vi "PrefDialog-2.vi"(8 "error in (no error)":errorcluster, 11 "MyPluginsBase in":refnum<class "NHRGridSim.lvclass">) -> (0 "error out":errorcluster, 1 "Save As":bool, 2 "Changed":bool, 3 "MyPluginsBase out":refnum<class "NHRGridSim.lvclass">)   [LabVIEW 2018, in "AcPwrPlugins.lvlib" / "NHRGridSim.lvclass"]
doc: "This VI opens up the modal preference dialog window and allows a user to configure the properties with new values, or keep the existing values from the last time the function was called. The user can also save the new values to a new file name and new type name using the save as button."
uses:
  NHRGridSim.lvclass
  C:/Program Files (x86)/National Instruments/LabVIEW 2018/user.lib/NIST/BaseClasses/BasePlugin_class/BasePlugin.lvclass
  C:/Users/Public/Projects/ICDAS/NistPluggableModules/AcPwr/AcPwrPlugins/AcPwrBaseClass/AcPwrBase.lvclass
  PublicMethods/Measurements.ctl
  TypeDefs/MeasurementType.ctl
  TypeDefs/NHRGrid_Modes.ctl
  TypeDefs/Device(s)Settings.ctl
  TypeDefs/NHRGrid_InstrumentCluster_Tabs.ctl
  TypeDefs/NHRGrid_Configure_Tabs.ctl
  TypeDefs/NHRGrid_Ranges_Tabs.ctl
  TypeDefs/NHRGrid_SafetyTrips_Tabs.ctl
  TypeDefs/NHRGrid_SlewRates_Tabs.ctl
  TypeDefs/NHRGrid_Phases_Tabs.ctl
  <userlib>/NIST/BaseClasses/BasePlugin_class/BasePlugin.lvclass/BasePlugin.ctl
  AcPwrBaseClass/AcPwrBase.lvclass/AcPwrBase.ctl
  TypeDefs/NHRGrid_UpdateSettings.ctl
  TypeDefs/NHRGrid_ModeAdjust_Tabs.ctl
  <userlib>/NIST/BaseClasses/BasePlugin_class/Accessors/Read PluginIniFilePath.vi
  AcPwrBaseClass/Accessors/Read BaseConfig.vi
  AcPwrBaseClass/Accessors/Read BaseMeasurements.vi
  <userlib>/NIST/BaseClasses/BasePlugin_class/Accessors/Write PluginIniFilePath.vi
  <vilib>/Utility/config.llb/NI_LVConfig.lvlib
panel:
  in  "ModeVal":u8
  in  "ChassisTxt":string
  in  "Update":bool
  in  "Device(s)Settings":T1={"MeasName"="", "Instr1"={"Name"="", "Vout (V)"=0.0, "VType"="", "FreqOut (Hz)"=60.0, "Aperture (cycles)"=1, "Synchronization"=0, "Ranges"={"Voltage (V)"=0, "Current (A)"=1}, "Safety Trips"={"Vmin (V)"=0.0, "Vmin Time (s)"=-1.0, "Vmax (V)"=0.0, "Vmax Time (s)"=-1.0, "Imax Source (A)"=0.0, "I Src Time (s)"=-1.0, "Imax Sink (A)"=0.0, "I Snk Time (s)"=-1.0, "Pmax Source (W)"=0.0, "P Src Time (s)"=-1.0, "Pmax Sink (W)"=0.0, "P Snk Time (s)"=-1.0, "Abs Volt Peak"=0.0, "Enable Vpk"=FALSE, "Abs Curr Peak"=0.0, "Enable Ipk"=FALSE}, "Slew Rates"={"Voltage (V/s)"=866030.0, "Current (A/s)"=100000.0, "Power (W/s)"=3000000.0, "Frequency (Hz/s)"=500.0, "Phase Angle (Deg/s)"=50000.0}, "Phases"={"A-Volts (V)"=0.0, "B-Volts (V)"=0.0, "C-Volts (V)"=0.0, "A-Change at..."=0, "B-Angle (Deg)"=240, "C-Angle (Deg)"=120, "B-Change at..."=0, "C-Change at..."=0, "AngleTxt"="", "A-Wave Shape"=0, "B-Wave Shape"=0, "C-Wave Shape"=0}}, "Instr2"={"Name"="", "Vout (V)"=0.0, "VType"="", "FreqOut (Hz)"=60.0, "Aperture (cycles)"=1, "Synchronization"=0, "Ranges"={"Voltage (V)"=0, "Current (A)"=1}, "Safety Trips"={"Vmin (V)"=0.0, "Vmin Time (s)"=-1.0, "Vmax (V)"=0.0, "Vmax Time (s)"=-1.0, "Imax Source (A)"=0.0, "I Src Time (s)"=-1.0, "Imax Sink (A)"=0.0, "I Snk Time (s)"=-1.0, "Pmax Source (W)"=0.0, "P Src Time (s)"=-1.0, "Pmax Sink (W)"=0.0, "P Snk Time (s)"=-1.0, "Abs Volt Peak"=0.0, "Enable Vpk"=FALSE, "Abs Curr Peak"=0.0, "Enable Ipk"=FALSE}, "Slew Rates"={"Voltage (V/s)"=866030.0, "Current (A/s)"=100000.0, "Power (W/s)"=3000000.0, "Frequency (Hz/s)"=500.0, "Phase Angle (Deg/s)"=50000.0}, "Phases"={"A-Volts (V)"=0.0, "B-Volts (V)"=0.0, "C-Volts (V)"=0.0, "A-Change at..."=0, "B-Angle (Deg)"=240, "C-Angle (Deg)"=120, "B-Change at..."=0, "C-Change at..."=0, "AngleTxt"="", "A-Wave Shape"=0, "B-Wave Shape"=0, "C-Wave Shape"=0}}, "Instr3"={"Name"="", "Vout (V)"=0.0, "VType"="", "FreqOut (Hz)"=60.0, "Aperture (cycles)"=1, "Synchronization"=0, "Ranges"={"Voltage (V)"=0, "Current (A)"=1}, "Safety Trips"={"Vmin (V)"=0.0, "Vmin Time (s)"=-1.0, "Vmax (V)"=0.0, "Vmax Time (s)"=-1.0, "Imax Source (A)"=0.0, "I Src Time (s)"=-1.0, "Imax Sink (A)"=0.0, "I Snk Time (s)"=-1.0, "Pmax Source (W)"=0.0, "P Src Time (s)"=-1.0, "Pmax Sink (W)"=0.0, "P Snk Time (s)"=-1.0, "Abs Volt Peak"=0.0, "Enable Vpk"=FALSE, "Abs Curr Peak"=0.0, "Enable Ipk"=FALSE}, "Slew Rates"={"Voltage (V/s)"=866030.0, "Current (A/s)"=100000.0, "Power (W/s)"=3000000.0, "Frequency (Hz/s)"=500.0, "Phase Angle (Deg/s)"=50000.0}, "Phases"={"A-Volts (V)"=0.0, "B-Volts (V)"=0.0, "C-Volts (V)"=0.0, "A-Change at..."=0, "B-Angle (Deg)"=240, "C-Angle (Deg)"=120, "B-Change at..."=0, "C-Change at..."=0, "AngleTxt"="", "A-Wave Shape"=0, "B-Wave Shape"=0, "C-Wave Shape"=0}}, "Handle"="", "Reset"=FALSE, "Mode"=0, "ID Query"=FALSE, "Connected"=FALSE, "Chassis"=1, "VRangeVals1"=[], "SyncList1"=[], "Wave1A"=[], "Wave1B"=[], "Wave1C"=[], "SyncList2"=[], "SyncList3"=[], "VRangeVals3"=[], "VRangeVals2"=[], "CRangeVals1"=[], "CRangeVals3"=[], "CRangeVals2"=[], "TabPages"=[], "Wave2A"=[], "Wave2B"=[], "Wave2C"=[], "Wave3A"=[], "Wave3B"=[], "Wave3C"=[], "EnableCtrls"=[[1, 0, 0, 0, 0, 0, 0, 0, 0, 0, 0, 0, 0, 0, 0, 0, 0, 0], [1, 0, 0, 0, 0, 0, 0, 0, 0, 0, 0, 0, 0, 0, 0, 0, 0, 0], [1, 0, 0, 0, 0, 0, 0, 0, 0, 0, 0, 0, 0, 0, 0, 0, 0, 0]]} {"Chassis" min=1 max=8 step=1; "Mode" items=["3-Phase AC"=0, "AC"=1, "DC"=2, "AC - AC"=7, "AC - DC"=8, "DC - AC"=11, "DC - DC"=12, "2-Phase AC - AC"=5, "2-Phase AC - DC"=6, "AC - AC - AC"=3, "DC - DC - DC"=4, "AC - AC - DC"=9, "AC - DC - DC"=10, "AC - DC - AC"=13, "DC - AC - AC"=14, "DC - AC - DC"=15]; "Instr3"."Phases"."C-Wave Shape" items=["Sine", "User1", "User2", "User3"]; "Instr3"."Phases"."B-Wave Shape" items=["Sine", "User1", "User2", "User3"]; "Instr3"."Phases"."A-Wave Shape" items=["Sine", "User1", "User2", "User3"]; "Instr3"."Phases"."C-Change at..." min=0 max=359; "Instr3"."Phases"."B-Change at..." min=0 max=359; "Instr3"."Phases"."A-Change at..." min=0 max=359; "Instr3"."Phases"."C-Angle (Deg)" min=0 max=359; "Instr3"."Phases"."B-Angle (Deg)" min=0 max=359; "Instr3"."Phases"."C-Volts (V)" min=0.0 max=606.0; "Instr3"."Phases"."B-Volts (V)" min=0.0 max=606.0; "Instr3"."Phases"."A-Volts (V)" min=0.0 max=606.0; "Instr3"."Slew Rates"."Phase Angle (Deg/s)" min=0.1 max=50000.0; "Instr3"."Slew Rates"."Frequency (Hz/s)" min=0.01 max=500.0; "Instr3"."Slew Rates"."Power (W/s)" min=2.0 max=8000000.0; "Instr3"."Slew Rates"."Current (A/s)" min=0.2 max=2400000.0; "Instr3"."Slew Rates"."Voltage (V/s)" min=0.01 max=2000000.0; "Instr3"."Safety Trips"."Abs Curr Peak" min=0.0; "Instr3"."Safety Trips"."Abs Volt Peak" min=0.0; "Instr3"."Safety Trips"."P Snk Time (s)" min=-1.0 max=3600.0; "Instr3"."Safety Trips"."Pmax Sink (W)" min=0.0 max=436000.0 format="%#_7g"; "Instr3"."Safety Trips"."P Src Time (s)" min=-1.0 max=3600.0; "Instr3"."Safety Trips"."Pmax Source (W)" min=0.0 max=436000.0 format="%#_7g"; "Instr3"."Safety Trips"."I Snk Time (s)" min=-1.0 max=3600.0; "Instr3"."Safety Trips"."Imax Sink (A)" min=0.0 max=720.0; "Instr3"."Safety Trips"."I Src Time (s)" min=-1.0 max=3600.0; "Instr3"."Safety Trips"."Imax Source (A)" min=0.0 max=720.0; "Instr3"."Safety Trips"."Vmax Time (s)" min=-1.0 max=3600.0; "Instr3"."Safety Trips"."Vmax (V)" min=0.0 max=606.0; "Instr3"."Safety Trips"."Vmin Time (s)" min=-1.0 max=3600.0; "Instr3"."Safety Trips"."Vmin (V)" min=0.0 max=606.0; "Instr3"."Ranges"."Current (A)" items=["6", "30"]; "Instr3"."Ranges"."Voltage (V)" items=["303", "606"]; "Instr3"."Synchronization" items=["Immediate", "Sync to Phase A"]; "Instr3"."Aperture (cycles)" min=0 max=64; "Instr3"."FreqOut (Hz)" min=30.0 max=880.0; "Instr3"."Vout (V)" min=0.0 max=606.0; "Instr2"."Phases"."C-Wave Shape" items=["Sine", "User1", "User2", "User3"]; "Instr2"."Phases"."B-Wave Shape" items=["Sine", "User1", "User2", "User3"]; "Instr2"."Phases"."A-Wave Shape" items=["Sine", "User1", "User2", "User3"]; "Instr2"."Phases"."C-Change at..." min=0 max=359; "Instr2"."Phases"."B-Change at..." min=0 max=359; "Instr2"."Phases"."A-Change at..." min=0 max=359; "Instr2"."Phases"."C-Angle (Deg)" min=0 max=359; "Instr2"."Phases"."B-Angle (Deg)" min=0 max=359; "Instr2"."Phases"."C-Volts (V)" min=0.0 max=606.0; "Instr2"."Phases"."B-Volts (V)" min=0.0 max=606.0; "Instr2"."Phases"."A-Volts (V)" min=0.0 max=606.0; "Instr2"."Slew Rates"."Phase Angle (Deg/s)" min=0.1 max=50000.0; "Instr2"."Slew Rates"."Frequency (Hz/s)" min=0.01 max=500.0; "Instr2"."Slew Rates"."Power (W/s)" min=2.0 max=8000000.0; "Instr2"."Slew Rates"."Current (A/s)" min=0.2 max=2400000.0; "Instr2"."Slew Rates"."Voltage (V/s)" min=0.01 max=2000000.0; "Instr2"."Safety Trips"."Abs Curr Peak" min=0.0; "Instr2"."Safety Trips"."Abs Volt Peak" min=0.0; "Instr2"."Safety Trips"."P Snk Time (s)" min=-1.0 max=3600.0; "Instr2"."Safety Trips"."Pmax Sink (W)" min=0.0 max=436000.0 format="%#_7g"; "Instr2"."Safety Trips"."P Src Time (s)" min=-1.0 max=3600.0; "Instr2"."Safety Trips"."Pmax Source (W)" min=0.0 max=436000.0 format="%#_7g"; "Instr2"."Safety Trips"."I Snk Time (s)" min=-1.0 max=3600.0; "Instr2"."Safety Trips"."Imax Sink (A)" min=0.0 max=720.0; "Instr2"."Safety Trips"."I Src Time (s)" min=-1.0 max=3600.0; "Instr2"."Safety Trips"."Imax Source (A)" min=0.0 max=720.0; "Instr2"."Safety Trips"."Vmax Time (s)" min=-1.0 max=3600.0; "Instr2"."Safety Trips"."Vmax (V)" min=0.0 max=606.0; "Instr2"."Safety Trips"."Vmin Time (s)" min=-1.0 max=3600.0; "Instr2"."Safety Trips"."Vmin (V)" min=0.0 max=606.0; "Instr2"."Ranges"."Current (A)" items=["6", "30"]; "Instr2"."Ranges"."Voltage (V)" items=["303", "606"]; "Instr2"."Synchronization" items=["Immediate", "Sync to Phase A"]; "Instr2"."Aperture (cycles)" min=0 max=64; "Instr2"."FreqOut (Hz)" min=30.0 max=880.0; "Instr2"."Vout (V)" min=0.0 max=606.0; "Instr1"."Phases"."C-Wave Shape" items=["Sine", "User1", "User2", "User3"]; "Instr1"."Phases"."B-Wave Shape" items=["Sine", "User1", "User2", "User3"]; "Instr1"."Phases"."A-Wave Shape" items=["Sine", "User1", "User2", "User3"]; "Instr1"."Phases"."C-Change at..." min=0 max=359; "Instr1"."Phases"."B-Change at..." min=0 max=359; "Instr1"."Phases"."A-Change at..." min=0 max=359; "Instr1"."Phases"."C-Angle (Deg)" min=0 max=359; "Instr1"."Phases"."B-Angle (Deg)" min=0 max=359; "Instr1"."Phases"."C-Volts (V)" min=0.0 max=606.0; "Instr1"."Phases"."B-Volts (V)" min=0.0 max=606.0; "Instr1"."Phases"."A-Volts (V)" min=0.0 max=606.0; "Instr1"."Slew Rates"."Phase Angle (Deg/s)" min=0.1 max=50000.0; "Instr1"."Slew Rates"."Frequency (Hz/s)" min=0.01 max=500.0; "Instr1"."Slew Rates"."Power (W/s)" min=2.0 max=8000000.0; "Instr1"."Slew Rates"."Current (A/s)" min=0.2 max=2400000.0; "Instr1"."Slew Rates"."Voltage (V/s)" min=0.01 max=2000000.0; "Instr1"."Safety Trips"."Abs Curr Peak" min=0.0; "Instr1"."Safety Trips"."Abs Volt Peak" min=0.0; "Instr1"."Safety Trips"."P Snk Time (s)" min=-1.0 max=3600.0; "Instr1"."Safety Trips"."Pmax Sink (W)" min=0.0 max=436000.0 format="%#_7g"; "Instr1"."Safety Trips"."P Src Time (s)" min=-1.0 max=3600.0; "Instr1"."Safety Trips"."Pmax Source (W)" min=0.0 max=436000.0 format="%#_7g"; "Instr1"."Safety Trips"."I Snk Time (s)" min=-1.0 max=3600.0; "Instr1"."Safety Trips"."Imax Sink (A)" min=0.0 max=720.0; "Instr1"."Safety Trips"."I Src Time (s)" min=-1.0 max=3600.0; "Instr1"."Safety Trips"."Imax Source (A)" min=0.0 max=720.0; "Instr1"."Safety Trips"."Vmax Time (s)" min=-1.0 max=3600.0; "Instr1"."Safety Trips"."Vmax (V)" min=0.0 max=606.0; "Instr1"."Safety Trips"."Vmin Time (s)" min=-1.0 max=3600.0; "Instr1"."Safety Trips"."Vmin (V)" min=0.0 max=606.0; "Instr1"."Ranges"."Current (A)" items=["6", "30"]; "Instr1"."Ranges"."Voltage (V)" items=["303", "606"]; "Instr1"."Synchronization" items=["Immediate", "Sync to Phase A"]; "Instr1"."Aperture (cycles)" min=0 max=64; "Instr1"."FreqOut (Hz)" min=30.0 max=880.0; "Instr1"."Vout (V)" min=0.0 max=606.0}
  in  "Chassis":i32=1 min=1 max=8 step=1
  in  "MeasName":string
  out "Connected":bool
  in  "ID Query":bool
  in  "Mode":T8 items=["3-Phase AC"=0, "AC"=1, "DC"=2, "AC - AC"=7, "AC - DC"=8, "DC - AC"=11, "DC - DC"=12, "2-Phase AC - AC"=5, "2-Phase AC - DC"=6, "AC - AC - AC"=3, "DC - DC - DC"=4, "AC - AC - DC"=9, "AC - DC - DC"=10, "AC - DC - AC"=13, "DC - AC - AC"=14, "DC - AC - DC"=15]
  in  "Reset":bool
  in  "Handle":string
  in  "Instruments":enum32{"Page 1", "Page 2", "Page 3"}(tab)
  in  "Instr1":T2={"Name"="", "Vout (V)"=0.0, "VType"="", "FreqOut (Hz)"=60.0, "Aperture (cycles)"=1, "Synchronization"=0, "Ranges"={"Voltage (V)"=0, "Current (A)"=1}, "Safety Trips"={"Vmin (V)"=0.0, "Vmin Time (s)"=-1.0, "Vmax (V)"=0.0, "Vmax Time (s)"=-1.0, "Imax Source (A)"=0.0, "I Src Time (s)"=-1.0, "Imax Sink (A)"=0.0, "I Snk Time (s)"=-1.0, "Pmax Source (W)"=0.0, "P Src Time (s)"=-1.0, "Pmax Sink (W)"=0.0, "P Snk Time (s)"=-1.0, "Abs Volt Peak"=0.0, "Enable Vpk"=FALSE, "Abs Curr Peak"=0.0, "Enable Ipk"=FALSE}, "Slew Rates"={"Voltage (V/s)"=866030.0, "Current (A/s)"=100000.0, "Power (W/s)"=3000000.0, "Frequency (Hz/s)"=500.0, "Phase Angle (Deg/s)"=50000.0}, "Phases"={"A-Volts (V)"=0.0, "B-Volts (V)"=0.0, "C-Volts (V)"=0.0, "A-Change at..."=0, "B-Angle (Deg)"=240, "C-Angle (Deg)"=120, "B-Change at..."=0, "C-Change at..."=0, "AngleTxt"="", "A-Wave Shape"=0, "B-Wave Shape"=0, "C-Wave Shape"=0}} {"Phases"."C-Wave Shape" items=["Sine", "User1", "User2", "User3"]; "Phases"."B-Wave Shape" items=["Sine", "User1", "User2", "User3"]; "Phases"."A-Wave Shape" items=["Sine", "User1", "User2", "User3"]; "Phases"."C-Change at..." min=0 max=359; "Phases"."B-Change at..." min=0 max=359; "Phases"."A-Change at..." min=0 max=359; "Phases"."C-Angle (Deg)" min=0 max=359; "Phases"."B-Angle (Deg)" min=0 max=359; "Phases"."C-Volts (V)" min=0.0 max=606.0; "Phases"."B-Volts (V)" min=0.0 max=606.0; "Phases"."A-Volts (V)" min=0.0 max=606.0; "Slew Rates"."Phase Angle (Deg/s)" min=0.1 max=50000.0; "Slew Rates"."Frequency (Hz/s)" min=0.01 max=500.0; "Slew Rates"."Power (W/s)" min=2.0 max=8000000.0; "Slew Rates"."Current (A/s)" min=0.2 max=2400000.0; "Slew Rates"."Voltage (V/s)" min=0.01 max=2000000.0; "Safety Trips"."Abs Curr Peak" min=0.0; "Safety Trips"."Abs Volt Peak" min=0.0; "Safety Trips"."P Snk Time (s)" min=-1.0 max=3600.0; "Safety Trips"."Pmax Sink (W)" min=0.0 max=436000.0 format="%#_7g"; "Safety Trips"."P Src Time (s)" min=-1.0 max=3600.0; "Safety Trips"."Pmax Source (W)" min=0.0 max=436000.0 format="%#_7g"; "Safety Trips"."I Snk Time (s)" min=-1.0 max=3600.0; "Safety Trips"."Imax Sink (A)" min=0.0 max=720.0; "Safety Trips"."I Src Time (s)" min=-1.0 max=3600.0; "Safety Trips"."Imax Source (A)" min=0.0 max=720.0; "Safety Trips"."Vmax Time (s)" min=-1.0 max=3600.0; "Safety Trips"."Vmax (V)" min=0.0 max=606.0; "Safety Trips"."Vmin Time (s)" min=-1.0 max=3600.0; "Safety Trips"."Vmin (V)" min=0.0 max=606.0; "Ranges"."Current (A)" items=["6", "30"]; "Ranges"."Voltage (V)" items=["303", "606"]; "Synchronization" items=["Immediate", "Sync to Phase A"]; "Aperture (cycles)" min=0 max=64; "FreqOut (Hz)" min=30.0 max=880.0; "Vout (V)" min=0.0 max=606.0}
  in  "Instr2":T2={"Name"="", "Vout (V)"=0.0, "VType"="", "FreqOut (Hz)"=60.0, "Aperture (cycles)"=1, "Synchronization"=0, "Ranges"={"Voltage (V)"=0, "Current (A)"=1}, "Safety Trips"={"Vmin (V)"=0.0, "Vmin Time (s)"=-1.0, "Vmax (V)"=0.0, "Vmax Time (s)"=-1.0, "Imax Source (A)"=0.0, "I Src Time (s)"=-1.0, "Imax Sink (A)"=0.0, "I Snk Time (s)"=-1.0, "Pmax Source (W)"=0.0, "P Src Time (s)"=-1.0, "Pmax Sink (W)"=0.0, "P Snk Time (s)"=-1.0, "Abs Volt Peak"=0.0, "Enable Vpk"=FALSE, "Abs Curr Peak"=0.0, "Enable Ipk"=FALSE}, "Slew Rates"={"Voltage (V/s)"=866030.0, "Current (A/s)"=100000.0, "Power (W/s)"=3000000.0, "Frequency (Hz/s)"=500.0, "Phase Angle (Deg/s)"=50000.0}, "Phases"={"A-Volts (V)"=0.0, "B-Volts (V)"=0.0, "C-Volts (V)"=0.0, "A-Change at..."=0, "B-Angle (Deg)"=240, "C-Angle (Deg)"=120, "B-Change at..."=0, "C-Change at..."=0, "AngleTxt"="", "A-Wave Shape"=0, "B-Wave Shape"=0, "C-Wave Shape"=0}} {"Phases"."C-Wave Shape" items=["Sine", "User1", "User2", "User3"]; "Phases"."B-Wave Shape" items=["Sine", "User1", "User2", "User3"]; "Phases"."A-Wave Shape" items=["Sine", "User1", "User2", "User3"]; "Phases"."C-Change at..." min=0 max=359; "Phases"."B-Change at..." min=0 max=359; "Phases"."A-Change at..." min=0 max=359; "Phases"."C-Angle (Deg)" min=0 max=359; "Phases"."B-Angle (Deg)" min=0 max=359; "Phases"."C-Volts (V)" min=0.0 max=606.0; "Phases"."B-Volts (V)" min=0.0 max=606.0; "Phases"."A-Volts (V)" min=0.0 max=606.0; "Slew Rates"."Phase Angle (Deg/s)" min=0.1 max=50000.0; "Slew Rates"."Frequency (Hz/s)" min=0.01 max=500.0; "Slew Rates"."Power (W/s)" min=2.0 max=8000000.0; "Slew Rates"."Current (A/s)" min=0.2 max=2400000.0; "Slew Rates"."Voltage (V/s)" min=0.01 max=2000000.0; "Safety Trips"."Abs Curr Peak" min=0.0; "Safety Trips"."Abs Volt Peak" min=0.0; "Safety Trips"."P Snk Time (s)" min=-1.0 max=3600.0; "Safety Trips"."Pmax Sink (W)" min=0.0 max=436000.0 format="%#_7g"; "Safety Trips"."P Src Time (s)" min=-1.0 max=3600.0; "Safety Trips"."Pmax Source (W)" min=0.0 max=436000.0 format="%#_7g"; "Safety Trips"."I Snk Time (s)" min=-1.0 max=3600.0; "Safety Trips"."Imax Sink (A)" min=0.0 max=720.0; "Safety Trips"."I Src Time (s)" min=-1.0 max=3600.0; "Safety Trips"."Imax Source (A)" min=0.0 max=720.0; "Safety Trips"."Vmax Time (s)" min=-1.0 max=3600.0; "Safety Trips"."Vmax (V)" min=0.0 max=606.0; "Safety Trips"."Vmin Time (s)" min=-1.0 max=3600.0; "Safety Trips"."Vmin (V)" min=0.0 max=606.0; "Ranges"."Current (A)" items=["6", "30"]; "Ranges"."Voltage (V)" items=["303", "606"]; "Synchronization" items=["Immediate", "Sync to Phase A"]; "Aperture (cycles)" min=0 max=64; "FreqOut (Hz)" min=30.0 max=880.0; "Vout (V)" min=0.0 max=606.0}
  in  "Instr3":T2={"Name"="", "Vout (V)"=0.0, "VType"="", "FreqOut (Hz)"=60.0, "Aperture (cycles)"=1, "Synchronization"=0, "Ranges"={"Voltage (V)"=0, "Current (A)"=1}, "Safety Trips"={"Vmin (V)"=0.0, "Vmin Time (s)"=-1.0, "Vmax (V)"=0.0, "Vmax Time (s)"=-1.0, "Imax Source (A)"=0.0, "I Src Time (s)"=-1.0, "Imax Sink (A)"=0.0, "I Snk Time (s)"=-1.0, "Pmax Source (W)"=0.0, "P Src Time (s)"=-1.0, "Pmax Sink (W)"=0.0, "P Snk Time (s)"=-1.0, "Abs Volt Peak"=0.0, "Enable Vpk"=FALSE, "Abs Curr Peak"=0.0, "Enable Ipk"=FALSE}, "Slew Rates"={"Voltage (V/s)"=866030.0, "Current (A/s)"=100000.0, "Power (W/s)"=3000000.0, "Frequency (Hz/s)"=500.0, "Phase Angle (Deg/s)"=50000.0}, "Phases"={"A-Volts (V)"=0.0, "B-Volts (V)"=0.0, "C-Volts (V)"=0.0, "A-Change at..."=0, "B-Angle (Deg)"=240, "C-Angle (Deg)"=120, "B-Change at..."=0, "C-Change at..."=0, "AngleTxt"="", "A-Wave Shape"=0, "B-Wave Shape"=0, "C-Wave Shape"=0}} {"Phases"."C-Wave Shape" items=["Sine", "User1", "User2", "User3"]; "Phases"."B-Wave Shape" items=["Sine", "User1", "User2", "User3"]; "Phases"."A-Wave Shape" items=["Sine", "User1", "User2", "User3"]; "Phases"."C-Change at..." min=0 max=359; "Phases"."B-Change at..." min=0 max=359; "Phases"."A-Change at..." min=0 max=359; "Phases"."C-Angle (Deg)" min=0 max=359; "Phases"."B-Angle (Deg)" min=0 max=359; "Phases"."C-Volts (V)" min=0.0 max=606.0; "Phases"."B-Volts (V)" min=0.0 max=606.0; "Phases"."A-Volts (V)" min=0.0 max=606.0; "Slew Rates"."Phase Angle (Deg/s)" min=0.1 max=50000.0; "Slew Rates"."Frequency (Hz/s)" min=0.01 max=500.0; "Slew Rates"."Power (W/s)" min=2.0 max=8000000.0; "Slew Rates"."Current (A/s)" min=0.2 max=2400000.0; "Slew Rates"."Voltage (V/s)" min=0.01 max=2000000.0; "Safety Trips"."Abs Curr Peak" min=0.0; "Safety Trips"."Abs Volt Peak" min=0.0; "Safety Trips"."P Snk Time (s)" min=-1.0 max=3600.0; "Safety Trips"."Pmax Sink (W)" min=0.0 max=436000.0 format="%#_7g"; "Safety Trips"."P Src Time (s)" min=-1.0 max=3600.0; "Safety Trips"."Pmax Source (W)" min=0.0 max=436000.0 format="%#_7g"; "Safety Trips"."I Snk Time (s)" min=-1.0 max=3600.0; "Safety Trips"."Imax Sink (A)" min=0.0 max=720.0; "Safety Trips"."I Src Time (s)" min=-1.0 max=3600.0; "Safety Trips"."Imax Source (A)" min=0.0 max=720.0; "Safety Trips"."Vmax Time (s)" min=-1.0 max=3600.0; "Safety Trips"."Vmax (V)" min=0.0 max=606.0; "Safety Trips"."Vmin Time (s)" min=-1.0 max=3600.0; "Safety Trips"."Vmin (V)" min=0.0 max=606.0; "Ranges"."Current (A)" items=["6", "30"]; "Ranges"."Voltage (V)" items=["303", "606"]; "Synchronization" items=["Immediate", "Sync to Phase A"]; "Aperture (cycles)" min=0 max=64; "FreqOut (Hz)" min=30.0 max=880.0; "Vout (V)" min=0.0 max=606.0}
  in  "Measurements":T9 {"Instrument Number" items=["1", "2", "3"]}
  in  "btnSaveAs":bool
  in  "Measurement RefreshTime (ms)":u32
  in  "btnSave":bool
  in  "btnCancel":bool
  # "@ 12 kW each"
  # "Row = Instrument\nColumn: 0-Name, 1-FreqOut, 2-Sync, 3-AVolts, 4-BVolts, 5-CVolts, 6-BAngle, 7-CAngle, 8-AChange, 9-BChange, 10-CChange, 11-AWave, 12-BWave, 13-CWave, 14-SlewCurr, 15-SlewPower, 16-SlewFreq, 17-SlewPhase"
  # "0= Enabled, 1= Disabled, 2= Disabled and Greyed"
  # "Degrees with Respect to Phase A"
  # "Voltages (L-N)"
  # "Degrees for Synchronization"
  # "AC Phase Waveform"
  # "Degrees with Respect to Phase A"
  # "Voltages (L-N)"
  # "Degrees for Synchronization"
  # "AC Phase Waveform"
  # "Degrees with Respect to Phase A"
  # "Voltages (L-N)"
  # "Degrees for Synchronization"
  # "AC Phase Waveform"
  # "Degrees with Respect to Phase A"
  # "Voltages (L-N)"
  # "Degrees for Synchronization"
  # "AC Phase Waveform"
  # "Degrees with Respect to Phase A"
  # "Voltages (L-N)"
  # "Degrees for Synchronization"
  # "AC Phase Waveform"
  # "Degrees with Respect to Phase A"
  # "Voltages (L-N)"
  # "Degrees for Synchronization"
  # "AC Phase Waveform"
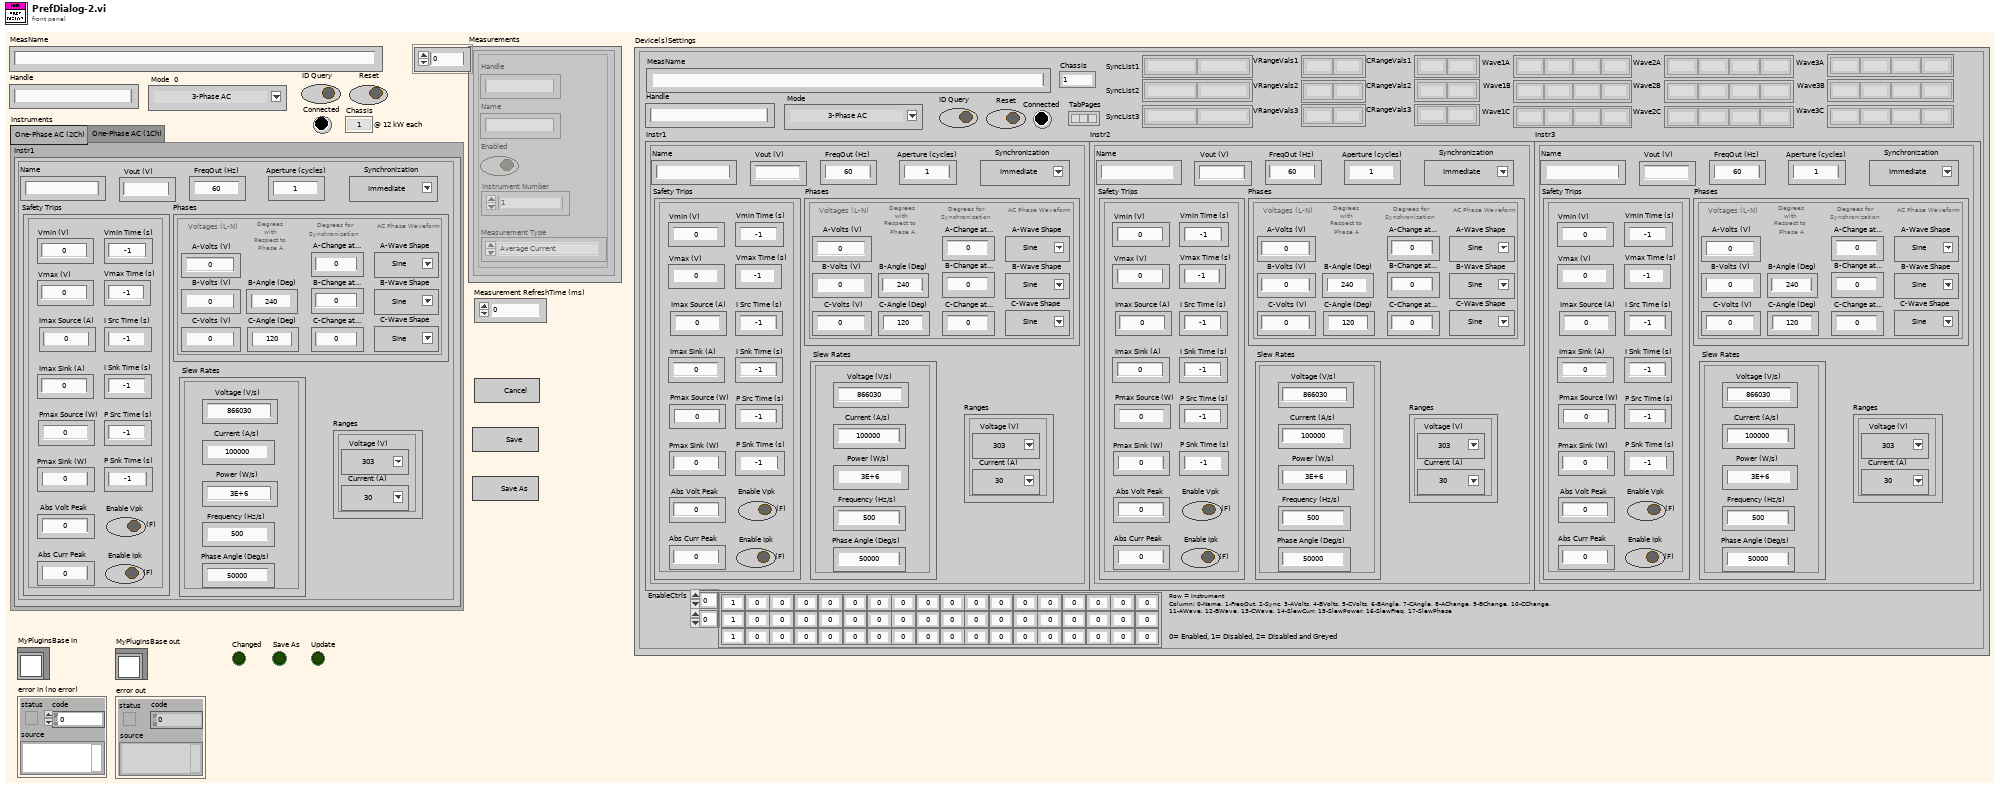
[diagram p1: front panel]
types:
  T1 = typedef "AcPwrPlugins.lvlib/NHRGridSim.lvclass/Device(s)Settings.ctl" = cluster{"MeasName":string, "Instr1":T2, "Instr2":T2, "Instr3":T2, "Handle":string, "Reset":bool, "Mode":T8, "ID Query":bool, "Connected":bool, "Chassis":i32, "VRangeVals1":string[], "SyncList1":string[], "Wave1A":string[], "Wave1B":string[], "Wave1C":string[], "SyncList2":string[], "SyncList3":string[], "VRangeVals3":string[], "VRangeVals2":string[], "CRangeVals1":string[], "CRangeVals3":string[], "CRangeVals2":string[], "TabPages":bool[], "Wave2A":string[], "Wave2B":string[], "Wave2C":string[], "Wave3A":string[], "Wave3B":string[], "Wave3C":string[], "EnableCtrls":i8[][]}
  T2 = typedef "AcPwrPlugins.lvlib/NHRGridSim.lvclass/NHRGrid_InstrumentCluster_Tabs.ctl" = cluster{"Name":string, "Vout (V)":dbl, "VType":string, "FreqOut (Hz)":dbl, "Aperture (cycles)":i32, "Synchronization":T3, "Ranges":T4, "Safety Trips":T5, "Slew Rates":T6, "Phases":T7}
  T3 = typedef "AcPwrPlugins.lvlib/NHRGridSim.lvclass/NHRGrid_Configure_Tabs.ctl" = u16
  T4 = typedef "AcPwrPlugins.lvlib/NHRGridSim.lvclass/NHRGrid_Ranges_Tabs.ctl" = cluster{"Voltage (V)":u16, "Current (A)":u16}
  T5 = typedef "AcPwrPlugins.lvlib/NHRGridSim.lvclass/NHRGrid_SafetyTrips_Tabs.ctl" = cluster{"Vmin (V)":dbl, "Vmin Time (s)":dbl, "Vmax (V)":dbl, "Vmax Time (s)":dbl, "Imax Source (A)":dbl, "I Src Time (s)":dbl, "Imax Sink (A)":dbl, "I Snk Time (s)":dbl, "Pmax Source (W)":dbl, "P Src Time (s)":dbl, "Pmax Sink (W)":dbl, "P Snk Time (s)":dbl, "Abs Volt Peak":dbl, "Enable Vpk":bool, "Abs Curr Peak":dbl, "Enable Ipk":bool}
  T6 = typedef "AcPwrPlugins.lvlib/NHRGridSim.lvclass/NHRGrid_SlewRates_Tabs.ctl" = cluster{"Voltage (V/s)":dbl, "Current (A/s)":dbl, "Power (W/s)":dbl, "Frequency (Hz/s)":dbl, "Phase Angle (Deg/s)":dbl}
  T7 = typedef "AcPwrPlugins.lvlib/NHRGridSim.lvclass/NHRGrid_Phases_Tabs.ctl" = cluster{"A-Volts (V)":dbl, "B-Volts (V)":dbl, "C-Volts (V)":dbl, "A-Change at...":i32, "B-Angle (Deg)":i32, "C-Angle (Deg)":i32, "B-Change at...":i32, "C-Change at...":i32, "AngleTxt":string, "A-Wave Shape":u16, "B-Wave Shape":u16, "C-Wave Shape":u16}
  T8 = typedef "AcPwrPlugins.lvlib/NHRGridSim.lvclass/NHRGrid_Modes.ctl" = u8
  T9 = typedef "AcPwrPlugins.lvlib/NHRGridSim.lvclass/Measurements.ctl" = cluster{"Handle":string, "Name":string, "Enabled ":bool, "Measurement Value":dbl, "Instrument Number ":i32, "Measurement Type ":T10}[]
  T10 = typedef "AcPwrPlugins.lvlib/NHRGridSim.lvclass/MeasurementType.ctl" = enum16{"Average Current", "Average Voltage"}
  T11 = enum32{"Invalid", "Default", "Floating", "Floating/Auto-Hide", "Modal"}
  T12 = enum32{"Invalid", "Standard", "Closed", "Hidden", "Minimized", "Maximized"}
  T13 = typedef "AcPwrPlugins.lvlib/NHRGridSim.lvclass/NHRGrid_UpdateSettings.ctl" = enum16{"VRanges", "CRanges", "Syncs", "Waves", "Load", "Tabs", "Values", "Waves1", "Waves2", "Waves3", "EnableNames", "EnableFreq", "EnableSync", "EnableVoltsA", "EnableVoltsB", "EnableVoltsC", "EnablePhaseB", "EnablePhaseC", "EnableChangeA", "EnableChangeB", "EnableChangeC", "EnableWavesA", "EnableWavesB", "EnableWavesC", "EnableCurrSlew", "EnablePowSlew", "EnableFreqSlew", "EnablePhaseSlew", "SaveEnables1", "SaveEnables2", "SaveEnables3", "SaveEnables4", "SaveEnables5", "SaveEnables6", "Array"}
  T14 = typedef "AcPwrPlugins.lvlib/NHRGridSim.lvclass/NHRGrid_ModeAdjust_Tabs.ctl" = enum16{"ShowTabs", "InstrNames", "VoltRanges", "ConfigSync", "Safety", "Phases", "FreqOut", "PhaseEnable", "ChangeEnable", "VoltsEnable", "Vtype", "Description", "CurrRanges", "VoutCoerce", "VSlewCoerce", "CSlewCoerce", "PSlewCoerce", "F&PhCoerce", "--- Available ---", "TripTCoerce1", "TripTCoerce2", "TripTCoerce3", "VPhaseCoerce", "WaveLists", "SetMode", "SetAperture", "Set V Slew", "Set I Slew", "Set F Slew", "Set P Slew", "Set Ang Slew", "SetVout", "WaveEnable", "SyncEnable", "SlewsCurr", "SlewsPow", "SlewsFreq", "SlewsPhase"}
  T15 = enum8{"Enabled", "Disabled", "Disabled and Grayed Out"}
  T16 = typedef "AcPwrPlugins.lvlib/AcPwrBase.lvclass/BaseConfig.ctl" = cluster{"Frequency":dbl, "FrequencyRange":dbl[], "Phases":T17[], "Name":string, "PluginConfigVariant":variant, "PluginMeasVariant":variant}
  T17 = typedef "AcPwrPlugins.lvlib/AcPwrBase.lvclass/Phase.ctl" = cluster{"Name":string, "Enabled":bool, "VoltageLevel":dbl, "Handle":string, "VoltageRange":dbl[], "Connected":bool, "CurrentLimit":dbl, "Waveform":string}
  T18 = typedef "AcPwrPlugins.lvlib/AcPwrBase.lvclass/BaseMeasurements.ctl" = cluster{"Handle":string, "Name":string, "Enabled":bool, "Measurement Value":dbl, "btnMeasFetch":bool, "Chroma Hold Peak Current Measurement":bool, "Chroma Measurement Type":T19, "Chroma Protection Status String":string, "NHRDC Fetch Method":i32, "NHRDC Fetch Time (s)":sgl, "NHRDC Measurement Type":i32, "NHRGridSim Measurement Type ":enum16{"Average Current", "Max Current", "Min Current", "Average Voltage", "Max Voltage", "Min Voltage", "Average True Power", "Max True Power", "Min True Power", "Average Apparent Power", "Max Apparent Power", "Min Apparent Power", "Power Factor", "Crest Factor"}, "NHRGridSim Phase ":i32, "PPS Measurement Type ":enum16{"Voltage RMS L-N", "Voltage RMS L-L", "Frequency", "Current RMS", "Current Peak", "Crest Factor", "Power Factor", "Power VA", "Real Power"}, "PPS Channel Name":enum16{"A", "B", "C"}}[]
  T19 = typedef "AcPwrPlugins.lvlib/ChromaAcLoad.lvclass/MeasurementType.ctl" = enum16{"Voltage (Vrms or V)", "Current (Arms or A)", "Power (W)", "Peak Voltage (V)", "Peak Current (A)", "Peak Power (W)", "Frequency (Hz)", "Resistance (Ohms)", "Voltage Overshoot (V)", "Positive Peak Current (A)", "Voltage Undershoot (V)", "Negative Peak Current (A)", "Apparent Power (VA)", "Reacitive Power (VAR)", "Voltage THD", "Power Factor", "Current's Crest Factor"}
  T20 = typedef "NI_LVConfig.lvlib/Config Data RefNum.ctl" = refnum<k1>
  T21 = enum8{"Enabled", "Disabled", "Disabled and Grayed Out"}[]
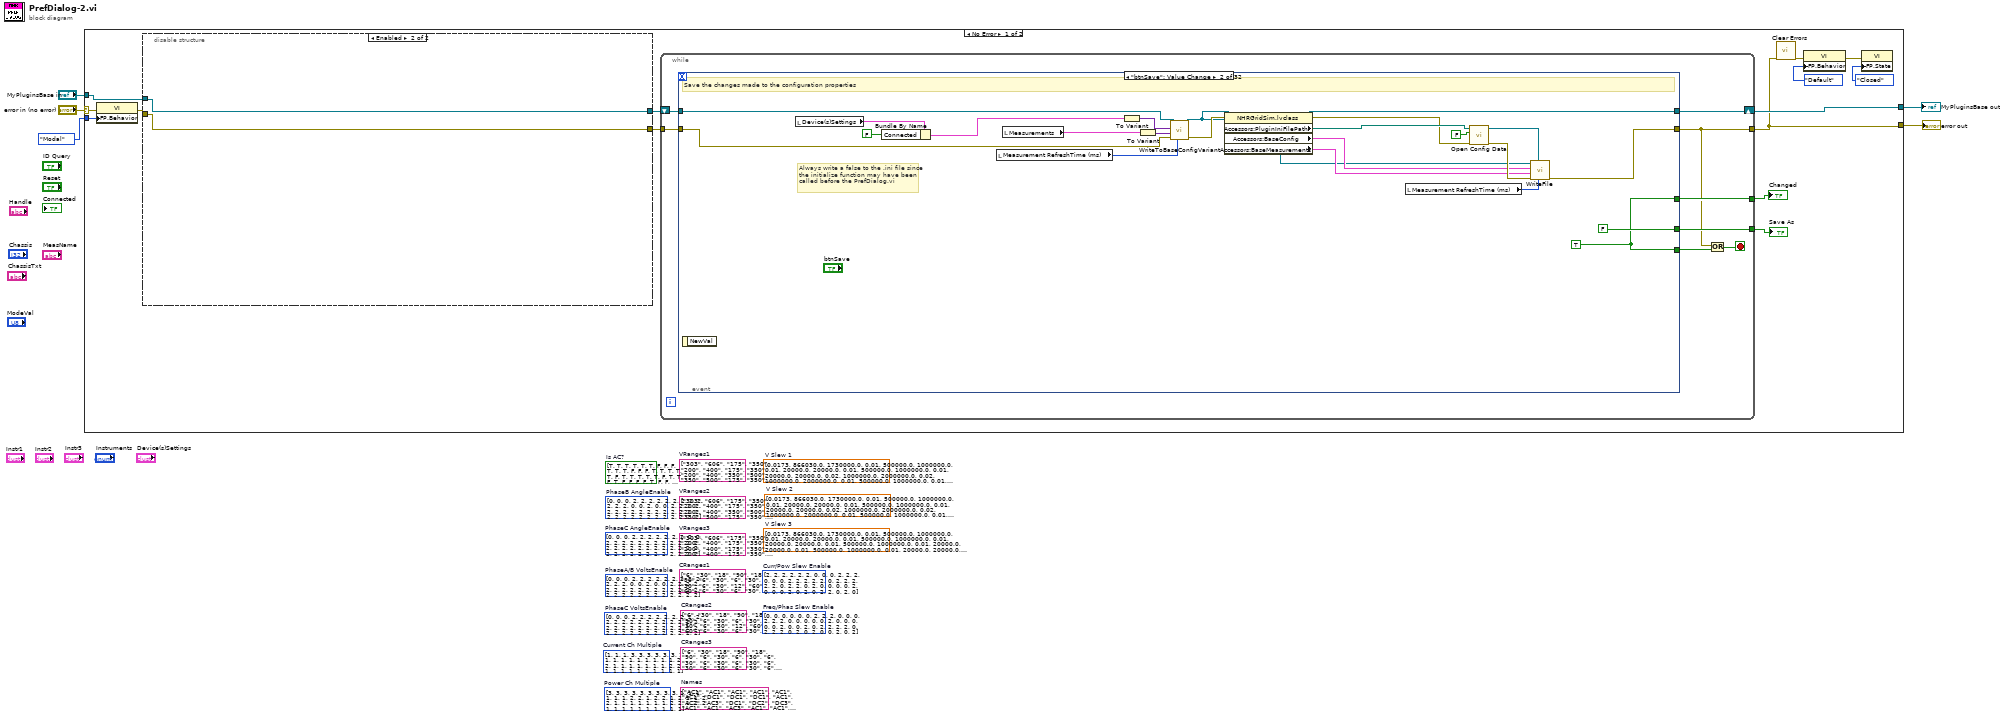
[diagram p0: block diagram]
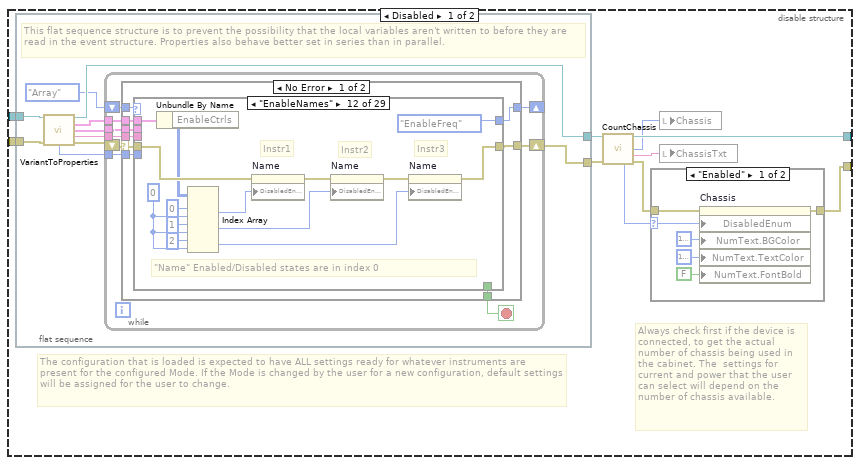
[diagram p2: hidden frame]
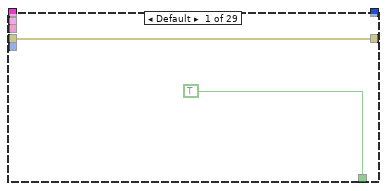
[diagram p3: hidden frame]
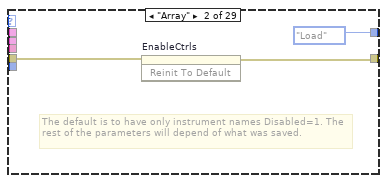
[diagram p4: hidden frame]
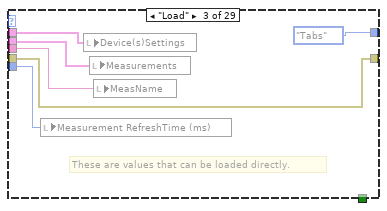
[diagram p5: hidden frame]
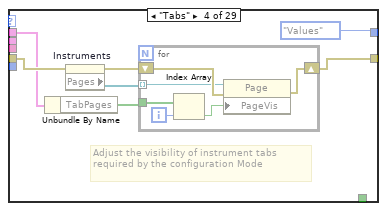
[diagram p6: hidden frame]
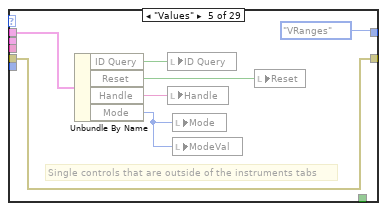
[diagram p7: hidden frame]
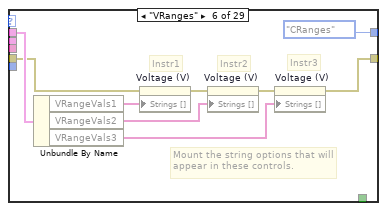
[diagram p8: hidden frame]
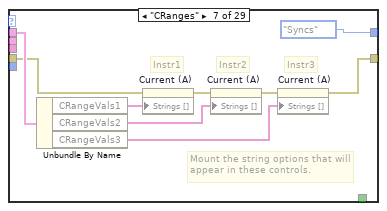
[diagram p9: hidden frame]
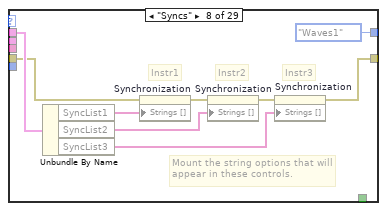
[diagram p10: hidden frame]
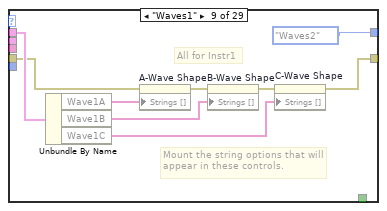
[diagram p11: hidden frame]
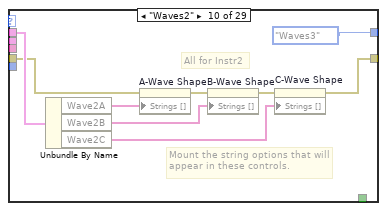
[diagram p12: hidden frame]
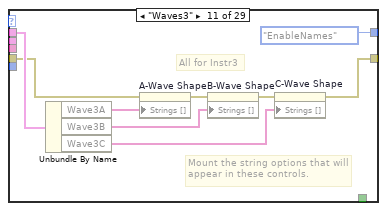
[diagram p13: hidden frame]
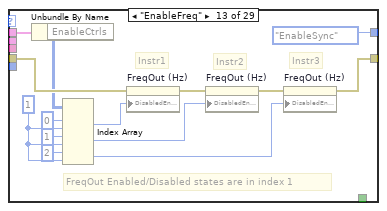
[diagram p14: hidden frame]
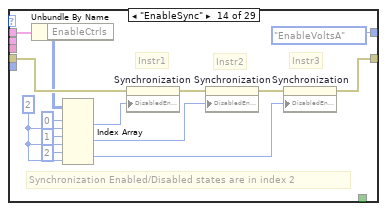
[diagram p15: hidden frame]
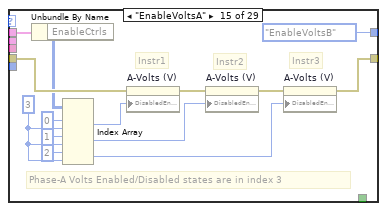
[diagram p16: hidden frame]
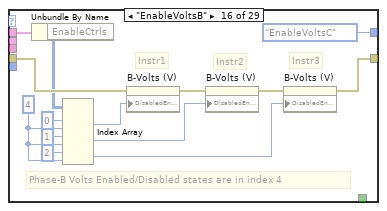
[diagram p17: hidden frame]
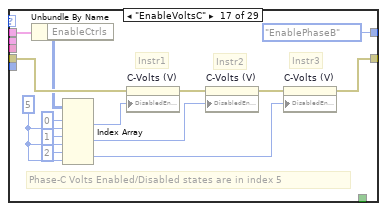
[diagram p18: hidden frame]
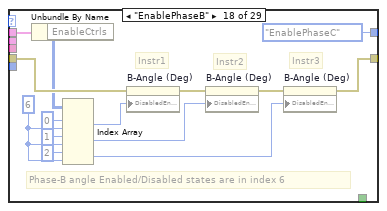
[diagram p19: hidden frame]
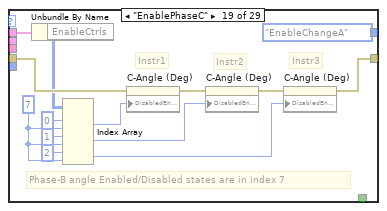
[diagram p20: hidden frame]
diagram:
  (unwired) i32[][] [[3, 3, 3], [3, 3, 3], [3, 3, 3], [1, 1, 1], [1, 1, 1], [2, 2, 1], [2, 2, 1], [2, 2, 1], [2, 2, 1], [1, 1, 1], [1, 1, 1], [2, 2, 1], [2, 2, 1], [1, 1, 1], [1, 1, 1], [1, 1, 1]]  # Power Ch Multiple
  (unwired) i8[][] [[0, 0, 0], [0, 0, 0], [2, 2, 2], [0, 0, 0], [2, 2, 2], [0, 0, 0], [0, 0, 2], [0, 0, 0], [0, 0, 2], [0, 0, 2], [0, 2, 2], [2, 2, 0], [2, 2, 2], [0, 2, 0], [2, 0, 0], [2, 0, 2]]  # Freq/Phas Slew Enable
  (unwired) i8[][] [[2, 2, 2], [2, 2, 2], [0, 0, 0], [2, 2, 2], [0, 0, 0], [2, 2, 2], [2, 2, 0], [2, 2, 2], [2, 2, 0], [2, 2, 0], [2, 0, 0], [0, 0, 2], [0, 0, 0], [2, 0, 2], [0, 2, 2], [0, 2, 0]]  # Curr/Pow Slew Enable
  (unwired) i32[][] [[1, 1, 1], [3, 3, 3], [3, 3, 3], [1, 1, 1], [1, 1, 1], [1, 1, 1], [1, 1, 1], [2, 2, 1], [2, 2, 1], [1, 1, 1], [1, 1, 1], [2, 2, 1], [2, 2, 1], [1, 1, 1], [1, 1, 1], [1, 1, 1]]  # Current Ch Multiple
  (unwired) dbl[][] [[0.0173, 866030.0, 1730000.0], [0.01, 500000.0, 1000000.0], [0.01, 20000.0, 20000.0], [0.01, 500000.0, 1000000.0], [0.01, 20000.0, 20000.0], [0.01, 500000.0, 1000000.0], [0.01, 20000.0, 20000.0], [0.01, 500000.0, 1000000.0], [0.01, 20000.0, 20000.0], [0.01, 20000.0, 20000.0], [0.01, 20000.0, 20000.0], [0.01, 500000.0, 1000000.0], [0.01, 20000.0, 20000.0], [0.01, 500000.0, 1000000.0], [0.01, 500000.0, 1000000.0], [0.01, 20000.0, 20000.0]]  # V Slew 3
  (unwired) dbl[][] [[0.0173, 866030.0, 1730000.0], [0.01, 500000.0, 1000000.0], [0.01, 20000.0, 20000.0], [0.01, 500000.0, 1000000.0], [0.01, 20000.0, 20000.0], [0.02, 1000000.0, 2000000.0], [0.02, 1000000.0, 2000000.0], [0.01, 500000.0, 1000000.0], [0.01, 500000.0, 1000000.0], [0.01, 500000.0, 1000000.0], [0.01, 20000.0, 20000.0], [0.01, 20000.0, 20000.0], [0.01, 20000.0, 20000.0], [0.01, 20000.0, 20000.0], [0.01, 500000.0, 1000000.0], [0.01, 500000.0, 1000000.0]]  # V Slew 2
  (unwired) dbl[][] [[0.0173, 866030.0, 1730000.0], [0.01, 500000.0, 1000000.0], [0.01, 20000.0, 20000.0], [0.01, 500000.0, 1000000.0], [0.01, 20000.0, 20000.0], [0.02, 1000000.0, 2000000.0], [0.02, 1000000.0, 2000000.0], [0.01, 500000.0, 1000000.0], [0.01, 500000.0, 1000000.0], [0.01, 500000.0, 1000000.0], [0.01, 500000.0, 1000000.0], [0.01, 20000.0, 20000.0], [0.01, 20000.0, 20000.0], [0.01, 500000.0, 1000000.0], [0.01, 20000.0, 20000.0], [0.01, 20000.0, 20000.0]]  # V Slew 1
  (unwired) i8[][] [[0, 0, 0], [2, 2, 2], [2, 2, 2], [2, 2, 2], [2, 2, 2], [0, 0, 2], [0, 0, 2], [2, 2, 2], [2, 2, 2], [2, 2, 2], [2, 2, 2], [2, 2, 2], [2, 2, 2], [2, 2, 2], [2, 2, 2], [2, 2, 2]]  # PhaseA/B VoltsEnable
  (unwired) i8[][] [[0, 0, 0], [2, 2, 2], [2, 2, 2], [2, 2, 2], [2, 2, 2], [2, 2, 2], [2, 2, 2], [2, 2, 2], [2, 2, 2], [2, 2, 2], [2, 2, 2], [2, 2, 2], [2, 2, 2], [2, 2, 2], [2, 2, 2], [2, 2, 2]]  # PhaseC VoltsEnable
  (unwired) i8[][] [[0, 0, 0], [2, 2, 2], [2, 2, 2], [2, 2, 2], [2, 2, 2], [2, 2, 2], [2, 2, 2], [2, 2, 2], [2, 2, 2], [2, 2, 2], [2, 2, 2], [2, 2, 2], [2, 2, 2], [2, 2, 2], [2, 2, 2], [2, 2, 2]]  # PhaseC AngleEnable
  (unwired) i8[][] [[0, 0, 0], [2, 2, 2], [2, 2, 2], [2, 2, 2], [2, 2, 2], [0, 0, 2], [0, 0, 2], [2, 2, 2], [2, 2, 2], [2, 2, 2], [2, 2, 2], [2, 2, 2], [2, 2, 2], [2, 2, 2], [2, 2, 2], [2, 2, 2]]  # PhaseB AngleEnable
  (unwired) string[][] [["6", "30"], ["18", "90"], ["18", "90"], ["6", "30"], ["6", "30"], ["6", "30"], ["6", "30"], ["6", "30"], ["6", "30"], ["6", "30"], ["6", "30"], ["6", "30"], ["6", "30"], ["6", "30"], ["6", "30"], ["6", "30"]]  # CRanges3
  (unwired) string[][] [["6", "30"], ["18", "90"], ["18", "90"], ["6", "30"], ["6", "30"], ["6", "30"], ["6", "30"], ["12", "60"], ["12", "60"], ["6", "30"], ["6", "30"], ["12", "60"], ["12", "60"], ["6", "30"], ["6", "30"], ["6", "30"]]  # CRanges2
  (unwired) string[][] [["6", "30"], ["18", "90"], ["18", "90"], ["6", "30"], ["6", "30"], ["6", "30"], ["6", "30"], ["12", "60"], ["12", "60"], ["6", "30"], ["6", "30"], ["12", "60"], ["12", "60"], ["6", "30"], ["6", "30"], ["6", "30"]]  # CRanges1
  (unwired) string[][] [["AC1", "AC1", "AC1"], ["AC1", "AC1", "AC1"], ["DC1", "DC1", "DC1"], ["AC1", "AC2", "AC3"], ["DC1", "DC2", "DC3"], ["AC1", "AC1", "AC3"], ["AC1", "AC1", "DC3"], ["AC1", "AC1", "AC3"], ["AC1", "AC1", "DC3"], ["AC1", "AC2", "DC3"], ["AC1", "DC2", "DC3"], ["DC1", "DC1", "AC3"], ["DC1", "DC1", "DC3"], ["AC1", "DC2", "AC3"], ["DC1", "AC2", "AC3"], ["DC1", "AC2", "DC3"]]  # Names
  (unwired) string[][] [["303", "606"], ["175", "350"], ["200", "400"], ["175", "350"], ["200", "400"], ["175", "350"], ["200", "400"], ["175", "350"], ["200", "400"], ["200", "400"], ["200", "400"], ["175", "350"], ["200", "400"], ["175", "350"], ["175", "350"], ["200", "400"]]  # VRanges3
  (unwired) string[][] [["303", "606"], ["175", "350"], ["200", "400"], ["175", "350"], ["200", "400"], ["350", "500"], ["350", "500"], ["175", "350"], ["175", "350"], ["175", "350"], ["200", "400"], ["200", "400"], ["200", "400"], ["200", "400"], ["175", "350"], ["175", "350"]]  # VRanges2
  (unwired) string[][] [["303", "606"], ["175", "350"], ["200", "400"], ["175", "350"], ["200", "400"], ["350", "500"], ["350", "500"], ["175", "350"], ["175", "350"], ["175", "350"], ["175", "350"], ["200", "400"], ["200", "400"], ["175", "350"], ["200", "400"], ["200", "400"]]  # VRanges1
  (unwired) bool[][] [[TRUE, TRUE, TRUE], [TRUE, TRUE, TRUE], [FALSE, FALSE, FALSE], [TRUE, TRUE, TRUE], [FALSE, FALSE, FALSE], [TRUE, TRUE, TRUE], [TRUE, TRUE, FALSE], [TRUE, TRUE, TRUE], [TRUE, TRUE, FALSE], [TRUE, TRUE, FALSE], [TRUE, FALSE, FALSE], [FALSE, FALSE, TRUE], [FALSE, FALSE, FALSE], [TRUE, FALSE, TRUE], [FALSE, TRUE, TRUE], [FALSE, TRUE, FALSE]]  # Is AC?
  n1 = case shown="No Error" "error in (no error)" {
    selector: "error in (no error)" -> [w18 w3283]
    tunnel: "MyPluginsBase in" -> [w10 w3282]
    tunnel: [w14 w3282] -> w3
    tunnel: [w9 w3283] -> w2
    tunnel: T11."Modal" ("Front Panel Window:Behavior") -> [w12 _]
    frame No Error {
      n2 = property class="VI"(error in=w18, "FP.Behavior"=w12) -> (error out=w11:errorcluster)  [unwired: 1 in, 1 out]
      n3 = disable-structure shown="Enabled" {
        disable-tunnel: w11 -> [w29 w410]
        disable-tunnel: w10 -> [w28 w411]
        disable-tunnel: [w27 w411] -> w7
        disable-tunnel: [w26 w410] -> w6
        frame Disabled {
          # "The configuration that is loaded is expected to have ALL settings ready for whatever instruments are present for the configured Mode. If the Mode is changed by the user for a new configuration, default settings will be assigned for the user to change."
          # "Always check first if the device is connected, to get the actual number of chassis being used in the cabinet. The  settings for current and power that the user can select will depend on the number of chassis available."
          n4 = flat-sequence {
            tunnel: [w39] -> w25
            tunnel: w29 -> [w38]
            tunnel: w28 -> [w37]
            tunnel: [w31] -> w20
            frame #0 {
              # "This flat sequence structure is to prevent the possibility that the local variables aren't written to before they are read in the event structure. Properties also behave better set in series than in parallel."
              n5 = call "VariantToProperties.vi"("NHRGridSim in"=w37, "error in (no error)"=w38) -> ("NHRGridSim out"=w39:refnum<class "NHRGridSim.lvclass">, "Device(s)Settings"=w36:T1, "Measurements"=w35:T9, "MeasName"=w33:string, "Measurement Refresh Time (ms)"=w34:u32, "error out"=w32:errorcluster)  [unwired: 8 in]
              n6 = while {
                tunnel: w36 -> [w47]
                tunnel: w35 -> [w46]
                tunnel: w34 -> [w45]
                tunnel: w33 -> [w44]
                shift-right: [w42] -> w31
                shift-left: w32 -> [w43]
                shift-right: [w41] -> _
                shift-left: NHRGrid_UpdateSettings."Array" -> [w48]
                stop <- w40 stop-if-true
                n7 = case shown="No Error" w43 {
                  selector: w43 -> [w52 w395]
                  tunnel: w48 -> [w57 w397]
                  tunnel: w47 -> [w56 _]
                  tunnel: w46 -> [w55 _]
                  tunnel: w45 -> [w54 _]
                  tunnel: w44 -> [w53 _]
                  tunnel: [w51 w395] -> w42
                  tunnel: [w50 w397] -> w41
                  tunnel: [w49 TRUE] -> w40
                  frame No Error {
                    n8 = case shown="\"EnableNames\"" w57 {
                      tunnel: w56 -> [_ _ w65 w71 w87 w96 w105 w115 w123 w132 w142 w156 w170 w184 w198 w212 w226 w240 w254 w268 w282 w296 w310 w324 w338 w352 w366 w380 w394]
                      tunnel: w55 -> [_ _ w67 _ _ _ _ _ _ _ _ _ _ _ _ _ _ _ _ _ _ _ _ _ _ _ _ _ _]
                      tunnel: w54 -> [_ _ w68 _ _ _ _ _ _ _ _ _ _ _ _ _ _ _ _ _ _ _ _ _ _ _ _ _ _]
                      tunnel: w53 -> [_ _ w66 _ _ _ _ _ _ _ _ _ _ _ _ _ _ _ _ _ _ _ _ _ _ _ _ _ _]
                      tunnel: w52 -> [w59 w61 w63 w72 w82 w92 w101 w111 w119 w128 w138 w155 w169 w183 w197 w211 w225 w239 w253 w267 w281 w295 w309 w323 w337 w351 w365 w379 w393]
                      tunnel: [_ NHRGrid_UpdateSettings."Load" NHRGrid_UpdateSettings."Tabs" NHRGrid_UpdateSettings."Values" NHRGrid_UpdateSettings."VRanges" NHRGrid_UpdateSettings."CRanges" NHRGrid_UpdateSettings."Syncs" NHRGrid_UpdateSettings."Waves1" NHRGrid_UpdateSettings."Waves2" NHRGrid_UpdateSettings."Waves3" NHRGrid_UpdateSettings."EnableNames" NHRGrid_UpdateSettings."EnableFreq" NHRGrid_UpdateSettings."EnableSync" NHRGrid_UpdateSettings."EnableVoltsA" NHRGrid_UpdateSettings."EnableVoltsB" NHRGrid_UpdateSettings."EnableVoltsC" NHRGrid_UpdateSettings."EnablePhaseB" NHRGrid_UpdateSettings."EnablePhaseC" NHRGrid_UpdateSettings."EnableChangeA" NHRGrid_UpdateSettings."EnableChangeB" NHRGrid_UpdateSettings."EnableChangeC" NHRGrid_UpdateSettings."EnableWavesA" NHRGrid_UpdateSettings."EnableWavesB" NHRGrid_UpdateSettings."EnableWavesC" NHRGrid_UpdateSettings."EnableCurrSlew" NHRGrid_UpdateSettings."EnablePowSlew" NHRGrid_UpdateSettings."EnableFreqSlew" NHRGrid_UpdateSettings."EnablePhaseSlew" _] -> w50
                      tunnel: [w59 w60 w63 w70 w82 w89 w98 w108 w116 w125 w135 w152 w166 w180 w194 w208 w222 w236 w250 w264 w278 w292 w306 w320 w334 w348 w362 w376 w390] -> w51
                      tunnel: [TRUE _ _ _ _ _ _ _ _ _ _ _ _ _ _ _ _ _ _ _ _ _ _ _ _ _ _ _ TRUE] -> w49
                      frame Default {
                      }
                      frame "Array" {
                        # "The default is to have only instrument names Disabled=1. The rest of the parameters will depend of what was saved."
                        n9 = invoke on="EnableCtrls" class="Arr (strict)" method="Reinit To Default"(error in=w61) -> (error out=w60:errorcluster)  [unwired: 2 in, 2 out]
                      }
                      frame "Load" {
                        # "These are values that can be loaded directly."
                        n10 = local write "Measurement RefreshTime (ms)"(w68) -> ()
                        n11 = local write "Device(s)Settings"(w65) -> ()
                        n12 = local write "Measurements"(w67) -> ()
                        n13 = local write "MeasName"(w66) -> ()
                      }
                      frame "Tabs" {
                        # "Adjust the visibility of instrument tabs required by the configuration Mode"
                        n14 = Unbundle By Name(w71) -> ("TabPages"=w75:bool[])
                        n15 = property on="Instruments" class="TabCtl (strict)"(error in=w72) -> (error out=w74:errorcluster, "Pages"=w73:refnum<vi>[])  [unwired: 1 in, 1 out]
                        n16 = for {
                          tunnel: w73 -> [w77] mode=indexing
                          tunnel: w75 -> [w80]
                          shift-right: [w76] -> w70
                          shift-left: w74 -> [w78]
                          i -> [w81]
                          n17 = Index Array(array=w80, index=w81) -> (element=w79:bool)
                          n18 = property class="Page"(reference=w77, error in=w78, "PageVis"=w79) -> (error out=w76:errorcluster)  [unwired: 1 out]
                        }
                      }
                      frame "Values" {
                        # "Single controls that are outside of the instruments tabs"
                        n19 = Unbundle By Name(w87) -> ("ID Query"=w86:bool, "Reset"=w85:bool, "Handle"=w84:string, "Mode"=w83:T8)
                        n20 = local write "ID Query"(w86) -> ()
                        n21 = local write "Handle"(w84) -> ()
                        n22 = local write "Mode"(w83) -> ()
                        n23 = local write "ModeVal"(w83) -> ()
                        n24 = local write "Reset"(w85) -> ()
                      }
                      frame "VRanges" {
                        # "Mount the string options that will appear in these controls."
                        # "Instr3"
                        # "Instr2"
                        # "Instr1"
                        n25 = Unbundle By Name(w96) -> ("VRangeVals1"=w95:string[], "VRangeVals2"=w94:string[], "VRangeVals3"=w93:string[])
                        n26 = property on="Voltage (V)" class="Ring (strict)"(error in=w92, "Strings []"=w95) -> (error out=w91:errorcluster)  [unwired: 1 in, 1 out]
                        n27 = property on="Voltage (V)" class="Ring (strict)"(error in=w91, "Strings []"=w94) -> (error out=w90:errorcluster)  [unwired: 1 in, 1 out]
                        n28 = property on="Voltage (V)" class="Ring (strict)"(error in=w90, "Strings []"=w93) -> (error out=w89:errorcluster)  [unwired: 1 in, 1 out]
                      }
                      frame "CRanges" {
                        # "Mount the string options that will appear in these controls."
                        # "Instr3"
                        # "Instr2"
                        # "Instr1"
                        n29 = Unbundle By Name(w105) -> ("CRangeVals1"=w104:string[], "CRangeVals2"=w103:string[], "CRangeVals3"=w102:string[])
                        n30 = property on="Current (A)" class="Ring (strict)"(error in=w101, "Strings []"=w104) -> (error out=w100:errorcluster)  [unwired: 1 in, 1 out]
                        n31 = property on="Current (A)" class="Ring (strict)"(error in=w100, "Strings []"=w103) -> (error out=w99:errorcluster)  [unwired: 1 in, 1 out]
                        n32 = property on="Current (A)" class="Ring (strict)"(error in=w99, "Strings []"=w102) -> (error out=w98:errorcluster)  [unwired: 1 in, 1 out]
                      }
                      frame "Syncs" {
                        # "Mount the string options that will appear in these controls."
                        # "Instr3"
                        # "Instr2"
                        # "Instr1"
                        n33 = Unbundle By Name(w115) -> ("SyncList1"=w114:string[], "SyncList2"=w113:string[], "SyncList3"=w112:string[])
                        n34 = property on="Synchronization" class="Ring (strict)"(error in=w111, "Strings []"=w114) -> (error out=w110:errorcluster)  [unwired: 1 in, 1 out]
                        n35 = property on="Synchronization" class="Ring (strict)"(error in=w110, "Strings []"=w113) -> (error out=w109:errorcluster)  [unwired: 1 in, 1 out]
                        n36 = property on="Synchronization" class="Ring (strict)"(error in=w109, "Strings []"=w112) -> (error out=w108:errorcluster)  [unwired: 1 in, 1 out]
                      }
                      frame "Waves1" {
                        # "All for Instr1"
                        # "Mount the string options that will appear in these controls."
                        n37 = Unbundle By Name(w123) -> ("Wave1A"=w122:string[], "Wave1B"=w121:string[], "Wave1C"=w120:string[])
                        n38 = property on="A-Wave Shape" class="Ring (strict)"(error in=w119, "Strings []"=w122) -> (error out=w118:errorcluster)  [unwired: 1 in, 1 out]
                        n39 = property on="B-Wave Shape" class="Ring (strict)"(error in=w118, "Strings []"=w121) -> (error out=w117:errorcluster)  [unwired: 1 in, 1 out]
                        n40 = property on="C-Wave Shape" class="Ring (strict)"(error in=w117, "Strings []"=w120) -> (error out=w116:errorcluster)  [unwired: 1 in, 1 out]
                      }
                      frame "Waves2" {
                        # "Mount the string options that will appear in these controls."
                        # "All for Instr2"
                        n41 = Unbundle By Name(w132) -> ("Wave2A"=w131:string[], "Wave2B"=w130:string[], "Wave2C"=w129:string[])
                        n42 = property on="A-Wave Shape" class="Ring (strict)"(error in=w128, "Strings []"=w131) -> (error out=w127:errorcluster)  [unwired: 1 in, 1 out]
                        n43 = property on="B-Wave Shape" class="Ring (strict)"(error in=w127, "Strings []"=w130) -> (error out=w126:errorcluster)  [unwired: 1 in, 1 out]
                        n44 = property on="C-Wave Shape" class="Ring (strict)"(error in=w126, "Strings []"=w129) -> (error out=w125:errorcluster)  [unwired: 1 in, 1 out]
                      }
                      frame "Waves3" {
                        # "Mount the string options that will appear in these controls."
                        # "All for Instr3"
                        n45 = Unbundle By Name(w142) -> ("Wave3A"=w141:string[], "Wave3B"=w140:string[], "Wave3C"=w139:string[])
                        n46 = property on="A-Wave Shape" class="Ring (strict)"(error in=w138, "Strings []"=w141) -> (error out=w137:errorcluster)  [unwired: 1 in, 1 out]
                        n47 = property on="B-Wave Shape" class="Ring (strict)"(error in=w137, "Strings []"=w140) -> (error out=w136:errorcluster)  [unwired: 1 in, 1 out]
                        n48 = property on="C-Wave Shape" class="Ring (strict)"(error in=w136, "Strings []"=w139) -> (error out=w135:errorcluster)  [unwired: 1 in, 1 out]
                      }
                      frame "EnableNames" {
                        w149 = 0 ("disabled index (col)")
                        # "Instr3"
                        # "Instr2"
                        # "Instr1"
                        # "\"Name\" Enabled/Disabled states are in index 0"
                        n49 = Unbundle By Name(w156) -> ("EnableCtrls"=w150:i8[][])
                        n50 = Index Array(array=w150, index (row) #1=0 ("disabled index (row)"), index (col) #1=w149, index (row) #2=1 ("disabled index (row)"), index (col) #2=w149, index (row) #3=2 ("disabled index (row)"), index (col) #3=w149) -> (element #1=w148:i8, element #2=w144:i8, element #3=w143:i8)
                        n51 = property on="Name" class="Str"(error in=w155, "DisabledEnum"=w148) -> (error out=w154:errorcluster)  [unwired: 1 in, 1 out]
                        n52 = property on="Name" class="Str"(error in=w154, "DisabledEnum"=w144) -> (error out=w153:errorcluster)  [unwired: 1 in, 1 out]
                        n53 = property on="Name" class="Str"(error in=w153, "DisabledEnum"=w143) -> (error out=w152:errorcluster)  [unwired: 1 in, 1 out]
                      }
                      frame "EnableFreq" {
                        w163 = 1 ("disabled index (col)")
                        # "Instr3"
                        # "Instr2"
                        # "Instr1"
                        # "FreqOut Enabled/Disabled states are in index 1"
                        n54 = Unbundle By Name(w170) -> ("EnableCtrls"=w164:i8[][])
                        n55 = Index Array(array=w164, index (row) #1=0 ("disabled index (row)"), index (col) #1=w163, index (row) #2=1 ("disabled index (row)"), index (col) #2=w163, index (row) #3=2 ("disabled index (row)"), index (col) #3=w163) -> (element #1=w162:i8, element #2=w158:i8, element #3=w157:i8)
                        n56 = property on="FreqOut (Hz)" class="DigNum (strict)"(error in=w169, "DisabledEnum"=w162) -> (error out=w168:errorcluster)  [unwired: 1 in, 1 out]
                        n57 = property on="FreqOut (Hz)" class="DigNum (strict)"(error in=w168, "DisabledEnum"=w158) -> (error out=w167:errorcluster)  [unwired: 1 in, 1 out]
                        n58 = property on="FreqOut (Hz)" class="DigNum (strict)"(error in=w167, "DisabledEnum"=w157) -> (error out=w166:errorcluster)  [unwired: 1 in, 1 out]
                      }
                      frame "EnableSync" {
                        w177 = 2 ("disabled index (col)")
                        # "Instr3"
                        # "Instr2"
                        # "Instr1"
                        # "Synchronization Enabled/Disabled states are in index 2"
                        n59 = Unbundle By Name(w184) -> ("EnableCtrls"=w178:i8[][])
                        n60 = Index Array(array=w178, index (row) #1=0 ("disabled index (row)"), index (col) #1=w177, index (row) #2=1 ("disabled index (row)"), index (col) #2=w177, index (row) #3=2 ("disabled index (row)"), index (col) #3=w177) -> (element #1=w176:i8, element #2=w172:i8, element #3=w171:i8)
                        n61 = property on="Synchronization" class="Ring (strict)"(error in=w183, "DisabledEnum"=w176) -> (error out=w182:errorcluster)  [unwired: 1 in, 1 out]
                        n62 = property on="Synchronization" class="Ring (strict)"(error in=w182, "DisabledEnum"=w172) -> (error out=w181:errorcluster)  [unwired: 1 in, 1 out]
                        n63 = property on="Synchronization" class="Ring (strict)"(error in=w181, "DisabledEnum"=w171) -> (error out=w180:errorcluster)  [unwired: 1 in, 1 out]
                      }
                      frame "EnableVoltsA" {
                        w192 = 3 ("disabled index (col)")
                        # "Instr3"
                        # "Instr2"
                        # "Instr1"
                        # "Phase-A Volts Enabled/Disabled states are in index 3"
                        n64 = Unbundle By Name(w198) -> ("EnableCtrls"=w193:i8[][])
                        n65 = Index Array(array=w193, index (row) #1=0 ("disabled index (row)"), index (col) #1=w192, index (row) #2=1 ("disabled index (row)"), index (col) #2=w192, index (row) #3=2 ("disabled index (row)"), index (col) #3=w192) -> (element #1=w191:i8, element #2=w187:i8, element #3=w186:i8)
                        n66 = property on="A-Volts (V)" class="DigNum (strict)"(error in=w197, "DisabledEnum"=w191) -> (error out=w196:errorcluster)  [unwired: 1 in, 1 out]
                        n67 = property on="A-Volts (V)" class="DigNum (strict)"(error in=w196, "DisabledEnum"=w187) -> (error out=w195:errorcluster)  [unwired: 1 in, 1 out]
                        n68 = property on="A-Volts (V)" class="DigNum (strict)"(error in=w195, "DisabledEnum"=w186) -> (error out=w194:errorcluster)  [unwired: 1 in, 1 out]
                      }
                      frame "EnableVoltsB" {
                        w206 = 4 ("disabled index (col)")
                        # "Instr3"
                        # "Instr2"
                        # "Instr1"
                        # "Phase-B Volts Enabled/Disabled states are in index 4"
                        n69 = Unbundle By Name(w212) -> ("EnableCtrls"=w207:i8[][])
                        n70 = Index Array(array=w207, index (row) #1=0 ("disabled index (row)"), index (col) #1=w206, index (row) #2=1 ("disabled index (row)"), index (col) #2=w206, index (row) #3=2 ("disabled index (row)"), index (col) #3=w206) -> (element #1=w205:i8, element #2=w201:i8, element #3=w200:i8)
                        n71 = property on="B-Volts (V)" class="DigNum (strict)"(error in=w211, "DisabledEnum"=w205) -> (error out=w210:errorcluster)  [unwired: 1 in, 1 out]
                        n72 = property on="B-Volts (V)" class="DigNum (strict)"(error in=w210, "DisabledEnum"=w201) -> (error out=w209:errorcluster)  [unwired: 1 in, 1 out]
                        n73 = property on="B-Volts (V)" class="DigNum (strict)"(error in=w209, "DisabledEnum"=w200) -> (error out=w208:errorcluster)  [unwired: 1 in, 1 out]
                      }
                      frame "EnableVoltsC" {
                        w220 = 5 ("disabled index (col)")
                        # "Instr3"
                        # "Instr2"
                        # "Instr1"
                        # "Phase-C Volts Enabled/Disabled states are in index 5"
                        n74 = Unbundle By Name(w226) -> ("EnableCtrls"=w221:i8[][])
                        n75 = Index Array(array=w221, index (row) #1=0 ("disabled index (row)"), index (col) #1=w220, index (row) #2=1 ("disabled index (row)"), index (col) #2=w220, index (row) #3=2 ("disabled index (row)"), index (col) #3=w220) -> (element #1=w219:i8, element #2=w215:i8, element #3=w214:i8)
                        n76 = property on="C-Volts (V)" class="DigNum (strict)"(error in=w225, "DisabledEnum"=w219) -> (error out=w224:errorcluster)  [unwired: 1 in, 1 out]
                        n77 = property on="C-Volts (V)" class="DigNum (strict)"(error in=w224, "DisabledEnum"=w215) -> (error out=w223:errorcluster)  [unwired: 1 in, 1 out]
                        n78 = property on="C-Volts (V)" class="DigNum (strict)"(error in=w223, "DisabledEnum"=w214) -> (error out=w222:errorcluster)  [unwired: 1 in, 1 out]
                      }
                      frame "EnablePhaseB" {
                        w234 = 6 ("disabled index (col)")
                        # "Instr3"
                        # "Instr2"
                        # "Instr1"
                        # "Phase-B angle Enabled/Disabled states are in index 6"
                        n79 = Unbundle By Name(w240) -> ("EnableCtrls"=w235:i8[][])
                        n80 = Index Array(array=w235, index (row) #1=0 ("disabled index (row)"), index (col) #1=w234, index (row) #2=1 ("disabled index (row)"), index (col) #2=w234, index (row) #3=2 ("disabled index (row)"), index (col) #3=w234) -> (element #1=w233:i8, element #2=w229:i8, element #3=w228:i8)
                        n81 = property on="B-Angle (Deg)" class="DigNum (strict)"(error in=w239, "DisabledEnum"=w233) -> (error out=w238:errorcluster)  [unwired: 1 in, 1 out]
                        n82 = property on="B-Angle (Deg)" class="DigNum (strict)"(error in=w238, "DisabledEnum"=w229) -> (error out=w237:errorcluster)  [unwired: 1 in, 1 out]
                        n83 = property on="B-Angle (Deg)" class="DigNum (strict)"(error in=w237, "DisabledEnum"=w228) -> (error out=w236:errorcluster)  [unwired: 1 in, 1 out]
                      }
                      frame "EnablePhaseC" {
                        w248 = 7 ("disabled index (col)")
                        # "Instr3"
                        # "Instr2"
                        # "Instr1"
                        # "Phase-B angle Enabled/Disabled states are in index 7"
                        n84 = Unbundle By Name(w254) -> ("EnableCtrls"=w249:i8[][])
                        n85 = Index Array(array=w249, index (row) #1=0 ("disabled index (row)"), index (col) #1=w248, index (row) #2=1 ("disabled index (row)"), index (col) #2=w248, index (row) #3=2 ("disabled index (row)"), index (col) #3=w248) -> (element #1=w247:i8, element #2=w243:i8, element #3=w242:i8)
                        n86 = property on="C-Angle (Deg)" class="DigNum (strict)"(error in=w253, "DisabledEnum"=w247) -> (error out=w252:errorcluster)  [unwired: 1 in, 1 out]
                        n87 = property on="C-Angle (Deg)" class="DigNum (strict)"(error in=w252, "DisabledEnum"=w243) -> (error out=w251:errorcluster)  [unwired: 1 in, 1 out]
                        n88 = property on="C-Angle (Deg)" class="DigNum (strict)"(error in=w251, "DisabledEnum"=w242) -> (error out=w250:errorcluster)  [unwired: 1 in, 1 out]
                      }
                      frame "EnableChangeA" {
                        w262 = 8 ("disabled index (col)")
                        # "Instr3"
                        # "Instr2"
                        # "Instr1"
                        # "Phase-A \"Change at\" Enabled/Disabled states are in index 8"
                        n89 = Unbundle By Name(w268) -> ("EnableCtrls"=w263:i8[][])
                        n90 = Index Array(array=w263, index (row) #1=0 ("disabled index (row)"), index (col) #1=w262, index (row) #2=1 ("disabled index (row)"), index (col) #2=w262, index (row) #3=2 ("disabled index (row)"), index (col) #3=w262) -> (element #1=w261:i8, element #2=w257:i8, element #3=w256:i8)
                        n91 = property on="A-Change at..." class="DigNum (strict)"(error in=w267, "DisabledEnum"=w261) -> (error out=w266:errorcluster)  [unwired: 1 in, 1 out]
                        n92 = property on="A-Change at..." class="DigNum (strict)"(error in=w266, "DisabledEnum"=w257) -> (error out=w265:errorcluster)  [unwired: 1 in, 1 out]
                        n93 = property on="A-Change at..." class="DigNum (strict)"(error in=w265, "DisabledEnum"=w256) -> (error out=w264:errorcluster)  [unwired: 1 in, 1 out]
                      }
                      frame "EnableChangeB" {
                        w276 = 9 ("disabled index (col)")
                        # "Instr3"
                        # "Instr2"
                        # "Instr1"
                        # "Phase-B \"Change at\" Enabled/Disabled states are in index 9"
                        n94 = Unbundle By Name(w282) -> ("EnableCtrls"=w277:i8[][])
                        n95 = Index Array(array=w277, index (row) #1=0 ("disabled index (row)"), index (col) #1=w276, index (row) #2=1 ("disabled index (row)"), index (col) #2=w276, index (row) #3=2 ("disabled index (row)"), index (col) #3=w276) -> (element #1=w275:i8, element #2=w271:i8, element #3=w270:i8)
                        n96 = property on="B-Change at..." class="DigNum (strict)"(error in=w281, "DisabledEnum"=w275) -> (error out=w280:errorcluster)  [unwired: 1 in, 1 out]
                        n97 = property on="B-Change at..." class="DigNum (strict)"(error in=w280, "DisabledEnum"=w271) -> (error out=w279:errorcluster)  [unwired: 1 in, 1 out]
                        n98 = property on="B-Change at..." class="DigNum (strict)"(error in=w279, "DisabledEnum"=w270) -> (error out=w278:errorcluster)  [unwired: 1 in, 1 out]
                      }
                      frame "EnableChangeC" {
                        w290 = 10 ("disabled index (col)")
                        # "Instr3"
                        # "Instr2"
                        # "Instr1"
                        # "Phase-C \"Change at\" Enabled/Disabled states are in index 10"
                        n99 = Unbundle By Name(w296) -> ("EnableCtrls"=w291:i8[][])
                        n100 = Index Array(array=w291, index (row) #1=0 ("disabled index (row)"), index (col) #1=w290, index (row) #2=1 ("disabled index (row)"), index (col) #2=w290, index (row) #3=2 ("disabled index (row)"), index (col) #3=w290) -> (element #1=w289:i8, element #2=w285:i8, element #3=w284:i8)
                        n101 = property on="C-Change at..." class="DigNum (strict)"(error in=w295, "DisabledEnum"=w289) -> (error out=w294:errorcluster)  [unwired: 1 in, 1 out]
                        n102 = property on="C-Change at..." class="DigNum (strict)"(error in=w294, "DisabledEnum"=w285) -> (error out=w293:errorcluster)  [unwired: 1 in, 1 out]
                        n103 = property on="C-Change at..." class="DigNum (strict)"(error in=w293, "DisabledEnum"=w284) -> (error out=w292:errorcluster)  [unwired: 1 in, 1 out]
                      }
                      frame "EnableWavesA" {
                        w304 = 11 ("disabled index (col)")
                        # "Instr3"
                        # "Instr2"
                        # "Instr1"
                        # "Phase-A waves Enabled/Disabled states are in index 11"
                        n104 = Unbundle By Name(w310) -> ("EnableCtrls"=w305:i8[][])
                        n105 = Index Array(array=w305, index (row) #1=0 ("disabled index (row)"), index (col) #1=w304, index (row) #2=1 ("disabled index (row)"), index (col) #2=w304, index (row) #3=2 ("disabled index (row)"), index (col) #3=w304) -> (element #1=w303:i8, element #2=w299:i8, element #3=w298:i8)
                        n106 = property on="A-Wave Shape" class="Ring (strict)"(error in=w309, "DisabledEnum"=w303) -> (error out=w308:errorcluster)  [unwired: 1 in, 1 out]
                        n107 = property on="A-Wave Shape" class="Ring (strict)"(error in=w308, "DisabledEnum"=w299) -> (error out=w307:errorcluster)  [unwired: 1 in, 1 out]
                        n108 = property on="A-Wave Shape" class="Ring (strict)"(error in=w307, "DisabledEnum"=w298) -> (error out=w306:errorcluster)  [unwired: 1 in, 1 out]
                      }
                      frame "EnableWavesB" {
                        w318 = 12 ("disabled index (col)")
                        # "Instr3"
                        # "Instr2"
                        # "Instr1"
                        # "Phase-B waves Enabled/Disabled states are in index 12"
                        n109 = Unbundle By Name(w324) -> ("EnableCtrls"=w319:i8[][])
                        n110 = Index Array(array=w319, index (row) #1=0 ("disabled index (row)"), index (col) #1=w318, index (row) #2=1 ("disabled index (row)"), index (col) #2=w318, index (row) #3=2 ("disabled index (row)"), index (col) #3=w318) -> (element #1=w317:i8, element #2=w313:i8, element #3=w312:i8)
                        n111 = property on="B-Wave Shape" class="Ring (strict)"(error in=w323, "DisabledEnum"=w317) -> (error out=w322:errorcluster)  [unwired: 1 in, 1 out]
                        n112 = property on="B-Wave Shape" class="Ring (strict)"(error in=w322, "DisabledEnum"=w313) -> (error out=w321:errorcluster)  [unwired: 1 in, 1 out]
                        n113 = property on="B-Wave Shape" class="Ring (strict)"(error in=w321, "DisabledEnum"=w312) -> (error out=w320:errorcluster)  [unwired: 1 in, 1 out]
                      }
                      frame "EnableWavesC" {
                        w332 = 13 ("disabled index (col)")
                        # "Instr3"
                        # "Instr2"
                        # "Instr1"
                        # "Phase-C waves Enabled/Disabled states are in index 13"
                        n114 = Unbundle By Name(w338) -> ("EnableCtrls"=w333:i8[][])
                        n115 = Index Array(array=w333, index (row) #1=0 ("disabled index (row)"), index (col) #1=w332, index (row) #2=1 ("disabled index (row)"), index (col) #2=w332, index (row) #3=2 ("disabled index (row)"), index (col) #3=w332) -> (element #1=w331:i8, element #2=w327:i8, element #3=w326:i8)
                        n116 = property on="C-Wave Shape" class="Ring (strict)"(error in=w337, "DisabledEnum"=w331) -> (error out=w336:errorcluster)  [unwired: 1 in, 1 out]
                        n117 = property on="C-Wave Shape" class="Ring (strict)"(error in=w336, "DisabledEnum"=w327) -> (error out=w335:errorcluster)  [unwired: 1 in, 1 out]
                        n118 = property on="C-Wave Shape" class="Ring (strict)"(error in=w335, "DisabledEnum"=w326) -> (error out=w334:errorcluster)  [unwired: 1 in, 1 out]
                      }
                      frame "EnableCurrSlew" {
                        w346 = 14 ("disabled index (col)")
                        # "Instr3"
                        # "Instr2"
                        # "Instr1"
                        # "Current slew Enabled/Disabled states are in index 14"
                        n119 = Unbundle By Name(w352) -> ("EnableCtrls"=w347:i8[][])
                        n120 = Index Array(array=w347, index (row) #1=0 ("disabled index (row)"), index (col) #1=w346, index (row) #2=1 ("disabled index (row)"), index (col) #2=w346, index (row) #3=2 ("disabled index (row)"), index (col) #3=w346) -> (element #1=w345:i8, element #2=w341:i8, element #3=w340:i8)
                        n121 = property on="Current (A/s)" class="DigNum (strict)"(error in=w351, "DisabledEnum"=w345) -> (error out=w350:errorcluster)  [unwired: 1 in, 1 out]
                        n122 = property on="Current (A/s)" class="DigNum (strict)"(error in=w350, "DisabledEnum"=w341) -> (error out=w349:errorcluster)  [unwired: 1 in, 1 out]
                        n123 = property on="Current (A/s)" class="DigNum (strict)"(error in=w349, "DisabledEnum"=w340) -> (error out=w348:errorcluster)  [unwired: 1 in, 1 out]
                      }
                      frame "EnablePowSlew" {
                        w360 = 15 ("disabled index (col)")
                        # "Instr3"
                        # "Instr2"
                        # "Instr1"
                        # "Power slew Enabled/Disabled states are in index 15"
                        n124 = Unbundle By Name(w366) -> ("EnableCtrls"=w361:i8[][])
                        n125 = Index Array(array=w361, index (row) #1=0 ("disabled index (row)"), index (col) #1=w360, index (row) #2=1 ("disabled index (row)"), index (col) #2=w360, index (row) #3=2 ("disabled index (row)"), index (col) #3=w360) -> (element #1=w359:i8, element #2=w355:i8, element #3=w354:i8)
                        n126 = property on="Power (W/s)" class="DigNum (strict)"(error in=w365, "DisabledEnum"=w359) -> (error out=w364:errorcluster)  [unwired: 1 in, 1 out]
                        n127 = property on="Power (W/s)" class="DigNum (strict)"(error in=w364, "DisabledEnum"=w355) -> (error out=w363:errorcluster)  [unwired: 1 in, 1 out]
                        n128 = property on="Power (W/s)" class="DigNum (strict)"(error in=w363, "DisabledEnum"=w354) -> (error out=w362:errorcluster)  [unwired: 1 in, 1 out]
                      }
                      frame "EnableFreqSlew" {
                        w374 = 16 ("disabled index (col)")
                        # "Instr3"
                        # "Instr2"
                        # "Instr1"
                        # "Frequency slew Enabled/Disabled states are in index 16"
                        n129 = Unbundle By Name(w380) -> ("EnableCtrls"=w375:i8[][])
                        n130 = Index Array(array=w375, index (row) #1=0 ("disabled index (row)"), index (col) #1=w374, index (row) #2=1 ("disabled index (row)"), index (col) #2=w374, index (row) #3=2 ("disabled index (row)"), index (col) #3=w374) -> (element #1=w373:i8, element #2=w369:i8, element #3=w368:i8)
                        n131 = property on="Frequency (Hz/s)" class="DigNum (strict)"(error in=w379, "DisabledEnum"=w373) -> (error out=w378:errorcluster)  [unwired: 1 in, 1 out]
                        n132 = property on="Frequency (Hz/s)" class="DigNum (strict)"(error in=w378, "DisabledEnum"=w369) -> (error out=w377:errorcluster)  [unwired: 1 in, 1 out]
                        n133 = property on="Frequency (Hz/s)" class="DigNum (strict)"(error in=w377, "DisabledEnum"=w368) -> (error out=w376:errorcluster)  [unwired: 1 in, 1 out]
                      }
                      frame "EnablePhaseSlew" {
                        w388 = 17 ("disabled index (col)")
                        # "Instr3"
                        # "Instr2"
                        # "Instr1"
                        # "Frequency slew Enabled/Disabled states are in index 17"
                        n134 = Unbundle By Name(w394) -> ("EnableCtrls"=w389:i8[][])
                        n135 = Index Array(array=w389, index (row) #1=0 ("disabled index (row)"), index (col) #1=w388, index (row) #2=1 ("disabled index (row)"), index (col) #2=w388, index (row) #3=2 ("disabled index (row)"), index (col) #3=w388) -> (element #1=w387:i8, element #2=w383:i8, element #3=w382:i8)
                        n136 = property on="Phase Angle (Deg/s)" class="DigNum (strict)"(error in=w393, "DisabledEnum"=w387) -> (error out=w392:errorcluster)  [unwired: 1 in, 1 out]
                        n137 = property on="Phase Angle (Deg/s)" class="DigNum (strict)"(error in=w392, "DisabledEnum"=w383) -> (error out=w391:errorcluster)  [unwired: 1 in, 1 out]
                        n138 = property on="Phase Angle (Deg/s)" class="DigNum (strict)"(error in=w391, "DisabledEnum"=w382) -> (error out=w390:errorcluster)  [unwired: 1 in, 1 out]
                      }
                    }
                  }
                  frame Error {
                    # "If the config file gives an error, discard the config procedure."
                  }
                }
              }
            }
          }
          n139 = call-dynamic "CountChassis.vi"("NhRegenGridSim in"=w25, "error in (no error)"=w20) -> ("NhRegenGridSim out"=w27:refnum<class "NHRGridSim.lvclass">, "Chassis"=w24:u32, "ChassisTxt"=w23:string, "ChassisStatus"=w22:T15, "error out"=w21:errorcluster)  [unwired: 8 in, 1 out]
          n140 = case shown="\"Enabled\"" w22 {
            selector: w22 -> [w403 w409]
            tunnel: w21 -> [w402 w408]
            tunnel: [w401 w407] -> w26
            frame "Enabled" {
              n141 = property on="Chassis" class="DigNum (strict)"(error in=w402, "DisabledEnum"=w403, "NumText.BGColor"=u32 16777225, "NumText.TextColor"=u32 16777228, "NumText.FontBold"=FALSE ("Numeric Text.Font:Bold")) -> (error out=w401:errorcluster)  [unwired: 1 in, 1 out]
            }
            frame "Disabled", Default {
              n142 = property on="Chassis" class="DigNum (strict)"(error in=w408, "DisabledEnum"=w409, "NumText.BGColor"=u32 16777228, "NumText.TextColor"=u32 6618880, "NumText.FontBold"=TRUE ("Numeric Text.Font:Bold")) -> (error out=w407:errorcluster)  [unwired: 1 in, 1 out]
            }
          }
          n143 = local write "Chassis"(w24) -> ()
          n144 = local write "ChassisTxt"(w23) -> ()
        }
        frame Enabled {
        }
      }
      n145 = while {
        shift-right: [w417] -> w14
        shift-left: w7 -> [w418]
        tunnel: [w419] -> w19
        tunnel: [w415] -> w13
        tunnel: w6 -> [w416]
        tunnel: [w412] -> w9
        stop <- w414 stop-if-true
        n146 = event shown="[1] \"btnSave\": Value Change" {
          selector: _ -> [_ _ _ _ _ _ _ _ _ _ _ _ _ _ _ _ _ _ _ _ _ _ _ _ _ _ _ _ _ _ _ _]
          dyn-events: _ -> [_ _ _ _ _ _ _ _ _ _ _ _ _ _ _ _ _ _ _ _ _ _ _ _ _ _ _ _ _ _ _ _]
          timeout: _ -> [_ _ _ _ _ _ _ _ _ _ _ _ _ _ _ _ _ _ _ _ _ _ _ _ _ _ _ _ _ _ _ _]
          tunnel: [w420 w445 w461 _ w830 w2036 w2065 w2368 w2416 w2456 w2480 w2504 w2525 w2539 w2561 w2639 w2668 w2691 w2825 w2851 w2893 w2943 w2969 w2991 w3006 w3031 w3107 w3136 w3158 w3221 w3251 w3271] -> w419
          tunnel: [TRUE w445 w461 _ w830 w2036 w2065 w2368 w2416 w2456 w2480 w2504 w2525 w2539 w2561 w2639 w2668 w2691 w2825 w2851 w2893 w2943 w2969 w2991 w3006 w3031 w3107 w3136 w3158 w3221 w3251 w3271] -> w413
          tunnel: w418 -> [w422 w426 w460 w497 w833 w2037 w2066 w2369 w2417 w2457 w2481 w2505 w2526 w2538 w2562 w2640 w2669 w2694 w2827 w2853 w2895 w2945 w2971 w2993 w3008 w3032 w3108 w3137 w3159 w3223 w3253 w3273]
          tunnel: [w422 w434 w457 w497 w833 w2037 w2066 w2369 w2417 w2457 w2481 w2505 w2526 w2531 w2562 w2640 w2669 w2694 w2827 w2853 w2895 w2945 w2971 w2993 w3008 w3032 w3108 w3137 w3159 w3223 w3253 w3273] -> w417
          tunnel: [w421 w444 w458 w494 w826 w2033 w2042 w2366 w2414 w2454 w2478 w2502 w2519 w2527 w2557 w2635 w2664 w2682 w2819 w2845 w2890 w2940 w2966 w2986 w3001 w3022 w3098 w3127 w3155 w3218 w3248 w3268] -> w412
          tunnel: w416 -> [w421 w425 w459 w496 w831 w2027 w2052 w2350 w2398 w2446 w2470 w2500 w2520 w2532 w2550 w2627 w2656 w2684 w2820 w2846 w2883 w2933 w2959 w2987 w3002 w3019 w3096 w3125 w3152 w3214 w3244 w3264]
          tunnel: [w420 FALSE w461 _ w830 w2036 w2065 w2368 w2416 w2456 w2480 w2504 w2525 w2539 w2561 w2639 w2668 w2691 w2825 w2851 w2893 w2943 w2969 w2991 w3006 w3031 w3107 w3136 w3158 w3221 w3251 w3271] -> w415
          event "btnCancel": Value Change {
            w420 = FALSE
            # "Cancel the configuration operation with saving any changes"
            n147 = event-data() -> ()  [unwired: 1 in, 1 out]
          }
          event "btnSave": Value Change {
            w445 = TRUE ("StartMeas")
            # "Always write a false to the .ini file since the initialize function may have been called before the PrefDialog.vi"
            # "Save the changes made to the configuration properties"
            n148 = event-data() -> ()  [unwired: 1 in, 1 out]
            n149 = local read "Device(s)Settings"() -> (w424:T1)
            n150 = Bundle By Name(cluster=w424, "Connected"=FALSE) -> (w428:T1)
            n151 = local read "Measurement RefreshTime (ms)"() -> (w437:u32)
            n152 = local read "Measurements"() -> (w435:T9)
            n153 = To Variant(anything=w428) -> (Variant=w440:variant)
            n154 = To Variant(anything=w435) -> (Variant=w439:variant)
            n155 = call-dynamic "WriteToBaseConfigVariant.vi"("Measurement RefreshTime (ms)"=w437, "error in (no error)"=w425, "Meas"=w439, "Config"=w440, "NHRGridSim in"=w426) -> ("error out"=w438:errorcluster, "NHRGridSim out"=w427:refnum<class "NHRGridSim.lvclass">)  [unwired: 5 in]
            n156 = property class="NHRGridSim.lvclass"(reference=w427, error in=w438) -> (reference out=w434:refnum<class "NHRGridSim.lvclass">, error out=w433:errorcluster, "Accessors:PluginIniFilePath"=w436:path, "Accessors:BaseConfig"=w432:T16, "Accessors:BaseMeasurements"=w431:T18)
            n157 = local read "Measurement RefreshTime (ms)"() -> (w430:u32)
            n158 = call <vilib>:"Open Config Data.vi"("error in (no error)"=w433, "create file if necessary (T)"=FALSE, "configuration file path"=w436) -> ("error out"=w441:errorcluster, "refnum"=w442:T20)  [unwired: 6 in, 1 out]
            n159 = call-dynamic "WriteFile.vi"("Measurement Refresh Time (ms)"=w430, "Refnum in"=w442, "error in (no error)"=w441, "BaseMeasurements"=w431, "BaseConfiguration"=w432, "NHRGridSim in"=w427) -> ("error out"=w444:errorcluster)  [unwired: 4 in, 1 out]
          }
          event "btnSaveAs": Value Change {
            # "Save the configuration properties to a different file in the same location as the original file."
            n160 = event-data() -> ()  [unwired: 1 in, 1 out]
            n161 = property class="NHRGridSim.lvclass"(reference=w460, error in=w459) -> (reference out=w456:refnum<class "NHRGridSim.lvclass">, error out=w450:errorcluster, "Accessors:PluginIniFilePath"=w451:path)
            n162 = local read "Device(s)Settings"() -> (w453:T1)
            n163 = local read "Measurements"() -> (w455:T9)
            n164 = local read "Measurement RefreshTime (ms)"() -> (w454:u32)
            n165 = call "SaveAsFileDialog.vi"("error in"=w450, "Current File"=w451) -> ("error out"=w449:errorcluster, "Cancelled?"=w447:bool, "selected file path"=w448:path, "Current File out"=w452:path)  [unwired: 6 in]
            n166 = case shown="False" w447 {
              tunnel: [TRUE FALSE] -> w461
              tunnel: [w489 w491] -> w458
              tunnel: [w488 w493] -> w457
              tunnel: w456 -> [w475 w493]
              tunnel: w455 -> [w473 _]
              tunnel: w454 -> [w471 _]
              tunnel: w453 -> [w464 _]
              tunnel: w449 -> [w469 w491]
              tunnel: w452 -> [w468 _]
              tunnel: w448 -> [w467 _]
              frame False {
                # "Always write a false to the .ini file since the initialize function may have been called before the PrefDialog.vi"
                n167 = Bundle By Name(cluster=w464, "Connected"=FALSE) -> (w465:T1)
                n168 = Copy(8:w469, 10:w467, 11:w468) -> (0:w478:errorcluster, 3:w485:path)  [unwired: 2 in, 1 out]
                n169 = To Variant(anything=w473) -> (Variant=w472:variant)
                n170 = To Variant(anything=w464) -> (Variant=w474:variant)
                n171 = call-dynamic "WriteToBaseConfigVariant.vi"("Measurement RefreshTime (ms)"=w471, "error in (no error)"=w478, "Meas"=w472, "Config"=w474, "NHRGridSim in"=w475) -> ("error out"=w477:errorcluster, "NHRGridSim out"=w476:refnum<class "NHRGridSim.lvclass">)  [unwired: 5 in]
                n172 = property class="NHRGridSim.lvclass"(reference=w476, error in=w477, "Accessors:PluginIniFilePath"=w485) -> (reference out=w488:refnum<class "NHRGridSim.lvclass">, error out=w482:errorcluster, "Accessors:PluginIniFilePath"=w484:path, "Accessors:BaseConfig"=w483:T16, "Accessors:BaseMeasurements"=w480:T18)
                n173 = To Variant(anything=w473) -> (Variant=w479:variant)
                n174 = To Variant(anything=w465) -> (Variant=w487:variant)
                n175 = call-dynamic "WriteToBaseConfigVariant.vi"("Measurement RefreshTime (ms)"=w471, "error in (no error)"=w482, "Meas"=w479, "Config"=w487, "NHRGridSim in"=w488) -> ("error out"=w481:errorcluster, "NHRGridSim out"=w486:refnum<class "NHRGridSim.lvclass">)  [unwired: 5 in]
                n176 = call <vilib>:"Open Config Data.vi"("error in (no error)"=w481, "create file if necessary (T)"=FALSE, "configuration file path"=w484) -> ("error out"=w462:errorcluster, "refnum"=w463:T20)  [unwired: 6 in, 1 out]
                n177 = call-dynamic "WriteFile.vi"("Measurement Refresh Time (ms)"=w471, "Refnum in"=w463, "error in (no error)"=w462, "BaseMeasurements"=w480, "BaseConfiguration"=w483, "NHRGridSim in"=w486) -> ("error out"=w489:errorcluster)  [unwired: 4 in, 1 out]
              }
              frame True {
              }
            }
          }
          event "Update": Value Change {
            # "The reason to save the user available selections of the Voltage Range, Current Range, Configure Instrument, and AC Wave Shape controls is because the options that these controls will show to the user vary depending on Mode. If they were not stored in separate arrays from the index value of the present selection in the control, there would be no way to either save the options to or read them from a INI file. The Mode control doesn't need this treatment because the list of Mode options never changes. Saving the Mode value is enough."
            # "Populate the Device(s)Settings cluster every time that a change in the settings of the PrefDialog controls is made"
            n178 = event-data() -> ()  [unwired: 1 in, 1 out]
            n179 = while {
              shift-right: [w501] -> _
              shift-left: NHRGrid_UpdateSettings."VRanges" -> [w502]
              shift-right: [w498] -> w494
              shift-left: w496 -> [w499]
              stop <- w500 stop-if-true
              # "The frames are to avoid race conditions writing to the Device(s)Settings cluster."
              n180 = case shown="\"Values\"" w502 {
                tunnel: [NHRGrid_UpdateSettings."CRanges" NHRGrid_UpdateSettings."Syncs" NHRGrid_UpdateSettings."Waves" NHRGrid_UpdateSettings."Values" NHRGrid_UpdateSettings."SaveEnables1" NHRGrid_UpdateSettings."SaveEnables2" NHRGrid_UpdateSettings."SaveEnables3" NHRGrid_UpdateSettings."SaveEnables4" NHRGrid_UpdateSettings."SaveEnables5" NHRGrid_UpdateSettings."SaveEnables6" _] -> w501
                tunnel: [FALSE FALSE FALSE FALSE FALSE FALSE FALSE FALSE FALSE FALSE TRUE] -> w500
                tunnel: w499 -> [w507 w527 w547 w567 w600 w647 w665 w693 w733 w764 w798]
                tunnel: [w504 w526 w544 w564 w599 w629 w655 w696 w730 w761 w789] -> w498
                frame "VRanges", Default {
                  # "The list of options for the Voltage Range changes depending on Mode. Save  the present list of V Range options in the instruments."
                  n181 = flat-sequence {
                    tunnel: w507 -> [w516]
                    tunnel: [w519] -> w506
                    tunnel: [w513] -> w505
                    tunnel: w506 -> [w522]
                    tunnel: [w521] -> w504
                    tunnel: w505 -> [w521]
                    frame #0 {
                      # "These are the actual ones to save."
                      # "These are only for feedback."
                      # "Instr1"
                      # "Instr2"
                      # "Instr3"
                      # "Instr3"
                      # "Instr2"
                      # "Instr1"
                      n182 = property on="Voltage (V)" class="Ring (strict)"(error in=w516) -> (error out=w518:errorcluster, "Strings []"=w509:string[])  [unwired: 1 in, 1 out]
                      n183 = property on="Voltage (V)" class="Ring (strict)"(error in=w518) -> (error out=w517:errorcluster, "Strings []"=w510:string[])  [unwired: 1 in, 1 out]
                      n184 = property on="Voltage (V)" class="Ring (strict)"(error in=w517) -> (error out=w512:errorcluster, "Strings []"=w511:string[])  [unwired: 1 in, 1 out]
                      n185 = property on="Voltage (V)" class="Ring (strict)"(error in=w512, "Strings []"=w511) -> (error out=w514:errorcluster)  [unwired: 1 in, 1 out]
                      n186 = property on="Voltage (V)" class="Ring (strict)"(error in=w514, "Strings []"=w510) -> (error out=w515:errorcluster)  [unwired: 1 in, 1 out]
                      n187 = property on="Voltage (V)" class="Ring (strict)"(error in=w515, "Strings []"=w509) -> (error out=w513:errorcluster)  [unwired: 1 in, 1 out]
                      n188 = local read "Device(s)Settings"() -> (w520:T1)
                      n189 = Bundle By Name(cluster=w520, "VRangeVals3"=w511, "VRangeVals2"=w510, "VRangeVals1"=w509) -> (w519:T1)
                    }
                    frame #1 {
                      n190 = local write "Device(s)Settings"(w522) -> ()
                    }
                  }
                }
                frame "CRanges" {
                  # "The list of options for the Current Range changes depending on Mode. Save  the present list of options in the instruments."
                  n191 = flat-sequence {
                    tunnel: w527 -> [w538]
                    tunnel: [w532] -> w525
                    tunnel: [w539] -> w524
                    tunnel: [w542] -> w526
                    tunnel: w525 -> [w542]
                    tunnel: w524 -> [w541]
                    frame #0 {
                      # "These are the actual ones to save."
                      # "These are only for feedback."
                      # "Instr1"
                      # "Instr2"
                      # "Instr3"
                      # "Instr3"
                      # "Instr2"
                      # "Instr1"
                      n192 = property on="Current (A)" class="Ring (strict)"(error in=w538) -> (error out=w537:errorcluster, "Strings []"=w529:string[])  [unwired: 1 in, 1 out]
                      n193 = property on="Current (A)" class="Ring (strict)"(error in=w537) -> (error out=w536:errorcluster, "Strings []"=w530:string[])  [unwired: 1 in, 1 out]
                      n194 = property on="Current (A)" class="Ring (strict)"(error in=w536) -> (error out=w533:errorcluster, "Strings []"=w531:string[])  [unwired: 1 in, 1 out]
                      n195 = property on="Current (A)" class="Ring (strict)"(error in=w533, "Strings []"=w531) -> (error out=w534:errorcluster)  [unwired: 1 in, 1 out]
                      n196 = property on="Current (A)" class="Ring (strict)"(error in=w534, "Strings []"=w530) -> (error out=w535:errorcluster)  [unwired: 1 in, 1 out]
                      n197 = property on="Current (A)" class="Ring (strict)"(error in=w535, "Strings []"=w529) -> (error out=w532:errorcluster)  [unwired: 1 in, 1 out]
                      n198 = local read "Device(s)Settings"() -> (w540:T1)
                      n199 = Bundle By Name(cluster=w540, "CRangeVals3"=w531, "CRangeVals2"=w530, "CRangeVals1"=w529) -> (w539:T1)
                    }
                    frame #1 {
                      n200 = local write "Device(s)Settings"(w541) -> ()
                    }
                  }
                }
                frame "Syncs" {
                  # "The list of options for the Synchronization control changes depending on Mode. Save the present list of options in the instruments."
                  n201 = flat-sequence {
                    tunnel: w547 -> [w558]
                    tunnel: [w559] -> w546
                    tunnel: [w553] -> w545
                    tunnel: w546 -> [w562]
                    tunnel: w545 -> [w561]
                    tunnel: [w561] -> w544
                    frame #0 {
                      # "Update the values in Device(s)Settings controls too"
                      # "Instr1"
                      # "Instr2"
                      # "Instr3"
                      # "Instr3"
                      # "Instr2"
                      # "Instr1"
                      n202 = property on="Synchronization" class="Ring (strict)"(error in=w558) -> (error out=w557:errorcluster, "Strings []"=w549:string[])  [unwired: 1 in, 1 out]
                      n203 = property on="Synchronization" class="Ring (strict)"(error in=w557) -> (error out=w556:errorcluster, "Strings []"=w550:string[])  [unwired: 1 in, 1 out]
                      n204 = property on="Synchronization" class="Ring (strict)"(error in=w556) -> (error out=w552:errorcluster, "Strings []"=w551:string[])  [unwired: 1 in, 1 out]
                      n205 = property on="Synchronization" class="Ring (strict)"(error in=w552, "Strings []"=w551) -> (error out=w554:errorcluster)  [unwired: 1 in, 1 out]
                      n206 = property on="Synchronization" class="Ring (strict)"(error in=w554, "Strings []"=w550) -> (error out=w555:errorcluster)  [unwired: 1 in, 1 out]
                      n207 = local read "Device(s)Settings"() -> (w560:T1)
                      n208 = property on="Synchronization" class="Ring (strict)"(error in=w555, "Strings []"=w549) -> (error out=w553:errorcluster)  [unwired: 1 in, 1 out]
                      n209 = Bundle By Name(cluster=w560, "SyncList3"=w551, "SyncList2"=w550, "SyncList1"=w549) -> (w559:T1)
                    }
                    frame #1 {
                      n210 = local write "Device(s)Settings"(w562) -> ()
                    }
                  }
                }
                frame "Waves" {
                  # "The list of options for the AC phase waveforms changes depending on Mode. Save  the present list of options in the instruments."
                  n211 = flat-sequence {
                    tunnel: w567 -> [w573]
                    tunnel: [w569] -> w566
                    tunnel: w566 -> [w584]
                    tunnel: [w579] -> w565
                    tunnel: w565 -> [w594]
                    tunnel: [w590] -> w564
                    frame #0 {
                      # "Instr1"
                      n212 = property on="A-Wave Shape" class="Ring (strict)"(error in=w573) -> (error out=w572:errorcluster, "Strings []"=w578:string[])  [unwired: 1 in, 1 out]
                      n213 = property on="B-Wave Shape" class="Ring (strict)"(error in=w573) -> (error out=w571:errorcluster, "Strings []"=w577:string[])  [unwired: 1 in, 1 out]
                      n214 = property on="C-Wave Shape" class="Ring (strict)"(error in=w573) -> (error out=w570:errorcluster, "Strings []"=w576:string[])  [unwired: 1 in, 1 out]
                      n215 = local read "Device(s)Settings"() -> (w575:T1)
                      n216 = Bundle By Name(cluster=w575, "Wave1A"=w578, "Wave1B"=w577, "Wave1C"=w576) -> (w574:T1)
                      n217 = local write "Device(s)Settings"(w574) -> ()
                      n218 = Merge Errors(w572, w571, w570) -> (w569:errorcluster)
                    }
                    frame #1 {
                      # "Instr2"
                      n219 = property on="A-Wave Shape" class="Ring (strict)"(error in=w584) -> (error out=w580:errorcluster, "Strings []"=w588:string[])  [unwired: 1 in, 1 out]
                      n220 = property on="B-Wave Shape" class="Ring (strict)"(error in=w584) -> (error out=w581:errorcluster, "Strings []"=w587:string[])  [unwired: 1 in, 1 out]
                      n221 = property on="C-Wave Shape" class="Ring (strict)"(error in=w584) -> (error out=w582:errorcluster, "Strings []"=w586:string[])  [unwired: 1 in, 1 out]
                      n222 = local read "Device(s)Settings"() -> (w585:T1)
                      n223 = Bundle By Name(cluster=w585, "Wave2A"=w588, "Wave2B"=w587, "Wave2C"=w586) -> (w583:T1)
                      n224 = local write "Device(s)Settings"(w583) -> ()
                      n225 = Merge Errors(w580, w581, w582) -> (w579:errorcluster)
                    }
                    frame #2 {
                      # "Instr3"
                      n226 = property on="A-Wave Shape" class="Ring (strict)"(error in=w594) -> (error out=w591:errorcluster, "Strings []"=w598:string[])  [unwired: 1 in, 1 out]
                      n227 = property on="B-Wave Shape" class="Ring (strict)"(error in=w594) -> (error out=w592:errorcluster, "Strings []"=w597:string[])  [unwired: 1 in, 1 out]
                      n228 = property on="C-Wave Shape" class="Ring (strict)"(error in=w594) -> (error out=w593:errorcluster, "Strings []"=w596:string[])  [unwired: 1 in, 1 out]
                      n229 = local read "Device(s)Settings"() -> (w595:T1)
                      n230 = Bundle By Name(cluster=w595, "Wave3A"=w598, "Wave3B"=w597, "Wave3C"=w596) -> (w589:T1)
                      n231 = local write "Device(s)Settings"(w589) -> ()
                      n232 = Merge Errors(w591, w592, w593) -> (w590:errorcluster)
                    }
                  }
                }
                frame "Values" {
                  # "Exchange the data that can be passed directly between the Instruments and the Device(s)Settings cluster."
                  n233 = flat-sequence {
                    tunnel: [w609] -> w603
                    tunnel: [w605] -> w601
                    tunnel: w600 -> [w605]
                    tunnel: w603 -> [w618]
                    tunnel: w601 -> [w617]
                    tunnel: [w617] -> w599
                    frame #0 {
                      # "This will take care of passing everything that is simply a value or an indexed setting choice. Some controls will share values directly. The clusters will only pass values, the properties of some of their controls need to be specified in a different way or Device(s)Settings will have no way to register them."
                      n234 = local read "Instr1"() -> (w608:T2)
                      n235 = local read "Instr3"() -> (w606:T2)
                      n236 = local read "ID Query"() -> (w615:bool)
                      n237 = local read "Reset"() -> (w613:bool)
                      n238 = local read "Instr2"() -> (w607:T2)
                      n239 = local read "MeasName"() -> (w611:string)
                      n240 = local read "Connected"() -> (w614:bool)
                      n241 = local read "Mode"() -> (w616:T8)
                      n242 = local read "Handle"() -> (w612:string)
                      n243 = local read "Device(s)Settings"() -> (w610:T1)
                      n244 = Bundle By Name(cluster=w610, "MeasName"=w611, "Instr1"=w608, "Instr2"=w607, "Instr3"=w606, "Handle"=w612, "Reset"=w613, "Connected"=w614, "ID Query"=w615, "Mode"=w616) -> (w609:T1)
                    }
                    frame #1 {
                      n245 = local write "Device(s)Settings"(w618) -> ()
                    }
                  }
                }
                frame "SaveEnables1" {
                  # "Instr3"
                  # "Instr2"
                  # "Instr1"
                  # "Instr3"
                  # "Instr2"
                  # "Instr1"
                  # "Instr3"
                  # "Instr2"
                  # "Instr1"
                  n246 = property on="Name" class="Str"(error in=w647) -> (error out=w650:errorcluster, "DisabledEnum"=w620:T15)  [unwired: 1 in, 1 out]
                  n247 = local read "Device(s)Settings"() -> (w648:T1)
                  n248 = property on="Name" class="Str"(error in=w650) -> (error out=w651:errorcluster, "DisabledEnum"=w621:T15)  [unwired: 1 in, 1 out]
                  n249 = Unbundle By Name(w648) -> ("EnableCtrls"=w623:i8[][])
                  n250 = property on="Name" class="Str"(error in=w651) -> (error out=w642:errorcluster, "DisabledEnum"=w622:T15)  [unwired: 1 in, 1 out]
                  n251 = Build Array(w620, w621, w622) -> (w619:T21)
                  n252 = property on="FreqOut (Hz)" class="DigNum (strict)"(error in=w642) -> (error out=w646:errorcluster, "DisabledEnum"=w639:T15)  [unwired: 1 in, 1 out]
                  n253 = Replace Array Subset(array=w623, new element=w619, index (col)=0 ("disabled index (col)")) -> (w624:i8[][])  [unwired: 1 in]
                  n254 = property on="FreqOut (Hz)" class="DigNum (strict)"(error in=w646) -> (error out=w645:errorcluster, "DisabledEnum"=w640:T15)  [unwired: 1 in, 1 out]
                  n255 = property on="FreqOut (Hz)" class="DigNum (strict)"(error in=w645) -> (error out=w636:errorcluster, "DisabledEnum"=w641:T15)  [unwired: 1 in, 1 out]
                  n256 = Build Array(w639, w640, w641) -> (w643:T21)
                  n257 = property on="Synchronization" class="Ring (strict)"(error in=w636) -> (error out=w638:errorcluster, "DisabledEnum"=w632:T15)  [unwired: 1 in, 1 out]
                  n258 = Replace Array Subset(array=w624, new element=w643, index (col)=1 ("disabled index (col)")) -> (w633:i8[][])  [unwired: 1 in]
                  n259 = property on="Synchronization" class="Ring (strict)"(error in=w638) -> (error out=w637:errorcluster, "DisabledEnum"=w631:T15)  [unwired: 1 in, 1 out]
                  n260 = property on="Synchronization" class="Ring (strict)"(error in=w637) -> (error out=w629:errorcluster, "DisabledEnum"=w630:T15)  [unwired: 1 in, 1 out]
                  n261 = Build Array(w632, w631, w630) -> (w634:T21)
                  n262 = local read "Device(s)Settings"() -> (w649:T1)
                  n263 = Replace Array Subset(array=w633, new element=w634, index (col)=2 ("disabled index (col)")) -> (w628:i8[][])  [unwired: 1 in]
                  n264 = Bundle By Name(cluster=w649, "EnableCtrls"=w628) -> (w627:T1)
                  n265 = local write "Device(s)Settings"(w627) -> ()
                }
                frame "SaveEnables2" {
                  # "Instr3"
                  # "Instr2"
                  # "Instr1"
                  # "Instr3"
                  # "Instr2"
                  # "Instr1"
                  # "Instr3"
                  # "Instr2"
                  # "Instr1"
                  n266 = property on="A-Volts (V)" class="DigNum (strict)"(error in=w665) -> (error out=w667:errorcluster, "DisabledEnum"=w660:T15)  [unwired: 1 in, 1 out]
                  n267 = local read "Device(s)Settings"() -> (w683:T1)
                  n268 = property on="A-Volts (V)" class="DigNum (strict)"(error in=w667) -> (error out=w666:errorcluster, "DisabledEnum"=w661:T15)  [unwired: 1 in, 1 out]
                  n269 = property on="A-Volts (V)" class="DigNum (strict)"(error in=w666) -> (error out=w664:errorcluster, "DisabledEnum"=w662:T15)  [unwired: 1 in, 1 out]
                  n270 = Unbundle By Name(w683) -> ("EnableCtrls"=w682:i8[][])
                  n271 = Build Array(w660, w661, w662) -> (w681:T21)
                  n272 = property on="B-Volts (V)" class="DigNum (strict)"(error in=w664) -> (error out=w669:errorcluster, "DisabledEnum"=w657:T15)  [unwired: 1 in, 1 out]
                  n273 = Replace Array Subset(array=w682, new element=w681, index (col)=3 ("disabled index (col)")) -> (w678:i8[][])  [unwired: 1 in]
                  n274 = property on="B-Volts (V)" class="DigNum (strict)"(error in=w669) -> (error out=w668:errorcluster, "DisabledEnum"=w658:T15)  [unwired: 1 in, 1 out]
                  n275 = property on="B-Volts (V)" class="DigNum (strict)"(error in=w668) -> (error out=w663:errorcluster, "DisabledEnum"=w659:T15)  [unwired: 1 in, 1 out]
                  n276 = Build Array(w657, w658, w659) -> (w679:T21)
                  n277 = Replace Array Subset(array=w678, new element=w679, index (col)=4 ("disabled index (col)")) -> (w675:i8[][])  [unwired: 1 in]
                  n278 = property on="C-Volts (V)" class="DigNum (strict)"(error in=w663) -> (error out=w671:errorcluster, "DisabledEnum"=w653:T15)  [unwired: 1 in, 1 out]
                  n279 = property on="C-Volts (V)" class="DigNum (strict)"(error in=w671) -> (error out=w670:errorcluster, "DisabledEnum"=w654:T15)  [unwired: 1 in, 1 out]
                  n280 = property on="C-Volts (V)" class="DigNum (strict)"(error in=w670) -> (error out=w655:errorcluster, "DisabledEnum"=w656:T15)  [unwired: 1 in, 1 out]
                  n281 = Build Array(w653, w654, w656) -> (w676:T21)
                  n282 = local read "Device(s)Settings"() -> (w685:T1)
                  n283 = Replace Array Subset(array=w675, new element=w676, index (col)=5 ("disabled index (col)")) -> (w674:i8[][])  [unwired: 1 in]
                  n284 = Bundle By Name(cluster=w685, "EnableCtrls"=w674) -> (w673:T1)
                  n285 = local write "Device(s)Settings"(w673) -> ()
                }
                frame "SaveEnables3" {
                  # "Instr3"
                  # "Instr2"
                  # "Instr1"
                  # "Instr3"
                  # "Instr2"
                  # "Instr1"
                  # "Instr3"
                  # "Instr2"
                  # "Instr1"
                  n286 = property on="B-Angle (Deg)" class="DigNum (strict)"(error in=w693) -> (error out=w701:errorcluster, "DisabledEnum"=w687:T15)  [unwired: 1 in, 1 out]
                  n287 = local read "Device(s)Settings"() -> (w717:T1)
                  n288 = property on="B-Angle (Deg)" class="DigNum (strict)"(error in=w701) -> (error out=w700:errorcluster, "DisabledEnum"=w688:T15)  [unwired: 1 in, 1 out]
                  n289 = Unbundle By Name(w717) -> ("EnableCtrls"=w716:i8[][])
                  n290 = property on="B-Angle (Deg)" class="DigNum (strict)"(error in=w700) -> (error out=w694:errorcluster, "DisabledEnum"=w689:T15)  [unwired: 1 in, 1 out]
                  n291 = Build Array(w687, w688, w689) -> (w715:T21)
                  n292 = property on="C-Angle (Deg)" class="DigNum (strict)"(error in=w694) -> (error out=w703:errorcluster, "DisabledEnum"=w690:T15)  [unwired: 1 in, 1 out]
                  n293 = Replace Array Subset(array=w716, new element=w715, index (col)=6 ("disabled index (col)")) -> (w712:i8[][])  [unwired: 1 in]
                  n294 = property on="C-Angle (Deg)" class="DigNum (strict)"(error in=w703) -> (error out=w702:errorcluster, "DisabledEnum"=w691:T15)  [unwired: 1 in, 1 out]
                  n295 = property on="C-Angle (Deg)" class="DigNum (strict)"(error in=w702) -> (error out=w695:errorcluster, "DisabledEnum"=w692:T15)  [unwired: 1 in, 1 out]
                  n296 = Build Array(w690, w691, w692) -> (w713:T21)
                  n297 = property on="A-Change at..." class="DigNum (strict)"(error in=w695) -> (error out=w705:errorcluster, "DisabledEnum"=w697:T15)  [unwired: 1 in, 1 out]
                  n298 = Replace Array Subset(array=w712, new element=w713, index (col)=7 ("disabled index (col)")) -> (w709:i8[][])  [unwired: 1 in]
                  n299 = property on="A-Change at..." class="DigNum (strict)"(error in=w705) -> (error out=w704:errorcluster, "DisabledEnum"=w698:T15)  [unwired: 1 in, 1 out]
                  n300 = property on="A-Change at..." class="DigNum (strict)"(error in=w704) -> (error out=w696:errorcluster, "DisabledEnum"=w699:T15)  [unwired: 1 in, 1 out]
                  n301 = Build Array(w697, w698, w699) -> (w710:T21)
                  n302 = local read "Device(s)Settings"() -> (w719:T1)
                  n303 = Replace Array Subset(array=w709, new element=w710, index (col)=8 ("disabled index (col)")) -> (w708:i8[][])  [unwired: 1 in]
                  n304 = Bundle By Name(cluster=w719, "EnableCtrls"=w708) -> (w707:T1)
                  n305 = local write "Device(s)Settings"(w707) -> ()
                }
                frame "SaveEnables4" {
                  # "Instr3"
                  # "Instr2"
                  # "Instr1"
                  # "Instr3"
                  # "Instr2"
                  # "Instr1"
                  # "Instr3"
                  # "Instr2"
                  # "Instr1"
                  n306 = property on="B-Change at..." class="DigNum (strict)"(error in=w733) -> (error out=w735:errorcluster, "DisabledEnum"=w721:T15)  [unwired: 1 in, 1 out]
                  n307 = local read "Device(s)Settings"() -> (w751:T1)
                  n308 = property on="B-Change at..." class="DigNum (strict)"(error in=w735) -> (error out=w734:errorcluster, "DisabledEnum"=w722:T15)  [unwired: 1 in, 1 out]
                  n309 = property on="B-Change at..." class="DigNum (strict)"(error in=w734) -> (error out=w732:errorcluster, "DisabledEnum"=w723:T15)  [unwired: 1 in, 1 out]
                  n310 = Unbundle By Name(w751) -> ("EnableCtrls"=w750:i8[][])
                  n311 = Build Array(w721, w722, w723) -> (w749:T21)
                  n312 = property on="C-Change at..." class="DigNum (strict)"(error in=w732) -> (error out=w737:errorcluster, "DisabledEnum"=w724:T15)  [unwired: 1 in, 1 out]
                  n313 = Replace Array Subset(array=w750, new element=w749, index (col)=9 ("disabled index (col)")) -> (w746:i8[][])  [unwired: 1 in]
                  n314 = property on="C-Change at..." class="DigNum (strict)"(error in=w737) -> (error out=w736:errorcluster, "DisabledEnum"=w725:T15)  [unwired: 1 in, 1 out]
                  n315 = property on="C-Change at..." class="DigNum (strict)"(error in=w736) -> (error out=w731:errorcluster, "DisabledEnum"=w726:T15)  [unwired: 1 in, 1 out]
                  n316 = Build Array(w724, w725, w726) -> (w747:T21)
                  n317 = property on="A-Wave Shape" class="Ring (strict)"(error in=w731) -> (error out=w739:errorcluster, "DisabledEnum"=w727:T15)  [unwired: 1 in, 1 out]
                  n318 = Replace Array Subset(array=w746, new element=w747, index (col)=10 ("disabled index (col)")) -> (w743:i8[][])  [unwired: 1 in]
                  n319 = property on="A-Wave Shape" class="Ring (strict)"(error in=w739) -> (error out=w738:errorcluster, "DisabledEnum"=w728:T15)  [unwired: 1 in, 1 out]
                  n320 = property on="A-Wave Shape" class="Ring (strict)"(error in=w738) -> (error out=w730:errorcluster, "DisabledEnum"=w729:T15)  [unwired: 1 in, 1 out]
                  n321 = Build Array(w727, w728, w729) -> (w744:T21)
                  n322 = local read "Device(s)Settings"() -> (w753:T1)
                  n323 = Replace Array Subset(array=w743, new element=w744, index (col)=11 ("disabled index (col)")) -> (w742:i8[][])  [unwired: 1 in]
                  n324 = Bundle By Name(cluster=w753, "EnableCtrls"=w742) -> (w741:T1)
                  n325 = local write "Device(s)Settings"(w741) -> ()
                }
                frame "SaveEnables5" {
                  # "Instr1"
                  # "Instr3"
                  # "Instr2"
                  # "Instr1"
                  # "Instr3"
                  # "Instr2"
                  # "Instr1"
                  # "Instr3"
                  # "Instr2"
                  # "Instr1"
                  n326 = property on="B-Wave Shape" class="Ring (strict)"(error in=w764) -> (error out=w769:errorcluster, "DisabledEnum"=w765:T15)  [unwired: 1 in, 1 out]
                  n327 = local read "Device(s)Settings"() -> (w785:T1)
                  n328 = property on="B-Wave Shape" class="Ring (strict)"(error in=w769) -> (error out=w768:errorcluster, "DisabledEnum"=w766:T15)  [unwired: 1 in, 1 out]
                  n329 = property on="B-Wave Shape" class="Ring (strict)"(error in=w768) -> (error out=w763:errorcluster, "DisabledEnum"=w767:T15)  [unwired: 1 in, 1 out]
                  n330 = Unbundle By Name(w785) -> ("EnableCtrls"=w784:i8[][])
                  n331 = Build Array(w765, w766, w767) -> (w783:T21)
                  n332 = property on="C-Wave Shape" class="Ring (strict)"(error in=w763) -> (error out=w771:errorcluster, "DisabledEnum"=w758:T15)  [unwired: 1 in, 1 out]
                  n333 = Replace Array Subset(array=w784, new element=w783, index (col)=12 ("disabled index (col)")) -> (w780:i8[][])  [unwired: 1 in]
                  n334 = property on="C-Wave Shape" class="Ring (strict)"(error in=w771) -> (error out=w770:errorcluster, "DisabledEnum"=w759:T15)  [unwired: 1 in, 1 out]
                  n335 = property on="C-Wave Shape" class="Ring (strict)"(error in=w770) -> (error out=w762:errorcluster, "DisabledEnum"=w760:T15)  [unwired: 1 in, 1 out]
                  n336 = Build Array(w758, w759, w760) -> (w781:T21)
                  n337 = property on="Current (A/s)" class="DigNum (strict)"(error in=w762) -> (error out=w773:errorcluster, "DisabledEnum"=w755:T15)  [unwired: 1 in, 1 out]
                  n338 = Replace Array Subset(array=w780, new element=w781, index (col)=13 ("disabled index (col)")) -> (w777:i8[][])  [unwired: 1 in]
                  n339 = property on="Current (A/s)" class="DigNum (strict)"(error in=w773) -> (error out=w772:errorcluster, "DisabledEnum"=w756:T15)  [unwired: 1 in, 1 out]
                  n340 = property on="Current (A/s)" class="DigNum (strict)"(error in=w772) -> (error out=w761:errorcluster, "DisabledEnum"=w757:T15)  [unwired: 1 in, 1 out]
                  n341 = Build Array(w755, w756, w757) -> (w778:T21)
                  n342 = local read "Device(s)Settings"() -> (w787:T1)
                  n343 = Replace Array Subset(array=w777, new element=w778, index (col)=14 ("disabled index (col)")) -> (w776:i8[][])  [unwired: 1 in]
                  n344 = Bundle By Name(cluster=w787, "EnableCtrls"=w776) -> (w775:T1)
                  n345 = local write "Device(s)Settings"(w775) -> ()
                }
                frame "SaveEnables6" {
                  # "Instr1"
                  # "Instr3"
                  # "Instr2"
                  # "Instr1"
                  # "Instr3"
                  # "Instr2"
                  # "Instr1"
                  # "Instr3"
                  # "Instr2"
                  # "Instr1"
                  n346 = property on="Power (W/s)" class="DigNum (strict)"(error in=w798) -> (error out=w803:errorcluster, "DisabledEnum"=w799:T15)  [unwired: 1 in, 1 out]
                  n347 = local read "Device(s)Settings"() -> (w818:T1)
                  n348 = property on="Power (W/s)" class="DigNum (strict)"(error in=w803) -> (error out=w802:errorcluster, "DisabledEnum"=w800:T15)  [unwired: 1 in, 1 out]
                  n349 = property on="Power (W/s)" class="DigNum (strict)"(error in=w802) -> (error out=w797:errorcluster, "DisabledEnum"=w801:T15)  [unwired: 1 in, 1 out]
                  n350 = Unbundle By Name(w818) -> ("EnableCtrls"=w817:i8[][])
                  n351 = Build Array(w799, w800, w801) -> (w816:T21)
                  n352 = property on="Frequency (Hz/s)" class="DigNum (strict)"(error in=w797) -> (error out=w805:errorcluster, "DisabledEnum"=w796:T15)  [unwired: 1 in, 1 out]
                  n353 = Replace Array Subset(array=w817, new element=w816, index (col)=15 ("disabled index (col)")) -> (w813:i8[][])  [unwired: 1 in]
                  n354 = property on="Frequency (Hz/s)" class="DigNum (strict)"(error in=w805) -> (error out=w804:errorcluster, "DisabledEnum"=w795:T15)  [unwired: 1 in, 1 out]
                  n355 = property on="Frequency (Hz/s)" class="DigNum (strict)"(error in=w804) -> (error out=w793:errorcluster, "DisabledEnum"=w794:T15)  [unwired: 1 in, 1 out]
                  n356 = Build Array(w796, w795, w794) -> (w814:T21)
                  n357 = property on="Phase Angle (Deg/s)" class="DigNum (strict)"(error in=w793) -> (error out=w807:errorcluster, "DisabledEnum"=w792:T15)  [unwired: 1 in, 1 out]
                  n358 = Replace Array Subset(array=w813, new element=w814, index (col)=16 ("disabled index (col)")) -> (w810:i8[][])  [unwired: 1 in]
                  n359 = property on="Phase Angle (Deg/s)" class="DigNum (strict)"(error in=w807) -> (error out=w806:errorcluster, "DisabledEnum"=w791:T15)  [unwired: 1 in, 1 out]
                  n360 = property on="Phase Angle (Deg/s)" class="DigNum (strict)"(error in=w806) -> (error out=w789:errorcluster, "DisabledEnum"=w790:T15)  [unwired: 1 in, 1 out]
                  n361 = Build Array(w792, w791, w790) -> (w811:T21)
                  n362 = local read "Device(s)Settings"() -> (w820:T1)
                  n363 = Replace Array Subset(array=w810, new element=w811, index (col)=17 ("disabled index (col)")) -> (w809:i8[][])  [unwired: 1 in]
                  n364 = Bundle By Name(cluster=w820, "EnableCtrls"=w809) -> (w808:T1)
                  n365 = local write "Device(s)Settings"(w808) -> ()
                }
              }
            }
          }
          event Value Change {
            w827 = T15."Enabled" ("Disabled")
            w830 = FALSE ("StartMeas")
            # "Update Device(s)Settings"
            n366 = event-data() -> ()  [unwired: 1 in, 1 out]
            n367 = while {
              shift-right: [w836] -> _
              shift-left: NHRGrid_ModeAdjust_Tabs."ShowTabs" ("AcPwrPlugins.lvlib:NHRGridSim.lvclass:NHRGrid_ModeAdjust_Tabs") -> [w838]
              shift-right: [w837] -> w824
              shift-left: w831 -> [w834]
              stop <- w835 stop-if-true
              n368 = case shown="No Error" w834 {
                selector: w834 -> [w839 w2025]
                tunnel: w838 -> [w843 w2023]
                tunnel: [w842 w2025] -> w837
                tunnel: [w841 w2023] -> w836
                tunnel: [w840 TRUE] -> w835
                frame No Error {
                  n369 = case shown="\"CurrRanges\"" w843 {
                    tunnel: w839 -> [w854 w902 w934 w963 w996 w1000 w1042 w1085 w1130 w1174 w1194 w1246 w1280 w1487 w1522 w1557 w1598 w1650 w1703 w1742 w1771 w1801 w1829 w1870 w1889 w1900 w1917 w1957 w1963]
                    tunnel: [w845 w899 w935 w962 w993 w999 w1041 w1084 w1131 w1165 w1195 w1245 w1271 w1506 w1521 w1556 w1599 w1651 w1704 w1746 w1775 w1804 w1833 w1873 w1892 w1911 w1916 w1938 w1972] -> w842
                    tunnel: [NHRGrid_ModeAdjust_Tabs."InstrNames" ("AcPwrPlugins.lvlib:NHRGridSim.lvclass:NHRGrid_ModeAdjust_Tabs") NHRGrid_ModeAdjust_Tabs."VoltRanges" ("AcPwrPlugins.lvlib:NHRGridSim.lvclass:NHRGrid_ModeAdjust_Tabs") NHRGrid_ModeAdjust_Tabs."ConfigSync" ("AcPwrPlugins.lvlib:NHRGridSim.lvclass:NHRGrid_ModeAdjust_Tabs") NHRGrid_ModeAdjust_Tabs."Safety" ("AcPwrPlugins.lvlib:NHRGridSim.lvclass:NHRGrid_ModeAdjust_Tabs") NHRGrid_ModeAdjust_Tabs."Phases" ("AcPwrPlugins.lvlib:NHRGridSim.lvclass:NHRGrid_ModeAdjust_Tabs") NHRGrid_ModeAdjust_Tabs."FreqOut" ("AcPwrPlugins.lvlib:NHRGridSim.lvclass:NHRGrid_ModeAdjust_Tabs") NHRGrid_ModeAdjust_Tabs."PhaseEnable" ("AcPwrPlugins.lvlib:NHRGridSim.lvclass:NHRGrid_ModeAdjust_Tabs") NHRGrid_ModeAdjust_Tabs."SyncEnable" ("AcPwrPlugins.lvlib:NHRGridSim.lvclass:NHRGrid_ModeAdjust_Tabs") NHRGrid_ModeAdjust_Tabs."ChangeEnable" ("AcPwrPlugins.lvlib:NHRGridSim.lvclass:NHRGrid_ModeAdjust_Tabs") NHRGrid_ModeAdjust_Tabs."VoltsEnable" ("AcPwrPlugins.lvlib:NHRGridSim.lvclass:NHRGrid_ModeAdjust_Tabs") NHRGrid_ModeAdjust_Tabs."Vtype" ("AcPwrPlugins.lvlib:NHRGridSim.lvclass:NHRGrid_ModeAdjust_Tabs") NHRGrid_ModeAdjust_Tabs."Description" ("AcPwrPlugins.lvlib:NHRGridSim.lvclass:NHRGrid_ModeAdjust_Tabs") NHRGrid_ModeAdjust_Tabs."CurrRanges" ("AcPwrPlugins.lvlib:NHRGridSim.lvclass:NHRGrid_ModeAdjust_Tabs") NHRGrid_ModeAdjust_Tabs."VoutCoerce" ("AcPwrPlugins.lvlib:NHRGridSim.lvclass:NHRGrid_ModeAdjust_Tabs") NHRGrid_ModeAdjust_Tabs."VSlewCoerce" ("AcPwrPlugins.lvlib:NHRGridSim.lvclass:NHRGrid_ModeAdjust_Tabs") NHRGrid_ModeAdjust_Tabs."CSlewCoerce" ("AcPwrPlugins.lvlib:NHRGridSim.lvclass:NHRGrid_ModeAdjust_Tabs") NHRGrid_ModeAdjust_Tabs."PSlewCoerce" ("AcPwrPlugins.lvlib:NHRGridSim.lvclass:NHRGrid_ModeAdjust_Tabs") NHRGrid_ModeAdjust_Tabs."F&PhCoerce" ("AcPwrPlugins.lvlib:NHRGridSim.lvclass:NHRGrid_ModeAdjust_Tabs") NHRGrid_ModeAdjust_Tabs."SlewsCurr" ("AcPwrPlugins.lvlib:NHRGridSim.lvclass:NHRGrid_ModeAdjust_Tabs") NHRGrid_ModeAdjust_Tabs."SlewsPow" ("AcPwrPlugins.lvlib:NHRGridSim.lvclass:NHRGrid_ModeAdjust_Tabs") NHRGrid_ModeAdjust_Tabs."SlewsFreq" ("AcPwrPlugins.lvlib:NHRGridSim.lvclass:NHRGrid_ModeAdjust_Tabs") NHRGrid_ModeAdjust_Tabs."SlewsPhase" ("AcPwrPlugins.lvlib:NHRGridSim.lvclass:NHRGrid_ModeAdjust_Tabs") NHRGrid_ModeAdjust_Tabs."TripTCoerce1" ("AcPwrPlugins.lvlib:NHRGridSim.lvclass:NHRGrid_ModeAdjust_Tabs") NHRGrid_ModeAdjust_Tabs."TripTCoerce2" ("AcPwrPlugins.lvlib:NHRGridSim.lvclass:NHRGrid_ModeAdjust_Tabs") NHRGrid_ModeAdjust_Tabs."TripTCoerce3" ("AcPwrPlugins.lvlib:NHRGridSim.lvclass:NHRGrid_ModeAdjust_Tabs") NHRGrid_ModeAdjust_Tabs."VPhaseCoerce" ("AcPwrPlugins.lvlib:NHRGridSim.lvclass:NHRGrid_ModeAdjust_Tabs") NHRGrid_ModeAdjust_Tabs."WaveLists" ("AcPwrPlugins.lvlib:NHRGridSim.lvclass:NHRGrid_ModeAdjust_Tabs") NHRGrid_ModeAdjust_Tabs."WaveEnable" ("AcPwrPlugins.lvlib:NHRGridSim.lvclass:NHRGrid_ModeAdjust_Tabs") NHRGrid_ModeAdjust_Tabs."ShowTabs" ("AcPwrPlugins.lvlib:NHRGridSim.lvclass:NHRGrid_ModeAdjust_Tabs")] -> w841
                    tunnel: [FALSE FALSE FALSE FALSE FALSE FALSE FALSE FALSE FALSE FALSE FALSE FALSE FALSE FALSE FALSE FALSE FALSE FALSE FALSE FALSE FALSE FALSE FALSE FALSE FALSE FALSE FALSE FALSE TRUE] -> w840
                    frame "ShowTabs", Default {
                      # "Display chosen Mode"
                      # "Get the reference of each instrument tab."
                      # "Store the visibility properties of the tabs so that they can be loaded from a config file the same way."
                      # "Mode determines number of instruments (and their respective tabs) visible on each configuration."
                      n370 = local read "Mode"() -> (w844:T8)
                      n371 = property on="Instruments" class="TabCtl (strict)"(error in=w854) -> (error out=w853:errorcluster, "Pages"=w855:refnum<vi>[])  [unwired: 1 in, 1 out]
                      n372 = local write "ModeVal"(w844) -> ()
                      n373 = for {
                        tunnel: w855 -> [w861] mode=indexing
                        tunnel: w844 -> [w862]
                        shift-right: [w858] -> w850
                        shift-left: w853 -> [w859]
                        tunnel: [w857] -> w849 mode=indexing
                        tunnel: [w856] -> w847
                        i -> [w860]
                        n374 = case shown="0..2, Default" w862 {
                          tunnel: w861 -> [w875 w889 w896]
                          tunnel: w860 -> [w870 w884 _]
                          tunnel: w859 -> [w868 w882 w894]
                          tunnel: [w867 w881 w893] -> w858
                          tunnel: [w866 w880 w892] -> w857
                          tunnel: [w863 w879 w890] -> w856
                          frame 0..2, Default {
                            w864 = FALSE ("x .or. y?")
                            # "Only Tab1 should be enabled"
                            n375 = Equal?(x=0, y=w870) -> (x = y?=w871:bool)
                            n376 = Select(t=TRUE ("x .or. y?"), s=w871, f=FALSE ("x .or. y?")) -> (s? t:f=w874:bool)
                            n377 = property class="Page"(reference=w875, error in=w868, "PageVis"=w874) -> (reference out=w866:refnum<vi>, error out=w867:errorcluster)
                            n378 = Build Array(TRUE ("x .or. y?"), w864, w864) -> (w863:bool[])
                          }
                          frame 5..8, 11, 12 {
                            # "Only tabs 1 and 3 should be enabled"
                            n379 = Equal?(x=1, y=w884) -> (x = y?=w885:bool)
                            n380 = Select(t=FALSE ("x .or. y?"), s=w885, f=TRUE ("x .or. y?")) -> (s? t:f=w888:bool)
                            n381 = property class="Page"(reference=w889, error in=w882, "PageVis"=w888) -> (reference out=w880:refnum<vi>, error out=w881:errorcluster)
                            n382 = Build Array(TRUE ("x .or. y?"), FALSE ("x .or. y?"), TRUE ("x .or. y?")) -> (w879:bool[])
                          }
                          frame 3, 4, 9, 10, 13..15 {
                            w891 = TRUE ("x .or. y?")
                            # "All three tabs should be enabled"
                            n383 = property class="Page"(reference=w896, error in=w894, "PageVis"=TRUE ("x .or. y?")) -> (reference out=w892:refnum<vi>, error out=w893:errorcluster)
                            n384 = Build Array(w891, w891, w891) -> (w890:bool[])
                          }
                        }
                      }
                      n385 = local read "Device(s)Settings"() -> (w848:T1)
                      n386 = Close Reference(reference=w849, error in (no error)=w850) -> (error out=w845:errorcluster)
                      n387 = Bundle By Name(cluster=w848, "TabPages"=w847) -> (w846:T1)
                      n388 = local write "Device(s)Settings"(w846) -> ()
                    }
                    frame "InstrNames" {
                      w897 = T15."Disabled" ("Disabled")
                      # "Store the same status given to the Name controls in Device(s)Settings for later retrieval."
                      # "Instr3"
                      # "Instr2"
                      # "Instr1"
                      # "Don't allow the user to alter the default name assigned to each instrument"
                      # "Logcial Instrument Name assigned for each Mode"
                      n389 = flat-sequence {
                        tunnel: [w911] -> w903
                        tunnel: w902 -> [w911]
                        frame #0 {
                          w915 = string[][] [["AC1", "AC1", "AC1"], ["AC1", "AC1", "AC1"], ["DC1", "DC1", "DC1"], ["AC1", "AC2", "AC3"], ["DC1", "DC2", "DC3"], ["AC1", "AC1", "AC3"], ["AC1", "AC1", "DC3"], ["AC1", "AC1", "AC3"], ["AC1", "AC1", "DC3"], ["AC1", "AC2", "DC3"], ["AC1", "DC2", "DC3"], ["DC1", "DC1", "AC3"], ["DC1", "DC1", "DC3"], ["AC1", "DC2", "AC3"], ["DC1", "AC2", "AC3"], ["DC1", "AC2", "DC3"]]  # Names
                          # "Row = Mode\nCol = Instrument Name"
                          n390 = local read "Mode"() -> (w922:T8)
                          n391 = Index Array(array=w915, index (row) #1=w922, index (col) #1=0 ("disabled index (col)"), index (row) #2=w922, index (col) #2=1 ("disabled index (col)"), index (row) #3=w922, index (col) #3=2 ("disabled index (col)")) -> (element #1=w924:string, element #2=w923:string, element #3=w925:string)
                          n392 = local read "Instr1"() -> (w916:T2)
                          n393 = Bundle By Name(cluster=w916, "Name"=w924) -> (w917:T2)
                          n394 = local read "Instr2"() -> (w918:T2)
                          n395 = Bundle By Name(cluster=w918, "Name"=w923) -> (w919:T2)
                          n396 = local read "Instr3"() -> (w920:T2)
                          n397 = Bundle By Name(cluster=w920, "Name"=w925) -> (w921:T2)
                          n398 = local write "Instr1"(w917) -> ()
                          n399 = local write "Instr2"(w919) -> ()
                          n400 = local write "Instr3"(w921) -> ()
                        }
                      }
                      n401 = property on="Name" class="Str"(error in=w903, "DisabledEnum"=w897) -> (error out=w908:errorcluster)  [unwired: 1 in, 1 out]
                      n402 = property on="Name" class="Str"(error in=w908, "DisabledEnum"=w897) -> (error out=w907:errorcluster)  [unwired: 1 in, 1 out]
                      n403 = property on="Name" class="Str"(error in=w907, "DisabledEnum"=w897) -> (error out=w898:errorcluster)  [unwired: 1 in, 1 out]
                      n404 = property on="EnableCtrls" class="Arr (strict)"(error in=w898) -> (error out=w900:errorcluster, "Value"=w901:i8[][])  [unwired: 1 in, 1 out]
                      n405 = Build Array(w897, w897, w897) -> (w905:T21)
                      n406 = Replace Array Subset(array=w901, new element=w905, index (col)=0 ("disabled index (col)")) -> (w904:i8[][])  [unwired: 1 in]
                      n407 = property on="EnableCtrls" class="Arr (strict)"(error in=w900, "Value"=w904) -> (error out=w899:errorcluster)  [unwired: 1 in, 1 out]
                    }
                    frame "VoltRanges" {
                      w928 = string[][] [["303", "606"], ["175", "350"], ["200", "400"], ["175", "350"], ["200", "400"], ["175", "350"], ["200", "400"], ["175", "350"], ["200", "400"], ["200", "400"], ["200", "400"], ["175", "350"], ["200", "400"], ["175", "350"], ["175", "350"], ["200", "400"]]  # VRanges3
                      w930 = string[][] [["303", "606"], ["175", "350"], ["200", "400"], ["175", "350"], ["200", "400"], ["350", "500"], ["350", "500"], ["175", "350"], ["175", "350"], ["175", "350"], ["200", "400"], ["200", "400"], ["200", "400"], ["200", "400"], ["175", "350"], ["175", "350"]]  # VRanges2
                      w932 = string[][] [["303", "606"], ["175", "350"], ["200", "400"], ["175", "350"], ["200", "400"], ["350", "500"], ["350", "500"], ["175", "350"], ["175", "350"], ["175", "350"], ["175", "350"], ["200", "400"], ["200", "400"], ["175", "350"], ["200", "400"], ["200", "400"]]  # VRanges1
                      # "Mode determines the strings shown as Voltage Range options in the different instrument controls."
                      # "Instr3"
                      # "Instr2"
                      # "Instr1"
                      # "Multiphase, single phase, and DC instruments have different voltage ranges"
                      n408 = flat-sequence {
                        tunnel: [w940] -> w933
                        tunnel: w934 -> [w940]
                        frame #0 {
                          # "Reinitialize all Vout values and set the voltage range in all instruments to the maximum."
                          n409 = local read "Instr1"() -> (w951:T2)
                          n410 = Bundle By Name(cluster=w951, "Vout (V)"=0.0 ("Value"), "Ranges.Voltage (V)"=u16 1) -> (w952:T2)
                          n411 = local read "Instr3"() -> (w943:T2)
                          n412 = Bundle By Name(cluster=w943, "Vout (V)"=0.0 ("Value"), "Ranges.Voltage (V)"=u16 1) -> (w944:T2)
                          n413 = local read "Instr2"() -> (w946:T2)
                          n414 = Bundle By Name(cluster=w946, "Vout (V)"=0.0 ("Value"), "Ranges.Voltage (V)"=u16 1) -> (w945:T2)
                          n415 = local write "Instr1"(w952) -> ()
                          n416 = local write "Instr3"(w944) -> ()
                          n417 = local write "Instr2"(w945) -> ()
                        }
                      }
                      n418 = local read "Mode"() -> (w927:T8)
                      n419 = Index Array(array=w932, index (row)=w927) -> (element=w931:string[])  [unwired: 1 in]
                      n420 = Index Array(array=w930, index (row)=w927) -> (element=w929:string[])  [unwired: 1 in]
                      n421 = Index Array(array=w928, index (row)=w927) -> (element=w926:string[])  [unwired: 1 in]
                      n422 = property on="Voltage (V)" class="Ring (strict)"(error in=w933, "Strings []"=w931) -> (error out=w936:errorcluster)  [unwired: 1 in, 1 out]
                      n423 = property on="Voltage (V)" class="Ring (strict)"(error in=w936, "Strings []"=w929) -> (error out=w937:errorcluster)  [unwired: 1 in, 1 out]
                      n424 = property on="Voltage (V)" class="Ring (strict)"(error in=w937, "Strings []"=w926) -> (error out=w935:errorcluster)  [unwired: 1 in, 1 out]
                    }
                    frame "ConfigSync" {
                      # "Set the values also in the Device(s)Settings instruments"
                      # "Set the Sync selections to be \"Immediate\" by default"
                      # "Instr3"
                      # "Instr2"
                      # "Instr1"
                      # "Multiphase instruments  will have a \"Sync to Phase A\" configuration available; Single phase ones will be just \"Sync\". For DC, this setting is irrelevant."
                      n425 = local read "Mode"() -> (w966:T8)
                      n426 = case shown="Default" w966 {
                        tunnel: [w980 w985 w990] -> w959
                        tunnel: [w980 w985 w990] -> w958
                        tunnel: [w980 w984 w990] -> w957
                        tunnel: w963 -> [w979 w983 w989]
                        tunnel: [w979 w983 w989] -> w956
                        frame 0 {
                          # "Three-phase Mode"
                          n427 = Build Array("Immediate" ("element"), "Sync to Phase A" ("element")) -> (w980:string[])
                        }
                        frame 5, 6 {
                          w986 = "Immediate" ("element")
                          # "Two-phase Mode for Instr1/2"
                          n428 = Build Array(w986, "Sync to Phase A" ("element")) -> (w985:string[])
                          n429 = Build Array(w986, "Sync" ("element")) -> (w984:string[])
                        }
                        frame Default {
                          # "Instruments with no phases"
                          n430 = Build Array("Immediate" ("element"), "Sync" ("element")) -> (w990:string[])
                        }
                      }
                      n431 = property on="Synchronization" class="Ring (strict)"(error in=w956, "Strings []"=w959) -> (error out=w964:errorcluster)  [unwired: 1 in, 1 out]
                      n432 = property on="Synchronization" class="Ring (strict)"(error in=w956, "Strings []"=w959) -> (error out=w961:errorcluster)  [unwired: 1 in, 1 out]
                      n433 = property on="Synchronization" class="Ring (strict)"(error in=w964, "Strings []"=w958) -> (error out=w965:errorcluster)  [unwired: 1 in, 1 out]
                      n434 = property on="Synchronization" class="Ring (strict)"(error in=w961, "Strings []"=w958) -> (error out=w960:errorcluster)  [unwired: 1 in, 1 out]
                      n435 = property on="Synchronization" class="Ring (strict)"(error in=w965, "Strings []"=w957) -> (error out=w954:errorcluster)  [unwired: 1 in, 1 out]
                      n436 = property on="Synchronization" class="Ring (strict)"(error in=w960, "Strings []"=w957) -> (error out=w953:errorcluster)  [unwired: 1 in, 1 out]
                      n437 = Merge Errors(w953, w954) -> (w955:errorcluster)
                      n438 = flat-sequence {
                        tunnel: w955 -> [w971]
                        tunnel: [w971] -> w962
                        frame #0 {
                          w969 = T3 0 items=["Immediate", "Sync to Phase A"] ("Synchronization")
                          w970 = T3 0 items=["Immediate", "Sync to Phase A"] ("Synchronization")
                          w976 = T3 0 items=["Immediate", "Sync to Phase A"] ("Synchronization")
                          n439 = local read "Instr1"() -> (w978:T2)
                          n440 = Bundle By Name(cluster=w978, "Synchronization"=w976) -> (w977:T2)
                          n441 = local read "Instr2"() -> (w974:T2)
                          n442 = Bundle By Name(cluster=w974, "Synchronization"=w970) -> (w975:T2)
                          n443 = local read "Instr3"() -> (w973:T2)
                          n444 = Bundle By Name(cluster=w973, "Synchronization"=w969) -> (w972:T2)
                          n445 = local write "Instr1"(w977) -> ()
                          n446 = local write "Instr2"(w975) -> ()
                          n447 = local write "Instr3"(w972) -> ()
                        }
                      }
                    }
                    frame "Safety" {
                      # "The defaults are:\n\n1) All times set to \"-1\" = trips monitoring deactivated\n2) All trip level values for current, voltage, and power set to 0\n3) Abs Current Peak and Abs Voltage Peak both disabled."
                      # "Instr3"
                      # "Instr2"
                      # "Instr1"
                      # "Recall the default cluster values for the \"Safety Trips\" in all instruments"
                      n448 = invoke on="Safety Trips" class="Clust (strict)" method="Reinit To Default"(error in=w996) -> (error out=w995:errorcluster)  [unwired: 2 in, 2 out]
                      n449 = invoke on="Safety Trips" class="Clust (strict)" method="Reinit To Default"(error in=w995) -> (error out=w994:errorcluster)  [unwired: 2 in, 2 out]
                      n450 = invoke on="Safety Trips" class="Clust (strict)" method="Reinit To Default"(error in=w994) -> (error out=w993:errorcluster)  [unwired: 2 in, 2 out]
                    }
                    frame "Phases" {
                      # "Set the default phase angles for the multiphase Mode cases. Also, initialize all phase voltage values to 0 volts, and Apertures to 1 cycle."
                      n451 = local read "Mode"() -> (w1001:T8)
                      n452 = case shown="0" w1001 {
                        tunnel: w1000 -> [w1011 w1021 w1033]
                        tunnel: [w1011 w1021 w1033] -> w999
                        frame 0 {
                          w1004 = 0.0 ("Phases.B-Volts (V)")
                          w1005 = 0.0 ("Phases.B-Volts (V)")
                          w1006 = 0.0 ("Phases.B-Volts (V)")
                          w1010 = 120 ("Phases.C-Angle (Deg)")
                          w1012 = 240 ("Phases.B-Angle (Deg)")
                          # "Three Phase Mode: all Instrs have B=240, C=120 degrees"
                          n453 = local read "Instr1"() -> (w1013:T2)
                          n454 = Bundle By Name(cluster=w1013, "Phases.B-Angle (Deg)"=w1012, "Aperture (cycles)"=1, "Phases.A-Volts (V)"=w1006, "Phases.B-Volts (V)"=w1006, "Phases.C-Volts (V)"=w1006, "Phases.C-Angle (Deg)"=w1010) -> (w1014:T2)
                          n455 = local write "Instr1"(w1014) -> ()
                          n456 = local read "Instr2"() -> (w1016:T2)
                          n457 = Bundle By Name(cluster=w1016, "Phases.B-Angle (Deg)"=w1012, "Aperture (cycles)"=1, "Phases.A-Volts (V)"=w1005, "Phases.B-Volts (V)"=w1005, "Phases.C-Volts (V)"=w1005, "Phases.C-Angle (Deg)"=w1010) -> (w1015:T2)
                          n458 = local write "Instr2"(w1015) -> ()
                          n459 = local read "Instr3"() -> (w1017:T2)
                          n460 = Bundle By Name(cluster=w1017, "Phases.B-Angle (Deg)"=w1012, "Aperture (cycles)"=1, "Phases.A-Volts (V)"=w1004, "Phases.B-Volts (V)"=w1004, "Phases.C-Volts (V)"=w1004, "Phases.C-Angle (Deg)"=w1010) -> (w1018:T2)
                          n461 = local write "Instr3"(w1018) -> ()
                        }
                        frame Default {
                          w1019 = 1 ("Aperture (cycles)")
                          w1020 = 0 ("Phases.B-Angle (Deg)")
                          # "Modes with no phases: all Instrs to B=0, C=0"
                          n462 = local read "Instr1"() -> (w1022:T2)
                          n463 = Bundle By Name(cluster=w1022, "Phases.B-Angle (Deg)"=w1020, "Phases.C-Angle (Deg)"=w1020, "Phases.A-Volts (V)"=w1020, "Phases.B-Volts (V)"=w1020, "Phases.C-Volts (V)"=w1020, "Aperture (cycles)"=w1019) -> (w1023:T2)
                          n464 = local write "Instr1"(w1023) -> ()
                          n465 = local read "Instr2"() -> (w1025:T2)
                          n466 = Bundle By Name(cluster=w1025, "Phases.B-Angle (Deg)"=w1020, "Phases.C-Angle (Deg)"=w1020, "Phases.A-Volts (V)"=w1020, "Phases.B-Volts (V)"=w1020, "Phases.C-Volts (V)"=w1020, "Aperture (cycles)"=w1019) -> (w1024:T2)
                          n467 = local write "Instr2"(w1024) -> ()
                          n468 = local read "Instr3"() -> (w1026:T2)
                          n469 = Bundle By Name(cluster=w1026, "Phases.B-Angle (Deg)"=w1020, "Phases.C-Angle (Deg)"=w1020, "Phases.A-Volts (V)"=w1020, "Phases.B-Volts (V)"=w1020, "Phases.C-Volts (V)"=w1020, "Aperture (cycles)"=w1019) -> (w1027:T2)
                          n470 = local write "Instr3"(w1027) -> ()
                        }
                        frame 5, 6 {
                          w1032 = 0 ("Phases.C-Angle (Deg)")
                          w1030 = 180 ("Phases.B-Angle (Deg)")
                          # "Two Phase Modes, B=180 applies only for Instr1/2, all others are B=0, C=0"
                          n471 = local read "Instr1"() -> (w1034:T2)
                          n472 = Bundle By Name(cluster=w1034, "Phases.B-Angle (Deg)"=w1030, "Aperture (cycles)"=1, "Phases.C-Angle (Deg)"=w1032, "Phases.A-Volts (V)"=w1032, "Phases.B-Volts (V)"=w1032, "Phases.C-Volts (V)"=w1032) -> (w1035:T2)
                          n473 = local write "Instr1"(w1035) -> ()
                          n474 = local read "Instr2"() -> (w1037:T2)
                          n475 = Bundle By Name(cluster=w1037, "Phases.B-Angle (Deg)"=w1030, "Aperture (cycles)"=1 ("Phases.B-Angle (Deg)"), "Phases.C-Angle (Deg)"=w1032, "Phases.A-Volts (V)"=w1032, "Phases.B-Volts (V)"=w1032, "Phases.C-Volts (V)"=w1032) -> (w1036:T2)
                          n476 = local write "Instr2"(w1036) -> ()
                          n477 = local read "Instr3"() -> (w1038:T2)
                          n478 = Bundle By Name(cluster=w1038, "Aperture (cycles)"=1, "Phases.B-Angle (Deg)"=w1032, "Phases.C-Angle (Deg)"=w1032, "Phases.A-Volts (V)"=w1032, "Phases.B-Volts (V)"=w1032, "Phases.C-Volts (V)"=w1032) -> (w1039:T2)
                          n479 = local write "Instr3"(w1039) -> ()
                        }
                      }
                    }
                    frame "FreqOut" {
                      # "Depending on Mode, check if each instrument will be AC or DC. The AC ones will have Freq=60 Hz and their FreqOut control will be enabled. The DC ones will have Freq=0 and their FreqOut control will be made unavailable to the user."
                      # "Store the same status given to the FreqOut controls in Device(s)Settings for later retrieval. Frequencies are column index 1 in the array."
                      # "AC instruments will have 60 Hz by default. Disable the DC ones."
                      n480 = for {
                        N: 3 -> [_]
                        shift-right: [w1053] -> w1040
                        shift-left: u8[] [] -> [w1054]
                        shift-right: [w1052] -> w1049
                        shift-left: w1042 -> [w1057]
                        i -> [w1058]
                        w1059 = bool[][] [[TRUE, TRUE, TRUE], [TRUE, TRUE, TRUE], [FALSE, FALSE, FALSE], [TRUE, TRUE, TRUE], [FALSE, FALSE, FALSE], [TRUE, TRUE, TRUE], [TRUE, TRUE, FALSE], [TRUE, TRUE, TRUE], [TRUE, TRUE, FALSE], [TRUE, TRUE, FALSE], [TRUE, FALSE, FALSE], [FALSE, FALSE, TRUE], [FALSE, FALSE, FALSE], [TRUE, FALSE, TRUE], [FALSE, TRUE, TRUE], [FALSE, TRUE, FALSE]]  # Is AC?
                        n481 = local read "Mode"() -> (w1060:T8)
                        n482 = Index Array(array=w1059, index (row)=w1060, index (col)=w1058) -> (element=w1061:bool)
                        n483 = case shown="True" w1061 {
                          tunnel: [0.0 ("x") 60.0 ("x")] -> w1056
                          tunnel: [u8 2 u8 0] -> w1055
                          frame False {
                          }
                          frame True {
                          }
                        }
                        n484 = case shown="2" w1058 {
                          tunnel: w1056 -> [w1065 w1071 w1077]
                          tunnel: w1055 -> [w1064 w1070 w1076]
                          tunnel: w1057 -> [w1063 w1069 w1075]
                          tunnel: [w1062 w1068 w1074] -> w1052
                          frame 0, Default {
                            # "Instr1"
                            n485 = local read "Instr1"() -> (w1066:T2)
                            n486 = Bundle By Name(cluster=w1066, "FreqOut (Hz)"=w1065) -> (w1067:T2)
                            n487 = property on="FreqOut (Hz)" class="DigNum (strict)"(error in=w1063, "DisabledEnum"=w1064) -> (error out=w1062:errorcluster)  [unwired: 1 in, 1 out]
                            n488 = local write "Instr1"(w1067) -> ()
                          }
                          frame 1 {
                            # "Instr2"
                            n489 = local read "Instr2"() -> (w1072:T2)
                            n490 = Bundle By Name(cluster=w1072, "FreqOut (Hz)"=w1071) -> (w1073:T2)
                            n491 = property on="FreqOut (Hz)" class="DigNum (strict)"(error in=w1069, "DisabledEnum"=w1070) -> (error out=w1068:errorcluster)  [unwired: 1 in, 1 out]
                            n492 = local write "Instr2"(w1073) -> ()
                          }
                          frame 2 {
                            # "Instr3"
                            n493 = local read "Instr3"() -> (w1078:T2)
                            n494 = Bundle By Name(cluster=w1078, "FreqOut (Hz)"=w1077) -> (w1079:T2)
                            n495 = property on="FreqOut (Hz)" class="DigNum (strict)"(error in=w1075, "DisabledEnum"=w1076) -> (error out=w1074:errorcluster)  [unwired: 1 in, 1 out]
                            n496 = local write "Instr3"(w1079) -> ()
                          }
                        }
                        n497 = Build Array (concatenate)(w1054, w1055) -> (w1053:u8[])
                      }
                      n498 = property on="EnableCtrls" class="Arr (strict)"(error in=w1049) -> (error out=w1047:errorcluster, "Value"=w1048:i8[][])  [unwired: 1 in, 1 out]
                      n499 = Replace Array Subset(array=w1048, new element=w1040, index (col)=1 ("disabled index (col)")) -> (w1046:i8[][])  [unwired: 1 in]
                      n500 = property on="EnableCtrls" class="Arr (strict)"(error in=w1047, "Value"=w1046) -> (error out=w1041:errorcluster)  [unwired: 1 in, 1 out]
                    }
                    frame "PhaseEnable" {
                      # "Only the three-phase and two-phase cases are the ones that matter for phase angle value, since those are the only cases with phases."
                      # "Store the enabled status given to the phase angle controls in Device(s)Settings for later retrieval. These are column indexes 6 and 7 in the array."
                      # "The Phase shift angles are only meaningful for the multiphase cases"
                      n501 = for {
                        N: 3 -> [_]
                        shift-right: [w1110] -> w1095
                        shift-left: u8[] [] -> [w1111]
                        shift-right: [w1102] -> w1096
                        shift-left: u8[] [] -> [w1103]
                        shift-right: [w1101] -> w1097
                        shift-left: w1085 -> [w1100]
                        i -> [w1106]
                        w1108 = i8[][] [[0, 0, 0], [2, 2, 2], [2, 2, 2], [2, 2, 2], [2, 2, 2], [2, 2, 2], [2, 2, 2], [2, 2, 2], [2, 2, 2], [2, 2, 2], [2, 2, 2], [2, 2, 2], [2, 2, 2], [2, 2, 2], [2, 2, 2], [2, 2, 2]]  # PhaseC AngleEnable
                        w1107 = i8[][] [[0, 0, 0], [2, 2, 2], [2, 2, 2], [2, 2, 2], [2, 2, 2], [0, 0, 2], [0, 0, 2], [2, 2, 2], [2, 2, 2], [2, 2, 2], [2, 2, 2], [2, 2, 2], [2, 2, 2], [2, 2, 2], [2, 2, 2], [2, 2, 2]]  # PhaseB AngleEnable
                        n502 = local read "Mode"() -> (w1109:T8)
                        n503 = Index Array(array=w1107, index (row)=w1109, index (col)=w1106) -> (element=w1105:i8)
                        n504 = Index Array(array=w1108, index (row)=w1109, index (col)=w1106) -> (element=w1104:i8)
                        n505 = case shown="0, Default" w1106 {
                          tunnel: w1100 -> [w1115 w1121 w1127]
                          tunnel: w1105 -> [w1117 w1123 w1129]
                          tunnel: w1104 -> [w1116 w1122 w1128]
                          tunnel: [w1112 w1118 w1124] -> w1101
                          frame 0, Default {
                            # "Instr1"
                            n506 = property on="B-Angle (Deg)" class="DigNum (strict)"(error in=w1115, "DisabledEnum"=w1117) -> (error out=w1114:errorcluster)  [unwired: 1 in, 1 out]
                            n507 = property on="C-Angle (Deg)" class="DigNum (strict)"(error in=w1115, "DisabledEnum"=w1116) -> (error out=w1113:errorcluster)  [unwired: 1 in, 1 out]
                            n508 = Merge Errors(w1114, w1113) -> (w1112:errorcluster)
                          }
                          frame 1 {
                            # "Instr2"
                            n509 = property on="B-Angle (Deg)" class="DigNum (strict)"(error in=w1121, "DisabledEnum"=w1123) -> (error out=w1120:errorcluster)  [unwired: 1 in, 1 out]
                            n510 = property on="C-Angle (Deg)" class="DigNum (strict)"(error in=w1121, "DisabledEnum"=w1122) -> (error out=w1119:errorcluster)  [unwired: 1 in, 1 out]
                            n511 = Merge Errors(w1120, w1119) -> (w1118:errorcluster)
                          }
                          frame 2 {
                            # "Instr3"
                            n512 = property on="B-Angle (Deg)" class="DigNum (strict)"(error in=w1127, "DisabledEnum"=w1129) -> (error out=w1126:errorcluster)  [unwired: 1 in, 1 out]
                            n513 = property on="C-Angle (Deg)" class="DigNum (strict)"(error in=w1127, "DisabledEnum"=w1128) -> (error out=w1125:errorcluster)  [unwired: 1 in, 1 out]
                            n514 = Merge Errors(w1126, w1125) -> (w1124:errorcluster)
                          }
                        }
                        n515 = Build Array (concatenate)(w1111, w1105) -> (w1110:u8[])
                        n516 = Build Array (concatenate)(w1104, w1103) -> (w1102:u8[])
                      }
                      n517 = property on="EnableCtrls" class="Arr (strict)"(error in=w1097) -> (error out=w1091:errorcluster, "Value"=w1092:i8[][])  [unwired: 1 in, 1 out]
                      n518 = Replace Array Subset(array=w1092, new element=w1095, index (col)=6 ("disabled index (col)")) -> (w1093:i8[][])  [unwired: 1 in]
                      n519 = Replace Array Subset(array=w1093, new element=w1096, index (col)=7 ("disabled index (col)")) -> (w1094:i8[][])  [unwired: 1 in]
                      n520 = property on="EnableCtrls" class="Arr (strict)"(error in=w1091, "Value"=w1094) -> (error out=w1084:errorcluster)  [unwired: 1 in, 1 out]
                    }
                    frame "SyncEnable" {
                      # "Store the same status given to the Synchronization controls in Device(s)Settings for later retrieval. Synchronizations are column index 2 in the array."
                      # "Synchronization settings are irrelevant for DC instruments. Enable it only for AC ones."
                      n521 = for {
                        N: 3 -> [_]
                        shift-right: [w1147] -> w1135
                        shift-left: u8[] [] -> [w1148]
                        shift-right: [w1146] -> w1139
                        shift-left: w1130 -> [w1149]
                        i -> [w1150]
                        w1151 = bool[][] [[TRUE, TRUE, TRUE], [TRUE, TRUE, TRUE], [FALSE, FALSE, FALSE], [TRUE, TRUE, TRUE], [FALSE, FALSE, FALSE], [TRUE, TRUE, TRUE], [TRUE, TRUE, FALSE], [TRUE, TRUE, TRUE], [TRUE, TRUE, FALSE], [TRUE, TRUE, FALSE], [TRUE, FALSE, FALSE], [FALSE, FALSE, TRUE], [FALSE, FALSE, FALSE], [TRUE, FALSE, TRUE], [FALSE, TRUE, TRUE], [FALSE, TRUE, FALSE]]  # Is AC?
                        n522 = local read "Mode"() -> (w1152:T8)
                        n523 = Index Array(array=w1151, index (row)=w1152, index (col)=w1150) -> (element=w1145:bool)
                        n524 = Select(t=0 ("disabled index (col)"), s=w1145, f=2 ("disabled index (col)")) -> (s? t:f=w1144:i32)
                        n525 = case shown="0, Default" w1150 {
                          tunnel: w1144 -> [w1155 w1158 w1161]
                          tunnel: w1149 -> [w1154 w1157 w1160]
                          tunnel: [w1153 w1156 w1159] -> w1146
                          frame 0, Default {
                            # "Instr1"
                            n526 = property on="Synchronization" class="Ring (strict)"(error in=w1154, "DisabledEnum"=w1155) -> (error out=w1153:errorcluster)  [unwired: 1 in, 1 out]
                          }
                          frame 1 {
                            # "Instr2"
                            n527 = property on="Synchronization" class="Ring (strict)"(error in=w1157, "DisabledEnum"=w1158) -> (error out=w1156:errorcluster)  [unwired: 1 in, 1 out]
                          }
                          frame 2 {
                            # "Instr3"
                            n528 = property on="Synchronization" class="Ring (strict)"(error in=w1160, "DisabledEnum"=w1161) -> (error out=w1159:errorcluster)  [unwired: 1 in, 1 out]
                          }
                        }
                        n529 = Build Array (concatenate)(w1148, w1144) -> (w1147:i32[])
                      }
                      n530 = property on="EnableCtrls" class="Arr (strict)"(error in=w1139) -> (error out=w1137:errorcluster, "Value"=w1138:i8[][])  [unwired: 1 in, 1 out]
                      n531 = Replace Array Subset(array=w1138, new element=w1135, index (col)=2 ("disabled index (col)")) -> (w1136:i8[][])  [unwired: 1 in]
                      n532 = property on="EnableCtrls" class="Arr (strict)"(error in=w1137, "Value"=w1136) -> (error out=w1131:errorcluster)  [unwired: 1 in, 1 out]
                    }
                    frame "ChangeEnable" {
                      w1163 = T15."Disabled and Grayed Out" ("Disabled")
                      w1183 = 0 ("Value")
                      w1188 = 0 ("Value")
                      w1189 = 0 ("Value")
                      # "Store the same status given to the 'Change at' controls in Device(s)Settings for later retrieval. Changes are column indexes 8, 9, & 10 in the array."
                      # "Since all instruments were set to have Synchronization as \"Immediate\" by default, the angle setting doesn't need to be used until the user either selects \"Sync\" or \"Synct to Phase A\" later to set the values. Therefore, have them all initially disabled."
                      # "Initialize all changes to 0 degrees"
                      # "\"Change at\" is only used for AC instruments, but by default all instruments will have their controls disabled."
                      n533 = property on="A-Change at..." class="DigNum (strict)"(error in=w1174, "DisabledEnum"=w1163) -> (error out=w1175:errorcluster)  [unwired: 1 in, 1 out]
                      n534 = local read "Instr1"() -> (w1190:T2)
                      n535 = Bundle By Name(cluster=w1190, "Phases.A-Change at..."=w1189, "Phases.B-Change at..."=w1189, "Phases.C-Change at..."=w1189) -> (w1191:T2)
                      n536 = property on="B-Change at..." class="DigNum (strict)"(error in=w1175, "DisabledEnum"=w1163) -> (error out=w1176:errorcluster)  [unwired: 1 in, 1 out]
                      n537 = property on="C-Change at..." class="DigNum (strict)"(error in=w1176, "DisabledEnum"=w1163) -> (error out=w1177:errorcluster)  [unwired: 1 in, 1 out]
                      n538 = local write "Instr1"(w1191) -> ()
                      n539 = property on="A-Change at..." class="DigNum (strict)"(error in=w1177, "DisabledEnum"=w1163) -> (error out=w1178:errorcluster)  [unwired: 1 in, 1 out]
                      n540 = local read "Instr2"() -> (w1187:T2)
                      n541 = Bundle By Name(cluster=w1187, "Phases.A-Change at..."=w1188, "Phases.B-Change at..."=w1188, "Phases.C-Change at..."=w1188) -> (w1186:T2)
                      n542 = property on="B-Change at..." class="DigNum (strict)"(error in=w1178, "DisabledEnum"=w1163) -> (error out=w1179:errorcluster)  [unwired: 1 in, 1 out]
                      n543 = property on="C-Change at..." class="DigNum (strict)"(error in=w1179, "DisabledEnum"=w1163) -> (error out=w1180:errorcluster)  [unwired: 1 in, 1 out]
                      n544 = local write "Instr2"(w1186) -> ()
                      n545 = property on="A-Change at..." class="DigNum (strict)"(error in=w1180, "DisabledEnum"=w1163) -> (error out=w1181:errorcluster)  [unwired: 1 in, 1 out]
                      n546 = local read "Instr3"() -> (w1184:T2)
                      n547 = Bundle By Name(cluster=w1184, "Phases.A-Change at..."=w1183, "Phases.B-Change at..."=w1183, "Phases.C-Change at..."=w1183) -> (w1185:T2)
                      n548 = property on="B-Change at..." class="DigNum (strict)"(error in=w1181, "DisabledEnum"=w1163) -> (error out=w1182:errorcluster)  [unwired: 1 in, 1 out]
                      n549 = property on="C-Change at..." class="DigNum (strict)"(error in=w1182, "DisabledEnum"=w1163) -> (error out=w1164:errorcluster)  [unwired: 1 in, 1 out]
                      n550 = local write "Instr3"(w1185) -> ()
                      n551 = Build Array(w1163, w1163, w1163) -> (w1162:T21)
                      n552 = property on="EnableCtrls" class="Arr (strict)"(error in=w1164) -> (error out=w1170:errorcluster, "Value"=w1169:i8[][])  [unwired: 1 in, 1 out]
                      n553 = Replace Array Subset(array=w1169, new element=w1162, index (col)=8 ("disabled index (col)")) -> (w1171:i8[][])  [unwired: 1 in]
                      n554 = Replace Array Subset(array=w1171, new element=w1162, index (col)=9 ("disabled index (col)")) -> (w1172:i8[][])  [unwired: 1 in]
                      n555 = Replace Array Subset(array=w1172, new element=w1162, index (col)=10 ("disabled index (col)")) -> (w1173:i8[][])  [unwired: 1 in]
                      n556 = property on="EnableCtrls" class="Arr (strict)"(error in=w1170, "Value"=w1173) -> (error out=w1165:errorcluster)  [unwired: 1 in, 1 out]
                    }
                    frame "VoltsEnable" {
                      # "Only the three-phase and two-phase cases are the ones that matter for phase voltage value, since those are the only cases with phases. In terms of voltages, the three-phase and two-phase cases always need phases A and B, so they have the same settings. But phase C is not needed for the two-phase."
                      # "Store the enabled status given to the phase voltage controls in Device(s)Settings for later retrieval. These are column indexes 3, 4 and 5 in the array."
                      # "Phase voltages should be used only for multi-phase Modes"
                      n557 = for {
                        N: 3 -> [_]
                        shift-right: [w1222] -> w1209
                        shift-left: u8[] [] -> [w1223]
                        shift-right: [w1216] -> w1205
                        shift-left: u8[] [] -> [w1217]
                        shift-right: [w1215] -> w1206
                        shift-left: w1194 -> [w1214]
                        i -> [w1220]
                        w1212 = i8[][] [[0, 0, 0], [2, 2, 2], [2, 2, 2], [2, 2, 2], [2, 2, 2], [0, 0, 2], [0, 0, 2], [2, 2, 2], [2, 2, 2], [2, 2, 2], [2, 2, 2], [2, 2, 2], [2, 2, 2], [2, 2, 2], [2, 2, 2], [2, 2, 2]]  # PhaseA/B VoltsEnable
                        w1213 = i8[][] [[0, 0, 0], [2, 2, 2], [2, 2, 2], [2, 2, 2], [2, 2, 2], [2, 2, 2], [2, 2, 2], [2, 2, 2], [2, 2, 2], [2, 2, 2], [2, 2, 2], [2, 2, 2], [2, 2, 2], [2, 2, 2], [2, 2, 2], [2, 2, 2]]  # PhaseC VoltsEnable
                        n558 = local read "Mode"() -> (w1221:T8)
                        n559 = Index Array(array=w1212, index (row)=w1221, index (col)=w1220) -> (element=w1219:i8)
                        n560 = Index Array(array=w1213, index (row)=w1221, index (col)=w1220) -> (element=w1218:i8)
                        n561 = case shown="2" w1220 {
                          tunnel: w1214 -> [w1226 w1233 w1240]
                          tunnel: w1219 -> [w1224 w1231 w1238]
                          tunnel: w1218 -> [w1225 w1232 w1239]
                          tunnel: [w1229 w1236 w1243] -> w1215
                          frame 0, Default {
                            # "Instr1"
                            n562 = property on="A-Volts (V)" class="DigNum (strict)"(error in=w1226, "DisabledEnum"=w1224) -> (error out=w1230:errorcluster)  [unwired: 1 in, 1 out]
                            n563 = property on="B-Volts (V)" class="DigNum (strict)"(error in=w1226, "DisabledEnum"=w1224) -> (error out=w1228:errorcluster)  [unwired: 1 in, 1 out]
                            n564 = property on="C-Volts (V)" class="DigNum (strict)"(error in=w1226, "DisabledEnum"=w1225) -> (error out=w1227:errorcluster)  [unwired: 1 in, 1 out]
                            n565 = Merge Errors(w1230, w1228, w1227) -> (w1229:errorcluster)
                          }
                          frame 1 {
                            # "Instr2"
                            n566 = property on="A-Volts (V)" class="DigNum (strict)"(error in=w1233, "DisabledEnum"=w1231) -> (error out=w1237:errorcluster)  [unwired: 1 in, 1 out]
                            n567 = property on="B-Volts (V)" class="DigNum (strict)"(error in=w1233, "DisabledEnum"=w1231) -> (error out=w1235:errorcluster)  [unwired: 1 in, 1 out]
                            n568 = property on="C-Volts (V)" class="DigNum (strict)"(error in=w1233, "DisabledEnum"=w1232) -> (error out=w1234:errorcluster)  [unwired: 1 in, 1 out]
                            n569 = Merge Errors(w1237, w1235, w1234) -> (w1236:errorcluster)
                          }
                          frame 2 {
                            # "Instr3"
                            n570 = property on="A-Volts (V)" class="DigNum (strict)"(error in=w1240, "DisabledEnum"=w1238) -> (error out=w1244:errorcluster)  [unwired: 1 in, 1 out]
                            n571 = property on="B-Volts (V)" class="DigNum (strict)"(error in=w1240, "DisabledEnum"=w1238) -> (error out=w1242:errorcluster)  [unwired: 1 in, 1 out]
                            n572 = property on="C-Volts (V)" class="DigNum (strict)"(error in=w1240, "DisabledEnum"=w1239) -> (error out=w1241:errorcluster)  [unwired: 1 in, 1 out]
                            n573 = Merge Errors(w1244, w1242, w1241) -> (w1243:errorcluster)
                          }
                        }
                        n574 = Build Array (concatenate)(w1223, w1219) -> (w1222:u8[])
                        n575 = Build Array (concatenate)(w1218, w1217) -> (w1216:u8[])
                      }
                      n576 = property on="EnableCtrls" class="Arr (strict)"(error in=w1206) -> (error out=w1202:errorcluster, "Value"=w1203:i8[][])  [unwired: 1 in, 1 out]
                      n577 = Replace Array Subset(array=w1203, new element=w1209, index (col)=3 ("disabled index (col)")) -> (w1207:i8[][])  [unwired: 1 in]
                      n578 = Replace Array Subset(array=w1207, new element=w1209, index (col)=4 ("disabled index (col)")) -> (w1208:i8[][])  [unwired: 1 in]
                      n579 = Replace Array Subset(array=w1208, new element=w1205, index (col)=5 ("disabled index (col)")) -> (w1204:i8[][])  [unwired: 1 in]
                      n580 = property on="EnableCtrls" class="Arr (strict)"(error in=w1202, "Value"=w1204) -> (error out=w1195:errorcluster)  [unwired: 1 in, 1 out]
                    }
                    frame "Vtype" {
                      # "Notify the user about the instrument voltage reference for the Vout value"
                      n581 = local read "Mode"() -> (w1247:T8)
                      n582 = case shown="0, 5, 6" w1247 {
                        selector: w1247 -> [w1252 _]
                        tunnel: w1246 -> [w1250 w1262]
                        tunnel: [w1250 w1262] -> w1245
                        frame 0, 5, 6 {
                          w1254 = "(L-L)" ("element")
                          # "For two-phase cases Instr3 has no phases."
                          # "Multiphase cases have Vout as Line-to-Line between phases"
                          n583 = Equal To 0?(x=w1252) -> (x = 0?=w1255:bool)
                          n584 = Select(t=w1254, s=w1255, f="(L-N)" ("element")) -> (s? t:f=w1253:string)
                          n585 = local read "Instr1"() -> (w1260:T2)
                          n586 = local read "Instr2"() -> (w1259:T2)
                          n587 = local read "Instr3"() -> (w1256:T2)
                          n588 = Bundle By Name(cluster=w1260, "VType"=w1254) -> (w1261:T2)
                          n589 = Bundle By Name(cluster=w1259, "VType"=w1254) -> (w1258:T2)
                          n590 = Bundle By Name(cluster=w1256, "VType"=w1253) -> (w1257:T2)
                          n591 = local write "Instr1"(w1261) -> ()
                          n592 = local write "Instr2"(w1258) -> ()
                          n593 = local write "Instr3"(w1257) -> ()
                        }
                        frame Default {
                          w1263 = "(L-N)" ("element")
                          # "For all other instances Vout is Line-to-Neutral"
                          n594 = local read "Instr1"() -> (w1268:T2)
                          n595 = local read "Instr2"() -> (w1267:T2)
                          n596 = local read "Instr3"() -> (w1264:T2)
                          n597 = Bundle By Name(cluster=w1268, "VType"=w1263) -> (w1269:T2)
                          n598 = Bundle By Name(cluster=w1267, "VType"=w1263) -> (w1266:T2)
                          n599 = Bundle By Name(cluster=w1264, "VType"=w1263) -> (w1265:T2)
                          n600 = local write "Instr1"(w1269) -> ()
                          n601 = local write "Instr2"(w1266) -> ()
                          n602 = local write "Instr3"(w1265) -> ()
                        }
                      }
                    }
                    frame "Description" {
                      # "Give a better description of the instrument in its Tab caption than the default Instrumnet name"
                      n603 = property on="Instruments" class="TabCtl (strict)"(error in=w1280) -> (error out=w1279:errorcluster, "Pages"=w1282:refnum<vi>[])  [unwired: 1 in, 1 out]
                      n604 = local read "Mode"() -> (w1281:T8)
                      n605 = for {
                        tunnel: w1282 -> [w1291] mode=indexing
                        tunnel: w1281 -> [w1292]
                        shift-right: [w1288] -> w1272
                        shift-left: w1279 -> [w1289]
                        tunnel: "Three-Phase AC" ("element") -> [w1287]
                        tunnel: "One-Phase AC" ("element") -> [w1286]
                        tunnel: "DC Source" ("element") -> [w1285]
                        tunnel: "Two-Phase AC" ("element") -> [w1284]
                        tunnel: [w1283] -> w1270 mode=indexing
                        i -> [w1290]
                        n606 = case shown="8" w1292 {
                          tunnel: w1291 -> [w1300 w1308 w1316 w1324 w1332 w1347 w1362 w1377 w1392 w1405 w1418 w1431 w1444 w1457 w1470 w1483]
                          tunnel: w1290 -> [_ _ _ _ _ w1343 w1358 w1373 w1388 w1398 w1410 w1423 w1437 w1446 w1459 w1472]
                          tunnel: w1289 -> [w1299 w1307 w1315 w1323 w1331 w1346 w1361 w1376 w1391 w1404 w1417 w1430 w1443 w1456 w1469 w1482]
                          tunnel: [w1298 w1306 w1314 w1322 w1330 w1345 w1360 w1375 w1390 w1403 w1416 w1429 w1442 w1455 w1468 w1481] -> w1288
                          tunnel: w1287 -> [w1295 _ _ _ _ _ _ _ _ _ _ _ _ _ _ _]
                          tunnel: w1286 -> [_ w1303 _ w1319 _ w1338 w1353 _ w1379 w1395 w1413 w1427 _ w1452 w1465 w1479]
                          tunnel: w1285 -> [_ _ w1310 _ w1326 _ w1349 w1364 w1380 _ w1414 w1426 w1433 w1453 w1466 w1478]
                          tunnel: w1284 -> [_ _ _ _ _ w1335 _ w1366 _ _ _ _ _ _ _ _]
                          tunnel: [w1293 w1301 w1309 w1317 w1325 w1333 w1348 w1363 w1378 w1393 w1406 w1419 w1432 w1445 w1458 w1471] -> w1283
                          frame 0, Default {
                            # "Three-Phase AC1"
                            n607 = Concatenate Strings(w1295, " (3Ch)" ("string")) -> (w1296:string)
                            n608 = property class="Page"(reference=w1300, error in=w1299, "IndependentLabel"=TRUE ("Independent Label"), "TabCaption"=w1296) -> (reference out=w1293:refnum<vi>, error out=w1298:errorcluster)
                          }
                          frame 1 {
                            # "AC1 using three channels as single phase"
                            n609 = Concatenate Strings(w1303, " (3Ch)" ("string")) -> (w1302:string)
                            n610 = property class="Page"(reference=w1308, error in=w1307, "TabCaption"=w1302, "IndependentLabel"=TRUE ("Independent Label")) -> (reference out=w1301:refnum<vi>, error out=w1306:errorcluster)
                          }
                          frame 2 {
                            # "DC1 using all three channels as single source"
                            n611 = Concatenate Strings(w1310, " (3Ch)" ("string")) -> (w1311:string)
                            n612 = property class="Page"(reference=w1316, error in=w1315, "TabCaption"=w1311, "IndependentLabel"=TRUE ("Independent Label")) -> (reference out=w1309:refnum<vi>, error out=w1314:errorcluster)
                          }
                          frame 3 {
                            # "AC1 - AC2 - AC3"
                            n613 = Concatenate Strings(w1319, " (1Ch)" ("string")) -> (w1318:string)
                            n614 = property class="Page"(reference=w1324, error in=w1323, "TabCaption"=w1318, "IndependentLabel"=TRUE ("Independent Label")) -> (reference out=w1317:refnum<vi>, error out=w1322:errorcluster)
                          }
                          frame 4 {
                            # "DC1- DC2- DC3"
                            n615 = Concatenate Strings(w1326, " (1Ch)" ("string")) -> (w1327:string)
                            n616 = property class="Page"(reference=w1332, error in=w1331, "TabCaption"=w1327, "IndependentLabel"=TRUE ("Independent Label")) -> (reference out=w1325:refnum<vi>, error out=w1330:errorcluster)
                          }
                          frame 5 {
                            # "AC1 Two-phase and AC3"
                            n617 = Equal?(x=w1343, y=2 ("x")) -> (x = y?=w1334:bool)
                            n618 = Concatenate Strings(w1338, " (1Ch)" ("string")) -> (w1340:string)
                            n619 = Concatenate Strings(w1335, " (2Ch)" ("string")) -> (w1337:string)
                            n620 = Select(t=w1340, s=w1334, f=w1337) -> (s? t:f=w1341:string)
                            n621 = property class="Page"(reference=w1347, error in=w1346, "TabCaption"=w1341, "IndependentLabel"=TRUE ("Independent Label")) -> (reference out=w1333:refnum<vi>, error out=w1345:errorcluster)
                          }
                          frame 11 {
                            # "DC1 with two channels and AC3"
                            n622 = Equal?(x=w1358, y=2 ("x")) -> (x = y?=w1350:bool)
                            n623 = Concatenate Strings(w1353, " (1Ch)" ("string")) -> (w1355:string)
                            n624 = Concatenate Strings(w1349, " (2Ch)" ("string")) -> (w1352:string)
                            n625 = Select(t=w1355, s=w1350, f=w1352) -> (s? t:f=w1356:string)
                            n626 = property class="Page"(reference=w1362, error in=w1361, "TabCaption"=w1356, "IndependentLabel"=TRUE ("Independent Label")) -> (reference out=w1348:refnum<vi>, error out=w1360:errorcluster)
                          }
                          frame 6 {
                            # "Ac1 Two-pahse and DC3"
                            n627 = Equal?(x=w1373, y=2 ("x")) -> (x = y?=w1365:bool)
                            n628 = Concatenate Strings(w1364, " (1Ch)" ("string")) -> (w1370:string)
                            n629 = Concatenate Strings(w1366, " (2Ch)" ("string")) -> (w1368:string)
                            n630 = Select(t=w1370, s=w1365, f=w1368) -> (s? t:f=w1371:string)
                            n631 = property class="Page"(reference=w1377, error in=w1376, "TabCaption"=w1371, "IndependentLabel"=TRUE ("Independent Label")) -> (reference out=w1363:refnum<vi>, error out=w1375:errorcluster)
                          }
                          frame 8 {
                            # "AC1 two channels as single phase and DC3"
                            n632 = Equal?(x=w1388, y=2 ("x")) -> (x = y?=w1381:bool)
                            n633 = Concatenate Strings(w1380, " (1Ch)" ("string")) -> (w1385:string)
                            n634 = Concatenate Strings(w1379, " (2Ch)" ("string")) -> (w1383:string)
                            n635 = Select(t=w1385, s=w1381, f=w1383) -> (s? t:f=w1386:string)
                            n636 = property class="Page"(reference=w1392, error in=w1391, "TabCaption"=w1386, "IndependentLabel"=TRUE ("Independent Label")) -> (reference out=w1378:refnum<vi>, error out=w1390:errorcluster)
                          }
                          frame 7 {
                            # "AC1 two channels as single phase and AC3"
                            n637 = Equal?(x=w1398, y=2 ("x")) -> (x = y?=w1401:bool)
                            n638 = Select(t=" (1Ch)" ("string"), s=w1401, f=" (2Ch)" ("string")) -> (s? t:f=w1394:string)
                            n639 = Concatenate Strings(w1395, w1394) -> (w1396:string)
                            n640 = property class="Page"(reference=w1405, error in=w1404, "TabCaption"=w1396, "IndependentLabel"=TRUE ("Independent Label")) -> (reference out=w1393:refnum<vi>, error out=w1403:errorcluster)
                          }
                          frame 9 {
                            # "AC1 - AC2 - DC3"
                            n641 = Equal?(x=w1410, y=2 ("x")) -> (x = y?=w1415:bool)
                            n642 = Select(t=w1414, s=w1415, f=w1413) -> (s? t:f=w1408:string)
                            n643 = Concatenate Strings(w1408, " (1Ch)" ("string")) -> (w1407:string)
                            n644 = property class="Page"(reference=w1418, error in=w1417, "TabCaption"=w1407, "IndependentLabel"=TRUE ("Independent Label")) -> (reference out=w1406:refnum<vi>, error out=w1416:errorcluster)
                          }
                          frame 10 {
                            # "AC1 - DC2 - DC3"
                            n645 = Equal?(x=w1423, y=0 ("x")) -> (x = y?=w1428:bool)
                            n646 = Select(t=w1427, s=w1428, f=w1426) -> (s? t:f=w1420:string)
                            n647 = Concatenate Strings(w1420, " (1Ch)" ("string")) -> (w1421:string)
                            n648 = property class="Page"(reference=w1431, error in=w1430, "TabCaption"=w1421, "IndependentLabel"=TRUE ("Independent Label")) -> (reference out=w1419:refnum<vi>, error out=w1429:errorcluster)
                          }
                          frame 12 {
                            # "DC1 in two channels and DC3"
                            n649 = Equal?(x=w1437, y=2 ("x")) -> (x = y?=w1440:bool)
                            n650 = Select(t=" (1Ch)" ("string"), s=w1440, f=" (2Ch)" ("string")) -> (s? t:f=w1434:string)
                            n651 = Concatenate Strings(w1433, w1434) -> (w1435:string)
                            n652 = property class="Page"(reference=w1444, error in=w1443, "TabCaption"=w1435, "IndependentLabel"=TRUE ("Independent Label")) -> (reference out=w1432:refnum<vi>, error out=w1442:errorcluster)
                          }
                          frame 13 {
                            # "AC1 - DC2 - AC3"
                            n653 = Equal?(x=w1446, y=1 ("x")) -> (x = y?=w1454:bool)
                            n654 = Select(t=w1453, s=w1454, f=w1452) -> (s? t:f=w1448:string)
                            n655 = Concatenate Strings(w1448, " (1Ch)" ("string")) -> (w1449:string)
                            n656 = property class="Page"(reference=w1457, error in=w1456, "TabCaption"=w1449, "IndependentLabel"=TRUE ("Independent Label")) -> (reference out=w1445:refnum<vi>, error out=w1455:errorcluster)
                          }
                          frame 14 {
                            # "DC1 - AC2 - AC3"
                            n657 = Equal?(x=w1459, y=0 ("x")) -> (x = y?=w1467:bool)
                            n658 = Select(t=w1466, s=w1467, f=w1465) -> (s? t:f=w1461:string)
                            n659 = Concatenate Strings(w1461, " (1Ch)" ("string")) -> (w1462:string)
                            n660 = property class="Page"(reference=w1470, error in=w1469, "TabCaption"=w1462, "IndependentLabel"=TRUE ("Independent Label")) -> (reference out=w1458:refnum<vi>, error out=w1468:errorcluster)
                          }
                          frame 15 {
                            # "DC1 - AC2 - DC3"
                            n661 = Equal?(x=w1472, y=1 ("x")) -> (x = y?=w1480:bool)
                            n662 = Select(t=w1479, s=w1480, f=w1478) -> (s? t:f=w1474:string)
                            n663 = Concatenate Strings(w1474, " (1Ch)" ("string")) -> (w1475:string)
                            n664 = property class="Page"(reference=w1483, error in=w1482, "TabCaption"=w1475, "IndependentLabel"=TRUE ("Independent Label")) -> (reference out=w1471:refnum<vi>, error out=w1481:errorcluster)
                          }
                        }
                      }
                      n665 = Close Reference(reference=w1270, error in (no error)=w1272) -> (error out=w1271:errorcluster)
                    }
                    frame "CurrRanges" {
                      w1491 = i8[][] [[1, 1, 1], [3, 3, 3], [3, 3, 3], [1, 1, 1], [1, 1, 1], [1, 1, 1], [1, 1, 1], [2, 2, 1], [2, 2, 1], [1, 1, 1], [1, 1, 1], [2, 2, 1], [2, 2, 1], [1, 1, 1], [1, 1, 1], [1, 1, 1]]  # CRangeMultiple
                      # "The frame ensures that this is done after placing the midified strings with the current limits in their controls first, and before updating the values of Device(s)Settings."
                      # "All instrumenst have the same two basic current range limits: 6A and 30A. But the actual values displayed to the user will vary not only depending on mode, but they also depend on the number of chassis turned on in the device. Determine the correct values and populate the control option list. \nNote: The chassis contribution is accounted for only when the device is \"Connected\"."
                      # "Set range value to the maximum."
                      # "Multiphase, single phase, and DC instruments have different current ranges"
                      n666 = local read "Mode"() -> (w1494:T8)
                      n667 = local read "Chassis"() -> (w1505:i32)
                      n668 = Index Array(array=w1491, index (row) #1=w1494, index (col) #1=0 ("disabled index (col)"), index (row) #2=w1494, index (col) #2=1 ("disabled index (col)"), index (row) #3=w1494, index (col) #3=2 ("disabled index (col)")) -> (element #1=w1504:i8, element #2=w1503:i8, element #3=w1502:i8)
                      n669 = Build Array(6, 30) -> (w1495:i32[])
                      n670 = Multiply(x=w1505, y=w1504) -> (x*y=w1499:i32)
                      n671 = Multiply(x=w1505, y=w1502) -> (x*y=w1501:i32)
                      n672 = Multiply(x=w1505, y=w1503) -> (x*y=w1500:i32)
                      n673 = Multiply(x=w1495, y=w1499) -> (x*y=w1496:i32[])
                      n674 = Multiply(x=w1495, y=w1501) -> (x*y=w1498:i32[])
                      n675 = Multiply(x=w1495, y=w1500) -> (x*y=w1497:i32[])
                      n676 = call "num2str.vi"("NumArray"=w1496) -> ("StrArray"=w1486:string[])  [unwired: 10 in]
                      n677 = call "num2str.vi"("NumArray"=w1497) -> ("StrArray"=w1485:string[])  [unwired: 10 in]
                      n678 = call "num2str.vi"("NumArray"=w1498) -> ("StrArray"=w1484:string[])  [unwired: 10 in]
                      n679 = property on="Current (A)" class="Ring (strict)"(error in=w1487, "Strings []"=w1486) -> (error out=w1509:errorcluster)  [unwired: 1 in, 1 out]
                      n680 = property on="Current (A)" class="Ring (strict)"(error in=w1509, "Strings []"=w1485) -> (error out=w1510:errorcluster)  [unwired: 1 in, 1 out]
                      n681 = property on="Current (A)" class="Ring (strict)"(error in=w1510, "Strings []"=w1484) -> (error out=w1507:errorcluster)  [unwired: 1 in, 1 out]
                      n682 = flat-sequence {
                        tunnel: u16 1 ("Ranges.Current (A)") -> [w1514]
                        tunnel: [w1513] -> w1506
                        tunnel: w1507 -> [w1513]
                        frame #0 {
                          n683 = local read "Instr1"() -> (w1519:T2)
                          n684 = Bundle By Name(cluster=w1519, "Ranges.Current (A)"=w1514) -> (w1520:T2)
                          n685 = local read "Instr2"() -> (w1518:T2)
                          n686 = Bundle By Name(cluster=w1518, "Ranges.Current (A)"=w1514) -> (w1517:T2)
                          n687 = local read "Instr3"() -> (w1515:T2)
                          n688 = Bundle By Name(cluster=w1515, "Ranges.Current (A)"=w1514) -> (w1516:T2)
                          n689 = local write "Instr1"(w1520) -> ()
                          n690 = local write "Instr2"(w1517) -> ()
                          n691 = local write "Instr3"(w1516) -> ()
                        }
                      }
                    }
                    frame "VoutCoerce" {
                      # "Ensure that user can not set Vout more than Vrange maximum of the selected Mode"
                      n692 = for {
                        N: 3 -> [_]
                        shift-right: [w1526] -> w1521
                        shift-left: w1522 -> [w1527]
                        i -> [w1528]
                        n693 = case shown="0, Default" w1528 {
                          tunnel: w1527 -> [w1530 w1539 w1548]
                          tunnel: [w1529 w1538 w1547] -> w1526
                          frame 0, Default {
                            # "Turn string to numeric"
                            # "Then coerce the Vout control so that the maximum value that the user could enter can only be up to the maximum value allowed by the range."
                            # "Extract the maximum (string) value of the V range"
                            # "1=Coerce"
                            # "Instr1"
                            n694 = property on="Voltage (V)" class="Ring (strict)"(error in=w1530) -> (error out=w1533:errorcluster, "Strings []"=w1532:string[])  [unwired: 1 in, 1 out]
                            n695 = Array Max & Min(array=w1532) -> (max value=w1534:string)  [unwired: 3 out]
                            n696 = Scan From String(format string="%d", input string=w1534, error in=w1533) -> (error out=w1537:errorcluster, output 1=w1535:i32)  [unwired: 2 in, 2 out]
                            n697 = property on="Vout (V)" class="DigNum (strict)"(error in=w1537, "Maximum"=w1535, "OutOfRngActMax"=u8 1 ("Response to Value Outside Limits:Maximum")) -> (error out=w1529:errorcluster)  [unwired: 1 in, 1 out]
                          }
                          frame 1 {
                            # "Turn string to numeric"
                            # "Then coerce the Vout control so that the maximum value that the user could enter can only be up to the maximum value allowed by the range."
                            # "Extract the maximum (string) value of the V range"
                            # "1=Coerce"
                            # "Instr2"
                            n698 = property on="Voltage (V)" class="Ring (strict)"(error in=w1539) -> (error out=w1542:errorcluster, "Strings []"=w1541:string[])  [unwired: 1 in, 1 out]
                            n699 = Array Max & Min(array=w1541) -> (max value=w1543:string)  [unwired: 3 out]
                            n700 = Scan From String(format string="%d", input string=w1543, error in=w1542) -> (error out=w1546:errorcluster, output 1=w1544:i32)  [unwired: 2 in, 2 out]
                            n701 = property on="Vout (V)" class="DigNum (strict)"(error in=w1546, "Maximum"=w1544, "OutOfRngActMax"=u8 1 ("Response to Value Outside Limits:Maximum")) -> (error out=w1538:errorcluster)  [unwired: 1 in, 1 out]
                          }
                          frame 2 {
                            # "Turn string to numeric"
                            # "Then coerce the Vout control so that the maximum value that the user could enter can only be up to the maximum value allowed by the range."
                            # "Extract the maximum (string) value of the V range"
                            # "1=Coerce"
                            # "Instr3"
                            n702 = property on="Voltage (V)" class="Ring (strict)"(error in=w1548) -> (error out=w1551:errorcluster, "Strings []"=w1550:string[])  [unwired: 1 in, 1 out]
                            n703 = Array Max & Min(array=w1550) -> (max value=w1552:string)  [unwired: 3 out]
                            n704 = Scan From String(format string="%d", input string=w1552, error in=w1551) -> (error out=w1555:errorcluster, output 1=w1553:i32)  [unwired: 2 in, 2 out]
                            n705 = property on="Vout (V)" class="DigNum (strict)"(error in=w1555, "Maximum"=w1553, "OutOfRngActMax"=u8 1 ("Response to Value Outside Limits:Maximum")) -> (error out=w1547:errorcluster)  [unwired: 1 in, 1 out]
                          }
                        }
                      }
                    }
                    frame "VSlewCoerce" {
                      # "Voltage slew limits depend on Mode. All AC and DC instruments can modify the Voltage Slew control in the user interface."
                      n706 = for {
                        N: 3 -> [_]
                        shift-right: [w1561] -> w1556
                        shift-left: w1557 -> [w1562]
                        i -> [w1563]
                        n707 = case shown="0, Default" w1563 {
                          tunnel: w1562 -> [w1565 w1577 w1588]
                          tunnel: [w1564 w1576 w1587] -> w1561
                          frame 0, Default {
                            w1566 = u8 1 ("Response to Value Outside Limits:Maximum")
                            w1570 = dbl[][] [[0.0173, 866030.0, 1730000.0], [0.01, 500000.0, 1000000.0], [0.01, 20000.0, 20000.0], [0.01, 500000.0, 1000000.0], [0.01, 20000.0, 20000.0], [0.02, 1000000.0, 2000000.0], [0.02, 1000000.0, 2000000.0], [0.01, 500000.0, 1000000.0], [0.01, 500000.0, 1000000.0], [0.01, 500000.0, 1000000.0], [0.01, 500000.0, 1000000.0], [0.01, 20000.0, 20000.0], [0.01, 20000.0, 20000.0], [0.01, 500000.0, 1000000.0], [0.01, 20000.0, 20000.0], [0.01, 20000.0, 20000.0]]  # V Slew 1
                            # "1 = Coerce"
                            # "Instr1"
                            n708 = local read "Mode"() -> (w1571:T8)
                            n709 = Index Array(array=w1570, index (row) #1=w1571, index (col) #1=0 ("disabled index (col)"), index (row) #2=w1571, index (col) #2=1 ("disabled index (col)"), index (row) #3=w1571, index (col) #3=2 ("disabled index (col)")) -> (element #1=w1572:dbl, element #2=w1573:dbl, element #3=w1574:dbl)
                            n710 = property on="Voltage (V/s)" class="DigNum (strict)"(error in=w1565, "Minimum"=w1572, "Value"=w1573, "Maximum"=w1574, "OutOfRngActMin"=w1566, "OutOfRngActMax"=w1566) -> (error out=w1564:errorcluster)  [unwired: 1 in, 1 out]
                          }
                          frame 1 {
                            w1575 = dbl[][] [[0.0173, 866030.0, 1730000.0], [0.01, 500000.0, 1000000.0], [0.01, 20000.0, 20000.0], [0.01, 500000.0, 1000000.0], [0.01, 20000.0, 20000.0], [0.02, 1000000.0, 2000000.0], [0.02, 1000000.0, 2000000.0], [0.01, 500000.0, 1000000.0], [0.01, 500000.0, 1000000.0], [0.01, 500000.0, 1000000.0], [0.01, 20000.0, 20000.0], [0.01, 20000.0, 20000.0], [0.01, 20000.0, 20000.0], [0.01, 20000.0, 20000.0], [0.01, 500000.0, 1000000.0], [0.01, 500000.0, 1000000.0]]  # V Slew 2
                            w1578 = u8 1 ("Response to Value Outside Limits:Maximum")
                            # "Instr2"
                            n711 = local read "Mode"() -> (w1582:T8)
                            n712 = Index Array(array=w1575, index (row) #1=w1582, index (col) #1=0 ("disabled index (col)"), index (row) #2=w1582, index (col) #2=1 ("disabled index (col)"), index (row) #3=w1582, index (col) #3=2 ("disabled index (col)")) -> (element #1=w1583:dbl, element #2=w1584:dbl, element #3=w1585:dbl)
                            n713 = property on="Voltage (V/s)" class="DigNum (strict)"(error in=w1577, "Minimum"=w1583, "Value"=w1584, "Maximum"=w1585, "OutOfRngActMin"=w1578, "OutOfRngActMax"=w1578) -> (error out=w1576:errorcluster)  [unwired: 1 in, 1 out]
                          }
                          frame 2 {
                            w1586 = dbl[][] [[0.0173, 866030.0, 1730000.0], [0.01, 500000.0, 1000000.0], [0.01, 20000.0, 20000.0], [0.01, 500000.0, 1000000.0], [0.01, 20000.0, 20000.0], [0.01, 500000.0, 1000000.0], [0.01, 20000.0, 20000.0], [0.01, 500000.0, 1000000.0], [0.01, 20000.0, 20000.0], [0.01, 20000.0, 20000.0], [0.01, 20000.0, 20000.0], [0.01, 500000.0, 1000000.0], [0.01, 20000.0, 20000.0], [0.01, 500000.0, 1000000.0], [0.01, 500000.0, 1000000.0], [0.01, 20000.0, 20000.0]]  # V Slew 3
                            w1589 = u8 1 ("Response to Value Outside Limits:Maximum")
                            # "Instr3"
                            n714 = local read "Mode"() -> (w1593:T8)
                            n715 = Index Array(array=w1586, index (row) #1=w1593, index (col) #1=0 ("disabled index (col)"), index (row) #2=w1593, index (col) #2=1 ("disabled index (col)"), index (row) #3=w1593, index (col) #3=2 ("disabled index (col)")) -> (element #1=w1594:dbl, element #2=w1595:dbl, element #3=w1596:dbl)
                            n716 = property on="Voltage (V/s)" class="DigNum (strict)"(error in=w1588, "Minimum"=w1594, "Value"=w1595, "Maximum"=w1596, "OutOfRngActMin"=w1589, "OutOfRngActMax"=w1589) -> (error out=w1587:errorcluster)  [unwired: 1 in, 1 out]
                          }
                        }
                      }
                    }
                    frame "CSlewCoerce" {
                      # "All instrument channels have the same base Current Slew values [Min=0.2, Def=100k, Max=100k] but they depend on how many channels are combined together and how many Chassis are on."
                      # "Current slew limits depend on Mode. Current Slew is used for DC instruments."
                      n717 = for {
                        N: 3 -> [_]
                        shift-right: [w1602] -> w1599
                        shift-left: w1598 -> [w1603]
                        i -> [w1604]
                        n718 = case shown="1" w1604 {
                          selector: w1604 -> [w1605 w1620 w1635]
                          tunnel: w1603 -> [w1617 w1632 w1647]
                          tunnel: [w1616 w1631 w1646] -> w1602
                          frame 0, Default {
                            w1615 = i32[][] [[1, 1, 1], [3, 3, 3], [3, 3, 3], [1, 1, 1], [1, 1, 1], [1, 1, 1], [1, 1, 1], [2, 2, 1], [2, 2, 1], [1, 1, 1], [1, 1, 1], [2, 2, 1], [2, 2, 1], [1, 1, 1], [1, 1, 1], [1, 1, 1]]  # Ch Multiple
                            w1611 = 100000.0
                            # "Instr1"
                            n719 = local read "Mode"() -> (w1619:T8)
                            n720 = local read "Chassis"() -> (w1612:i32)
                            n721 = Index Array(array=w1615, index (row)=w1619, index (col)=w1605) -> (element=w1613:i32)
                            n722 = Multiply(x=w1613, y=w1612) -> (x*y=w1610:i32)
                            n723 = Multiply(x=0.2, y=w1610) -> (x*y=w1609:dbl)
                            n724 = Multiply(x=w1610, y=w1611) -> (x*y=w1607:dbl)
                            n725 = Multiply(x=w1610, y=w1611) -> (x*y=w1606:dbl)
                            n726 = property on="Current (A/s)" class="DigNum (strict)"(error in=w1617, "Minimum"=w1609, "OutOfRngActMin"=u8 1 ("Response to Value Outside Limits:Minimum"), "Maximum"=w1607, "OutOfRngActMax"=u8 1 ("Response to Value Outside Limits:Maximum"), "Value"=w1606) -> (error out=w1616:errorcluster)  [unwired: 1 in, 1 out]
                          }
                          frame 1 {
                            w1630 = i32[][] [[1, 1, 1], [3, 3, 3], [3, 3, 3], [1, 1, 1], [1, 1, 1], [1, 1, 1], [1, 1, 1], [2, 2, 1], [2, 2, 1], [1, 1, 1], [1, 1, 1], [2, 2, 1], [2, 2, 1], [1, 1, 1], [1, 1, 1], [1, 1, 1]]  # Ch Multiple
                            w1626 = 100000.0
                            # "Instr2"
                            n727 = local read "Mode"() -> (w1634:T8)
                            n728 = local read "Chassis"() -> (w1627:i32)
                            n729 = Index Array(array=w1630, index (row)=w1634, index (col)=w1620) -> (element=w1628:i32)
                            n730 = Multiply(x=w1628, y=w1627) -> (x*y=w1625:i32)
                            n731 = Multiply(x=0.2, y=w1625) -> (x*y=w1624:dbl)
                            n732 = Multiply(x=w1625, y=w1626) -> (x*y=w1622:dbl)
                            n733 = Multiply(x=w1625, y=w1626) -> (x*y=w1621:dbl)
                            n734 = property on="Current (A/s)" class="DigNum (strict)"(error in=w1632, "Minimum"=w1624, "OutOfRngActMin"=u8 1 ("Response to Value Outside Limits:Minimum"), "Maximum"=w1622, "OutOfRngActMax"=u8 1 ("Response to Value Outside Limits:Maximum"), "Value"=w1621) -> (error out=w1631:errorcluster)  [unwired: 1 in, 1 out]
                          }
                          frame 2 {
                            w1645 = i32[][] [[1, 1, 1], [3, 3, 3], [3, 3, 3], [1, 1, 1], [1, 1, 1], [1, 1, 1], [1, 1, 1], [2, 2, 1], [2, 2, 1], [1, 1, 1], [1, 1, 1], [2, 2, 1], [2, 2, 1], [1, 1, 1], [1, 1, 1], [1, 1, 1]]  # Ch Multiple
                            w1641 = 100000.0
                            # "Instr3"
                            n735 = local read "Mode"() -> (w1649:T8)
                            n736 = local read "Chassis"() -> (w1642:i32)
                            n737 = Index Array(array=w1645, index (row)=w1649, index (col)=w1635) -> (element=w1643:i32)
                            n738 = Multiply(x=w1643, y=w1642) -> (x*y=w1640:i32)
                            n739 = Multiply(x=0.2, y=w1640) -> (x*y=w1639:dbl)
                            n740 = Multiply(x=w1640, y=w1641) -> (x*y=w1637:dbl)
                            n741 = Multiply(x=w1640, y=w1641) -> (x*y=w1636:dbl)
                            n742 = property on="Current (A/s)" class="DigNum (strict)"(error in=w1647, "Minimum"=w1639, "OutOfRngActMin"=u8 1 ("Response to Value Outside Limits:Minimum"), "Maximum"=w1637, "OutOfRngActMax"=u8 1 ("Response to Value Outside Limits:Maximum"), "Value"=w1636) -> (error out=w1646:errorcluster)  [unwired: 1 in, 1 out]
                          }
                        }
                      }
                    }
                    frame "PSlewCoerce" {
                      # "All instrument channels have the same base Power Slew values [Min=2, Def=1M, Max=1M] but they depend on how many channels are combined together and how many Chassis are on."
                      # "Power (test) slew limits depend on Mode. Power Slew is used for DC instruments."
                      n743 = for {
                        N: 3 -> [_]
                        shift-right: [w1655] -> w1651
                        shift-left: w1650 -> [w1656]
                        i -> [w1657]
                        n744 = case shown="0, Default" w1657 {
                          selector: w1657 -> [w1659 w1674 w1689]
                          tunnel: w1656 -> [w1670 w1685 w1700]
                          tunnel: [w1669 w1684 w1699] -> w1655
                          frame 0, Default {
                            w1658 = i32[][] [[3, 3, 3], [3, 3, 3], [3, 3, 3], [1, 1, 1], [1, 1, 1], [2, 2, 1], [2, 2, 1], [2, 2, 1], [2, 2, 1], [1, 1, 1], [1, 1, 1], [2, 2, 1], [2, 2, 1], [1, 1, 1], [1, 1, 1], [1, 1, 1]]  # Power Ch Multiple
                            w1665 = 1000000.0
                            # "Instr1"
                            n745 = local read "Mode"() -> (w1672:T8)
                            n746 = local read "Chassis"() -> (w1666:i32)
                            n747 = Index Array(array=w1658, index (row)=w1672, index (col)=w1659) -> (element=w1667:i32)
                            n748 = Multiply(x=w1667, y=w1666) -> (x*y=w1664:i32)
                            n749 = Multiply(x=2.0, y=w1664) -> (x*y=w1663:dbl)
                            n750 = Multiply(x=w1664, y=w1665) -> (x*y=w1661:dbl)
                            n751 = Multiply(x=w1664, y=w1665) -> (x*y=w1660:dbl)
                            n752 = property on="Power (W/s)" class="DigNum (strict)"(error in=w1670, "Minimum"=w1663, "OutOfRngActMin"=u8 1 ("Response to Value Outside Limits:Minimum"), "Maximum"=w1661, "OutOfRngActMax"=u8 1 ("Response to Value Outside Limits:Maximum"), "Value"=w1660) -> (error out=w1669:errorcluster)  [unwired: 1 in, 1 out]
                          }
                          frame 1 {
                            w1673 = i32[][] [[3, 3, 3], [3, 3, 3], [3, 3, 3], [1, 1, 1], [1, 1, 1], [2, 2, 1], [2, 2, 1], [2, 2, 1], [2, 2, 1], [1, 1, 1], [1, 1, 1], [2, 2, 1], [2, 2, 1], [1, 1, 1], [1, 1, 1], [1, 1, 1]]  # Power Ch Multiple
                            w1680 = 1000000.0
                            # "Instr2"
                            n753 = local read "Mode"() -> (w1687:T8)
                            n754 = local read "Chassis"() -> (w1681:i32)
                            n755 = Index Array(array=w1673, index (row)=w1687, index (col)=w1674) -> (element=w1682:i32)
                            n756 = Multiply(x=w1682, y=w1681) -> (x*y=w1679:i32)
                            n757 = Multiply(x=2.0, y=w1679) -> (x*y=w1678:dbl)
                            n758 = Multiply(x=w1679, y=w1680) -> (x*y=w1676:dbl)
                            n759 = Multiply(x=w1679, y=w1680) -> (x*y=w1675:dbl)
                            n760 = property on="Power (W/s)" class="DigNum (strict)"(error in=w1685, "Minimum"=w1678, "OutOfRngActMin"=u8 1 ("Response to Value Outside Limits:Minimum"), "Maximum"=w1676, "OutOfRngActMax"=u8 1 ("Response to Value Outside Limits:Maximum"), "Value"=w1675) -> (error out=w1684:errorcluster)  [unwired: 1 in, 1 out]
                          }
                          frame 2 {
                            w1688 = i32[][] [[3, 3, 3], [3, 3, 3], [3, 3, 3], [1, 1, 1], [1, 1, 1], [2, 2, 1], [2, 2, 1], [2, 2, 1], [2, 2, 1], [1, 1, 1], [1, 1, 1], [2, 2, 1], [2, 2, 1], [1, 1, 1], [1, 1, 1], [1, 1, 1]]  # Power Ch Multiple
                            w1695 = 1000000.0
                            # "Instr3"
                            n761 = local read "Mode"() -> (w1702:T8)
                            n762 = local read "Chassis"() -> (w1696:i32)
                            n763 = Index Array(array=w1688, index (row)=w1702, index (col)=w1689) -> (element=w1697:i32)
                            n764 = Multiply(x=w1697, y=w1696) -> (x*y=w1694:i32)
                            n765 = Multiply(x=2.0, y=w1694) -> (x*y=w1693:dbl)
                            n766 = Multiply(x=w1694, y=w1695) -> (x*y=w1691:dbl)
                            n767 = Multiply(x=w1694, y=w1695) -> (x*y=w1690:dbl)
                            n768 = property on="Power (W/s)" class="DigNum (strict)"(error in=w1700, "Minimum"=w1693, "OutOfRngActMin"=u8 1 ("Response to Value Outside Limits:Minimum"), "Maximum"=w1691, "OutOfRngActMax"=u8 1 ("Response to Value Outside Limits:Maximum"), "Value"=w1690) -> (error out=w1699:errorcluster)  [unwired: 1 in, 1 out]
                          }
                        }
                      }
                    }
                    frame "F&PhCoerce" {
                      # "Frequency slew limits and Phase Angle slew limits don't depend on Mode and always have the same values. They are needed for AC instruments."
                      n769 = for {
                        N: 3 -> [_]
                        shift-right: [w1708] -> w1704
                        shift-left: w1703 -> [w1709]
                        i -> [w1710]
                        n770 = case shown="0, Default" w1710 {
                          tunnel: w1709 -> [w1717 w1727 w1737]
                          tunnel: [w1720 w1730 w1740] -> w1708
                          frame 0, Default {
                            w1713 = 50000.0 ("Response to Value Outside Limits:Maximum")
                            w1714 = 500.0 ("Response to Value Outside Limits:Maximum")
                            w1715 = u8 1 ("Response to Value Outside Limits:Maximum")
                            w1716 = u8 1 ("Response to Value Outside Limits:Maximum")
                            # "Instr1"
                            n771 = property on="Frequency (Hz/s)" class="DigNum (strict)"(error in=w1717, "Minimum"=0.01 ("Response to Value Outside Limits:Maximum"), "OutOfRngActMin"=w1716, "OutOfRngActMax"=w1716, "Value"=w1714, "Maximum"=w1714) -> (error out=w1719:errorcluster)  [unwired: 1 in, 1 out]
                            n772 = property on="Phase Angle (Deg/s)" class="DigNum (strict)"(error in=w1717, "Minimum"=0.1 ("Response to Value Outside Limits:Maximum"), "OutOfRngActMin"=w1715, "OutOfRngActMax"=w1715, "Value"=w1713, "Maximum"=w1713) -> (error out=w1718:errorcluster)  [unwired: 1 in, 1 out]
                            n773 = Merge Errors(w1719, w1718) -> (w1720:errorcluster)
                          }
                          frame 1 {
                            w1722 = 50000.0 ("Response to Value Outside Limits:Maximum")
                            w1724 = 500.0 ("Response to Value Outside Limits:Maximum")
                            w1725 = u8 1 ("Response to Value Outside Limits:Maximum")
                            w1726 = u8 1 ("Response to Value Outside Limits:Maximum")
                            # "Instr2"
                            n774 = property on="Frequency (Hz/s)" class="DigNum (strict)"(error in=w1727, "Minimum"=0.01 ("Response to Value Outside Limits:Maximum"), "OutOfRngActMin"=w1726, "OutOfRngActMax"=w1726, "Value"=w1724, "Maximum"=w1724) -> (error out=w1729:errorcluster)  [unwired: 1 in, 1 out]
                            n775 = property on="Phase Angle (Deg/s)" class="DigNum (strict)"(error in=w1727, "Minimum"=0.1 ("Response to Value Outside Limits:Maximum"), "OutOfRngActMin"=w1725, "OutOfRngActMax"=w1725, "Value"=w1722, "Maximum"=w1722) -> (error out=w1728:errorcluster)  [unwired: 1 in, 1 out]
                            n776 = Merge Errors(w1729, w1728) -> (w1730:errorcluster)
                          }
                          frame 2 {
                            w1732 = 50000.0 ("Response to Value Outside Limits:Maximum")
                            w1734 = 500.0 ("Response to Value Outside Limits:Maximum")
                            w1735 = u8 1 ("Response to Value Outside Limits:Maximum")
                            w1736 = u8 1 ("Response to Value Outside Limits:Maximum")
                            # "Instr3"
                            n777 = property on="Frequency (Hz/s)" class="DigNum (strict)"(error in=w1737, "Minimum"=0.01 ("Response to Value Outside Limits:Maximum"), "OutOfRngActMin"=w1736, "OutOfRngActMax"=w1736, "Value"=w1734, "Maximum"=w1734) -> (error out=w1739:errorcluster)  [unwired: 1 in, 1 out]
                            n778 = property on="Phase Angle (Deg/s)" class="DigNum (strict)"(error in=w1737, "Minimum"=0.1 ("Response to Value Outside Limits:Maximum"), "OutOfRngActMin"=w1735, "OutOfRngActMax"=w1735, "Value"=w1732, "Maximum"=w1732) -> (error out=w1738:errorcluster)  [unwired: 1 in, 1 out]
                            n779 = Merge Errors(w1739, w1738) -> (w1740:errorcluster)
                          }
                        }
                      }
                    }
                    frame "SlewsCurr" {
                      # "Store the same status given to the Current slew controls in Device(s)Settings for later retrieval. Current slews are column index 14 in the array."
                      # "Slew types have specific avilability depending if the instrument is AC or DC. In the case of the Current Slew, it is avilable for DC only."
                      n780 = for {
                        N: 3 -> [_]
                        shift-right: [w1755] -> w1743
                        shift-left: w1742 -> [w1756]
                        shift-right: [w1754] -> w1741
                        shift-left: u8[] [] -> [w1759]
                        i -> [w1758]
                        w1753 = i8[][] [[2, 2, 2], [2, 2, 2], [0, 0, 0], [2, 2, 2], [0, 0, 0], [2, 2, 2], [2, 2, 0], [2, 2, 2], [2, 2, 0], [2, 2, 0], [2, 0, 0], [0, 0, 2], [0, 0, 0], [2, 0, 2], [0, 2, 2], [0, 2, 0]]  # Curr/Pow Slew Enable
                        n781 = local read "Mode"() -> (w1760:T8)
                        n782 = Index Array(array=w1753, index (row)=w1760, index (col)=w1758) -> (element=w1757:i8)
                        n783 = Build Array (concatenate)(w1759, w1757) -> (w1754:u8[])
                        n784 = case shown="2" w1758 {
                          tunnel: w1757 -> [w1763 w1766 w1769]
                          tunnel: w1756 -> [w1762 w1765 w1768]
                          tunnel: [w1761 w1764 w1767] -> w1755
                          frame 0, Default {
                            # "Instr1"
                            n785 = property on="Current (A/s)" class="DigNum (strict)"(error in=w1762, "DisabledEnum"=w1763) -> (error out=w1761:errorcluster)  [unwired: 1 in, 1 out]
                          }
                          frame 1 {
                            # "Instr2"
                            n786 = property on="Current (A/s)" class="DigNum (strict)"(error in=w1765, "DisabledEnum"=w1766) -> (error out=w1764:errorcluster)  [unwired: 1 in, 1 out]
                          }
                          frame 2 {
                            # "Instr3"
                            n787 = property on="Current (A/s)" class="DigNum (strict)"(error in=w1768, "DisabledEnum"=w1769) -> (error out=w1767:errorcluster)  [unwired: 1 in, 1 out]
                          }
                        }
                      }
                      n788 = property on="EnableCtrls" class="Arr (strict)"(error in=w1743) -> (error out=w1750:errorcluster, "Value"=w1749:i8[][])  [unwired: 1 in, 1 out]
                      n789 = Replace Array Subset(array=w1749, new element=w1741, index (col)=14 ("disabled index (col)")) -> (w1748:i8[][])  [unwired: 1 in]
                      n790 = property on="EnableCtrls" class="Arr (strict)"(error in=w1750, "Value"=w1748) -> (error out=w1746:errorcluster)  [unwired: 1 in, 1 out]
                    }
                    frame "SlewsPow" {
                      # "Store the same status given to the Power slew controls in Device(s)Settings for later retrieval. Power slews are column index 15 in the array."
                      # "Slew types have specific avilability depending if the instrument is AC or DC. In the case of Power Slew, it is avilable for DC only."
                      n791 = for {
                        N: 3 -> [_]
                        shift-right: [w1784] -> w1772
                        shift-left: w1771 -> [w1785]
                        shift-right: [w1783] -> w1770
                        shift-left: u8[] [] -> [w1788]
                        i -> [w1787]
                        w1782 = i8[][] [[2, 2, 2], [2, 2, 2], [0, 0, 0], [2, 2, 2], [0, 0, 0], [2, 2, 2], [2, 2, 0], [2, 2, 2], [2, 2, 0], [2, 2, 0], [2, 0, 0], [0, 0, 2], [0, 0, 0], [2, 0, 2], [0, 2, 2], [0, 2, 0]]  # Curr/Pow Slew Enable
                        n792 = local read "Mode"() -> (w1789:T8)
                        n793 = Index Array(array=w1782, index (row)=w1789, index (col)=w1787) -> (element=w1786:i8)
                        n794 = Build Array (concatenate)(w1788, w1786) -> (w1783:u8[])
                        n795 = case shown="0, Default" w1787 {
                          tunnel: w1786 -> [w1792 w1795 w1798]
                          tunnel: w1785 -> [w1791 w1794 w1797]
                          tunnel: [w1790 w1793 w1796] -> w1784
                          frame 0, Default {
                            # "Instr1"
                            n796 = property on="Power (W/s)" class="DigNum (strict)"(error in=w1791, "DisabledEnum"=w1792) -> (error out=w1790:errorcluster)  [unwired: 1 in, 1 out]
                          }
                          frame 1 {
                            # "Instr2"
                            n797 = property on="Power (W/s)" class="DigNum (strict)"(error in=w1794, "DisabledEnum"=w1795) -> (error out=w1793:errorcluster)  [unwired: 1 in, 1 out]
                          }
                          frame 2 {
                            # "Instr3"
                            n798 = property on="Power (W/s)" class="DigNum (strict)"(error in=w1797, "DisabledEnum"=w1798) -> (error out=w1796:errorcluster)  [unwired: 1 in, 1 out]
                          }
                        }
                      }
                      n799 = property on="EnableCtrls" class="Arr (strict)"(error in=w1772) -> (error out=w1779:errorcluster, "Value"=w1778:i8[][])  [unwired: 1 in, 1 out]
                      n800 = Replace Array Subset(array=w1778, new element=w1770, index (col)=15 ("disabled index (col)")) -> (w1777:i8[][])  [unwired: 1 in]
                      n801 = property on="EnableCtrls" class="Arr (strict)"(error in=w1779, "Value"=w1777) -> (error out=w1775:errorcluster)  [unwired: 1 in, 1 out]
                    }
                    frame "SlewsFreq" {
                      # "Store the same status given to the Frequency slew controls in Device(s)Settings for later retrieval. Frequency slews are column index 16 in the array."
                      # "Slew types have specific avilability depending if the instrument is AC or DC. In the case of Frequency Slew, it is avilable for AC only."
                      n802 = for {
                        N: 3 -> [_]
                        shift-right: [w1813] -> w1800
                        shift-left: w1801 -> [w1814]
                        shift-right: [w1812] -> w1799
                        shift-left: u8[] [] -> [w1817]
                        i -> [w1816]
                        w1811 = i8[][] [[0, 0, 0], [0, 0, 0], [2, 2, 2], [0, 0, 0], [2, 2, 2], [0, 0, 0], [0, 0, 2], [0, 0, 0], [0, 0, 2], [0, 0, 2], [0, 2, 2], [2, 2, 0], [2, 2, 2], [0, 2, 0], [2, 0, 0], [2, 0, 2]]  # Freq/Phas Slew Enable
                        n803 = local read "Mode"() -> (w1818:T8)
                        n804 = Index Array(array=w1811, index (row)=w1818, index (col)=w1816) -> (element=w1815:i8)
                        n805 = Build Array (concatenate)(w1817, w1815) -> (w1812:u8[])
                        n806 = case shown="0, Default" w1816 {
                          tunnel: w1815 -> [w1821 w1824 w1827]
                          tunnel: w1814 -> [w1820 w1823 w1826]
                          tunnel: [w1819 w1822 w1825] -> w1813
                          frame 0, Default {
                            # "Instr1"
                            n807 = property on="Frequency (Hz/s)" class="DigNum (strict)"(error in=w1820, "DisabledEnum"=w1821) -> (error out=w1819:errorcluster)  [unwired: 1 in, 1 out]
                          }
                          frame 1 {
                            # "Instr2"
                            n808 = property on="Frequency (Hz/s)" class="DigNum (strict)"(error in=w1823, "DisabledEnum"=w1824) -> (error out=w1822:errorcluster)  [unwired: 1 in, 1 out]
                          }
                          frame 2 {
                            # "Instr3"
                            n809 = property on="Frequency (Hz/s)" class="DigNum (strict)"(error in=w1826, "DisabledEnum"=w1827) -> (error out=w1825:errorcluster)  [unwired: 1 in, 1 out]
                          }
                        }
                      }
                      n810 = property on="EnableCtrls" class="Arr (strict)"(error in=w1800) -> (error out=w1808:errorcluster, "Value"=w1807:i8[][])  [unwired: 1 in, 1 out]
                      n811 = Replace Array Subset(array=w1807, new element=w1799, index (col)=16 ("disabled index (col)")) -> (w1806:i8[][])  [unwired: 1 in]
                      n812 = property on="EnableCtrls" class="Arr (strict)"(error in=w1808, "Value"=w1806) -> (error out=w1804:errorcluster)  [unwired: 1 in, 1 out]
                    }
                    frame "SlewsPhase" {
                      # "Store the same status given to the Phase Angle slew controls in Device(s)Settings for later retrieval. Phase Angle slews are column index 17 in the array."
                      # "Slew types have specific avilability depending if the instrument is AC or DC. In the case of the Phase Angle slew, it is avilable for AC only."
                      n813 = for {
                        N: 3 -> [_]
                        shift-right: [w1842] -> w1830
                        shift-left: w1829 -> [w1843]
                        shift-right: [w1841] -> w1828
                        shift-left: u8[] [] -> [w1846]
                        i -> [w1845]
                        w1840 = i8[][] [[0, 0, 0], [0, 0, 0], [2, 2, 2], [0, 0, 0], [2, 2, 2], [0, 0, 0], [0, 0, 2], [0, 0, 0], [0, 0, 2], [0, 0, 2], [0, 2, 2], [2, 2, 0], [2, 2, 2], [0, 2, 0], [2, 0, 0], [2, 0, 2]]  # Freq/Phas Slew Enable
                        n814 = local read "Mode"() -> (w1847:T8)
                        n815 = Index Array(array=w1840, index (row)=w1847, index (col)=w1845) -> (element=w1844:i8)
                        n816 = Build Array (concatenate)(w1846, w1844) -> (w1841:u8[])
                        n817 = case shown="0, Default" w1845 {
                          tunnel: w1844 -> [w1850 w1853 w1856]
                          tunnel: w1843 -> [w1849 w1852 w1855]
                          tunnel: [w1848 w1851 w1854] -> w1842
                          frame 0, Default {
                            # "Instr1"
                            n818 = property on="Phase Angle (Deg/s)" class="DigNum (strict)"(error in=w1849, "DisabledEnum"=w1850) -> (error out=w1848:errorcluster)  [unwired: 1 in, 1 out]
                          }
                          frame 1 {
                            # "Instr2"
                            n819 = property on="Phase Angle (Deg/s)" class="DigNum (strict)"(error in=w1852, "DisabledEnum"=w1853) -> (error out=w1851:errorcluster)  [unwired: 1 in, 1 out]
                          }
                          frame 2 {
                            # "Instr3"
                            n820 = property on="Phase Angle (Deg/s)" class="DigNum (strict)"(error in=w1855, "DisabledEnum"=w1856) -> (error out=w1854:errorcluster)  [unwired: 1 in, 1 out]
                          }
                        }
                      }
                      n821 = property on="EnableCtrls" class="Arr (strict)"(error in=w1830) -> (error out=w1837:errorcluster, "Value"=w1836:i8[][])  [unwired: 1 in, 1 out]
                      n822 = Replace Array Subset(array=w1836, new element=w1828, index (col)=17 ("disabled index (col)")) -> (w1835:i8[][])  [unwired: 1 in]
                      n823 = property on="EnableCtrls" class="Arr (strict)"(error in=w1837, "Value"=w1835) -> (error out=w1833:errorcluster)  [unwired: 1 in, 1 out]
                    }
                    frame "TripTCoerce1" {
                      w1857 = -1.0 ("Response to Value Outside Limits:Maximum")
                      w1863 = u8 1 ("Response to Value Outside Limits:Maximum")
                      w1865 = u8 1 ("Response to Value Outside Limits:Maximum")
                      w1864 = u8 1 ("Response to Value Outside Limits:Maximum")
                      w1858 = 3600.0 ("Response to Value Outside Limits:Maximum")
                      w1859 = -1.0 ("Response to Value Outside Limits:Maximum")
                      w1860 = u8 1 ("Response to Value Outside Limits:Maximum")
                      w1861 = u8 1 ("Response to Value Outside Limits:Maximum")
                      w1862 = u8 1 ("Response to Value Outside Limits:Maximum")
                      # "These are all for INSTR1 only"
                      # "Time trips for Instr1: trips are treated the same way for all modes and instruments"
                      n824 = property on="I Snk Time (s)" class="DigNum (strict)"(error in=w1870, "Value"=w1859, "Minimum"=w1859, "OutOfRngActMin"=w1862, "OutOfRngActMax"=w1862, "Maximum"=w1858) -> (error out=w1872:errorcluster)  [unwired: 1 in, 1 out]
                      n825 = property on="P Src Time (s)" class="DigNum (strict)"(error in=w1870, "Maximum"=w1858, "OutOfRngActMin"=w1864, "OutOfRngActMax"=w1864, "Value"=w1857, "Minimum"=w1857) -> (error out=w1869:errorcluster)  [unwired: 1 in, 1 out]
                      n826 = property on="I Src Time (s)" class="DigNum (strict)"(error in=w1872, "Value"=w1859, "Minimum"=w1859, "OutOfRngActMin"=w1861, "OutOfRngActMax"=w1861, "Maximum"=w1858) -> (error out=w1871:errorcluster)  [unwired: 1 in, 1 out]
                      n827 = property on="Vmax Time (s)" class="DigNum (strict)"(error in=w1869, "Maximum"=w1858, "OutOfRngActMin"=w1865, "OutOfRngActMax"=w1865, "Value"=w1857, "Minimum"=w1857) -> (error out=w1868:errorcluster)  [unwired: 1 in, 1 out]
                      n828 = property on="P Snk Time (s)" class="DigNum (strict)"(error in=w1871, "Value"=w1859, "Minimum"=w1859, "OutOfRngActMin"=w1860, "OutOfRngActMax"=w1860, "Maximum"=w1858) -> (error out=w1866:errorcluster)  [unwired: 1 in, 1 out]
                      n829 = property on="Vmin Time (s)" class="DigNum (strict)"(error in=w1868, "Maximum"=w1858, "OutOfRngActMin"=w1863, "OutOfRngActMax"=w1863, "Value"=w1857, "Minimum"=w1857) -> (error out=w1867:errorcluster)  [unwired: 1 in, 1 out]
                      n830 = Merge Errors(w1866, w1867) -> (w1873:errorcluster)
                    }
                    frame "TripTCoerce2" {
                      w1876 = -1.0 ("Response to Value Outside Limits:Maximum")
                      w1878 = 3600.0 ("Response to Value Outside Limits:Maximum")
                      w1879 = u8 1 ("Response to Value Outside Limits:Maximum")
                      w1880 = u8 1 ("Response to Value Outside Limits:Maximum")
                      w1881 = u8 1 ("Response to Value Outside Limits:Maximum")
                      w1877 = -1.0 ("Response to Value Outside Limits:Maximum")
                      w1882 = u8 1 ("Response to Value Outside Limits:Maximum")
                      w1883 = u8 1 ("Response to Value Outside Limits:Maximum")
                      w1884 = u8 1 ("Response to Value Outside Limits:Maximum")
                      # "These are all for INSTR2 only"
                      # "Time trips for Instr2: trips are treated the same way for all modes and instruments"
                      n831 = property on="I Snk Time (s)" class="DigNum (strict)"(error in=w1889, "Value"=w1877, "Minimum"=w1877, "OutOfRngActMin"=w1884, "OutOfRngActMax"=w1884, "Maximum"=w1878) -> (error out=w1891:errorcluster)  [unwired: 1 in, 1 out]
                      n832 = property on="P Src Time (s)" class="DigNum (strict)"(error in=w1889, "Maximum"=w1878, "OutOfRngActMin"=w1881, "OutOfRngActMax"=w1881, "Value"=w1876, "Minimum"=w1876) -> (error out=w1888:errorcluster)  [unwired: 1 in, 1 out]
                      n833 = property on="I Src Time (s)" class="DigNum (strict)"(error in=w1891, "Value"=w1877, "Minimum"=w1877, "OutOfRngActMin"=w1883, "OutOfRngActMax"=w1883, "Maximum"=w1878) -> (error out=w1890:errorcluster)  [unwired: 1 in, 1 out]
                      n834 = property on="Vmax Time (s)" class="DigNum (strict)"(error in=w1888, "Maximum"=w1878, "OutOfRngActMin"=w1880, "OutOfRngActMax"=w1880, "Value"=w1876, "Minimum"=w1876) -> (error out=w1887:errorcluster)  [unwired: 1 in, 1 out]
                      n835 = property on="P Snk Time (s)" class="DigNum (strict)"(error in=w1890, "Value"=w1877, "Minimum"=w1877, "OutOfRngActMin"=w1882, "OutOfRngActMax"=w1882, "Maximum"=w1878) -> (error out=w1885:errorcluster)  [unwired: 1 in, 1 out]
                      n836 = property on="Vmin Time (s)" class="DigNum (strict)"(error in=w1887, "Maximum"=w1878, "OutOfRngActMin"=w1879, "OutOfRngActMax"=w1879, "Value"=w1876, "Minimum"=w1876) -> (error out=w1886:errorcluster)  [unwired: 1 in, 1 out]
                      n837 = Merge Errors(w1885, w1886) -> (w1892:errorcluster)
                    }
                    frame "TripTCoerce3" {
                      w1895 = -1.0 ("Response to Value Outside Limits:Maximum")
                      w1897 = 3600.0 ("Response to Value Outside Limits:Maximum")
                      w1910 = u8 1 ("Response to Value Outside Limits:Maximum")
                      w1909 = u8 1 ("Response to Value Outside Limits:Maximum")
                      w1908 = u8 1 ("Response to Value Outside Limits:Maximum")
                      w1896 = -1.0 ("Response to Value Outside Limits:Maximum")
                      w1905 = u8 1 ("Response to Value Outside Limits:Maximum")
                      w1906 = u8 1 ("Response to Value Outside Limits:Maximum")
                      w1907 = u8 1 ("Response to Value Outside Limits:Maximum")
                      # "These are all for INSTR3 only"
                      # "Time trips for Instr3: trips are treated the same way for all modes and instruments"
                      n838 = property on="I Snk Time (s)" class="DigNum (strict)"(error in=w1900, "Value"=w1896, "Minimum"=w1896, "OutOfRngActMin"=w1907, "OutOfRngActMax"=w1907, "Maximum"=w1897) -> (error out=w1904:errorcluster)  [unwired: 1 in, 1 out]
                      n839 = property on="P Src Time (s)" class="DigNum (strict)"(error in=w1900, "Maximum"=w1897, "OutOfRngActMin"=w1908, "OutOfRngActMax"=w1908, "Value"=w1895, "Minimum"=w1895) -> (error out=w1899:errorcluster)  [unwired: 1 in, 1 out]
                      n840 = property on="I Src Time (s)" class="DigNum (strict)"(error in=w1904, "Value"=w1896, "Minimum"=w1896, "OutOfRngActMin"=w1906, "OutOfRngActMax"=w1906, "Maximum"=w1897) -> (error out=w1903:errorcluster)  [unwired: 1 in, 1 out]
                      n841 = property on="Vmax Time (s)" class="DigNum (strict)"(error in=w1899, "Maximum"=w1897, "OutOfRngActMin"=w1909, "OutOfRngActMax"=w1909, "Value"=w1895, "Minimum"=w1895) -> (error out=w1898:errorcluster)  [unwired: 1 in, 1 out]
                      n842 = property on="P Snk Time (s)" class="DigNum (strict)"(error in=w1903, "Value"=w1896, "Minimum"=w1896, "OutOfRngActMin"=w1905, "OutOfRngActMax"=w1905, "Maximum"=w1897) -> (error out=w1902:errorcluster)  [unwired: 1 in, 1 out]
                      n843 = property on="Vmin Time (s)" class="DigNum (strict)"(error in=w1898, "Maximum"=w1897, "OutOfRngActMin"=w1910, "OutOfRngActMax"=w1910, "Value"=w1895, "Minimum"=w1895) -> (error out=w1901:errorcluster)  [unwired: 1 in, 1 out]
                      n844 = Merge Errors(w1902, w1901) -> (w1911:errorcluster)
                    }
                    frame "VPhaseCoerce" {
                      # "INSTR1 is the only one that can have pahse voltages, and they are not allowed to be more than 350 V individually."
                      n845 = local read "Mode"() -> (w1915:T8)
                      n846 = case shown="0" w1915 {
                        tunnel: w1917 -> [w1924 w1933 w1936]
                        tunnel: [w1921 w1931 w1936] -> w1916
                        frame 0 {
                          w1920 = u8 1 ("Response to Value Outside Limits:Maximum")
                          # "1= Coerce"
                          # "Will give 349.87 max per phase, not exactly 350. Otherwise, they would exceed the 606V maximum when combined."
                          # "For Thee-Phase the value cannot be exactly 350 or it will yield more than Vout=606 V"
                          n847 = Square Root(x=3.0) -> (sqrt(x)=w1926:dbl)
                          n848 = Divide(x=606.0 ("Response to Value Outside Limits:Maximum"), y=w1926) -> (x/y=w1919:dbl)
                          n849 = property on="A-Volts (V)" class="DigNum (strict)"(error in=w1924, "Maximum"=w1919, "OutOfRngActMax"=w1920) -> (error out=w1923:errorcluster)  [unwired: 1 in, 1 out]
                          n850 = property on="B-Volts (V)" class="DigNum (strict)"(error in=w1923, "Maximum"=w1919, "OutOfRngActMax"=w1920) -> (error out=w1922:errorcluster)  [unwired: 1 in, 1 out]
                          n851 = property on="C-Volts (V)" class="DigNum (strict)"(error in=w1922, "Maximum"=w1919, "OutOfRngActMax"=w1920) -> (error out=w1921:errorcluster)  [unwired: 1 in, 1 out]
                        }
                        frame 5, 6 {
                          w1934 = 350.0 ("Response to Value Outside Limits:Maximum")
                          w1932 = u8 1 ("Response to Value Outside Limits:Maximum")
                          # "Also, the sum of both phases for the Two-Phase mode cannot exceed the total 500 V maximum. This is managed in the other code sections dedicated to control Vout and the phase voltages."
                          # "Instr3 will be 1-Phase\\Channel. Not affected."
                          # "The Two-Phase Modes can have the exact maximum value of 350 on each phase"
                          n852 = property on="A-Volts (V)" class="DigNum (strict)"(error in=w1933, "Maximum"=w1934, "OutOfRngActMax"=w1932) -> (error out=w1935:errorcluster)  [unwired: 1 in, 1 out]
                          n853 = property on="B-Volts (V)" class="DigNum (strict)"(error in=w1935, "Maximum"=w1934, "OutOfRngActMax"=w1932) -> (error out=w1931:errorcluster)  [unwired: 1 in, 1 out]
                          n854 = local read "Instr3"() -> (w1929:T2)
                          n855 = Bundle By Name(cluster=w1929, "Vout (V)"=0.0) -> (w1930:T2)
                          n856 = local write "Instr3"(w1930) -> ()
                        }
                        frame Default {
                          # "This does not apply for the other Modes that are not multi-phase."
                        }
                      }
                    }
                    frame "WaveLists" {
                      w1948 = 0 ("Value")
                      w1947 = 0 ("Value")
                      w1946 = 0 ("Value")
                      w1937 = string[] ["Sine", "User1", "User2", "User3"] ("Strings []")
                      # "If the user wants different waveforms than the default Sine, Triangular, etc. provided by the unit, they have to be loaded separately by following the procedure explained in the device manual, and then saved in the configuration to be recalled later."
                      # "Instr3"
                      # "Instr2"
                      # "Instr1"
                      # "0= First index = Sine"
                      # "By default the waveform shape will be set always to Sine"
                      # "Save the default AC Wave Shape control list of options for each instrument"
                      n857 = property on="A-Wave Shape" class="Ring (strict)"(error in=w1957, "Strings []"=w1937) -> (error out=w1956:errorcluster)  [unwired: 1 in, 1 out]
                      n858 = property on="B-Wave Shape" class="Ring (strict)"(error in=w1956, "Strings []"=w1937) -> (error out=w1945:errorcluster)  [unwired: 1 in, 1 out]
                      n859 = property on="C-Wave Shape" class="Ring (strict)"(error in=w1945, "Strings []"=w1937) -> (error out=w1940:errorcluster)  [unwired: 1 in, 1 out]
                      n860 = local read "Instr1"() -> (w1953:T2)
                      n861 = Bundle By Name(cluster=w1953, "Phases.A-Wave Shape"=w1946, "Phases.B-Wave Shape"=w1946, "Phases.C-Wave Shape"=w1946) -> (w1954:T2)
                      n862 = local write "Instr1"(w1954) -> ()
                      n863 = property on="A-Wave Shape" class="Ring (strict)"(error in=w1940, "Strings []"=w1937) -> (error out=w1943:errorcluster)  [unwired: 1 in, 1 out]
                      n864 = property on="B-Wave Shape" class="Ring (strict)"(error in=w1943, "Strings []"=w1937) -> (error out=w1944:errorcluster)  [unwired: 1 in, 1 out]
                      n865 = local read "Instr2"() -> (w1952:T2)
                      n866 = Bundle By Name(cluster=w1952, "Phases.A-Wave Shape"=w1947, "Phases.B-Wave Shape"=w1947, "Phases.C-Wave Shape"=w1947) -> (w1951:T2)
                      n867 = property on="C-Wave Shape" class="Ring (strict)"(error in=w1944, "Strings []"=w1937) -> (error out=w1939:errorcluster)  [unwired: 1 in, 1 out]
                      n868 = local write "Instr2"(w1951) -> ()
                      n869 = property on="A-Wave Shape" class="Ring (strict)"(error in=w1939, "Strings []"=w1937) -> (error out=w1942:errorcluster)  [unwired: 1 in, 1 out]
                      n870 = local read "Instr3"() -> (w1949:T2)
                      n871 = Bundle By Name(cluster=w1949, "Phases.A-Wave Shape"=w1948, "Phases.B-Wave Shape"=w1948, "Phases.C-Wave Shape"=w1948) -> (w1950:T2)
                      n872 = property on="B-Wave Shape" class="Ring (strict)"(error in=w1942, "Strings []"=w1937) -> (error out=w1941:errorcluster)  [unwired: 1 in, 1 out]
                      n873 = property on="C-Wave Shape" class="Ring (strict)"(error in=w1941, "Strings []"=w1937) -> (error out=w1938:errorcluster)  [unwired: 1 in, 1 out]
                      n874 = local write "Instr3"(w1950) -> ()
                    }
                    frame "WaveEnable" {
                      w1966 = i8[][] [[0, 0, 0], [0, 2, 2], [0, 0, 0], [0, 2, 2], [2, 2, 2], [0, 2, 2], [2, 2, 2], [0, 2, 2], [2, 2, 2], [2, 2, 2], [2, 2, 2], [0, 2, 2], [2, 2, 2], [0, 2, 2], [0, 2, 2], [2, 2, 2]]  # Wave Enable 3
                      w1965 = i8[][] [[0, 0, 0], [0, 2, 2], [0, 0, 0], [0, 2, 2], [2, 2, 2], [0, 0, 2], [0, 0, 2], [0, 2, 2], [0, 2, 2], [0, 2, 2], [2, 2, 2], [2, 2, 2], [2, 2, 2], [2, 2, 2], [0, 2, 2], [0, 2, 2]]  # Wave Enable 2
                      w1964 = i8[][] [[0, 0, 0], [0, 2, 2], [0, 0, 0], [0, 2, 2], [2, 2, 2], [0, 0, 2], [0, 0, 2], [0, 2, 2], [0, 2, 2], [0, 2, 2], [0, 2, 2], [2, 2, 2], [2, 2, 2], [0, 2, 2], [2, 2, 2], [2, 2, 2]]  # Wave Enable 1
                      # "Store the same status given to the Wave Shape controls in Device(s)Settings for later retrieval. Wave Shapes are column indexes 11, 12 & 13 in the array."
                      # "Only AC instruments should have AC waveform selection enabled."
                      n875 = local read "Mode"() -> (w1971:T8)
                      n876 = for {
                        N: 3 -> [_]
                        shift-right: [w1990] -> w1962
                        shift-left: w1963 -> [w1991]
                        shift-right: [w1989] -> w1961
                        shift-left: u8[] [] -> [w1996]
                        shift-right: [w1988] -> w1960
                        shift-left: u8[] [] -> [w1997]
                        shift-right: [w1987] -> w1959
                        shift-left: u8[] [] -> [w1998]
                        tunnel: w1966 -> [w1986]
                        tunnel: w1965 -> [w1985]
                        tunnel: w1964 -> [w1984]
                        tunnel: w1971 -> [w1983]
                        i -> [w1995]
                        n877 = Index Array(array=w1984, index (row)=w1983, index (col)=w1995) -> (element=w1994:i8)
                        n878 = Index Array(array=w1985, index (row)=w1983, index (col)=w1995) -> (element=w1993:i8)
                        n879 = Index Array(array=w1986, index (row)=w1983, index (col)=w1995) -> (element=w1992:i8)
                        n880 = Build Array (concatenate)(w1998, w1992) -> (w1987:u8[])
                        n881 = Build Array (concatenate)(w1997, w1993) -> (w1988:u8[])
                        n882 = Build Array (concatenate)(w1996, w1994) -> (w1989:u8[])
                        n883 = case shown="0, Default" w1995 {
                          tunnel: w1994 -> [w2006 w2014 w2022]
                          tunnel: w1993 -> [w2005 w2013 w2021]
                          tunnel: w1992 -> [w2004 w2012 w2020]
                          tunnel: w1991 -> [w2000 w2008 w2016]
                          tunnel: [w1999 w2007 w2015] -> w1990
                          frame 0, Default {
                            # "Instr1"
                            n884 = property on="C-Wave Shape" class="Ring (strict)"(error in=w2000, "DisabledEnum"=w2004) -> (error out=w2001:errorcluster)  [unwired: 1 in, 1 out]
                            n885 = property on="A-Wave Shape" class="Ring (strict)"(error in=w2000, "DisabledEnum"=w2006) -> (error out=w2003:errorcluster)  [unwired: 1 in, 1 out]
                            n886 = property on="B-Wave Shape" class="Ring (strict)"(error in=w2000, "DisabledEnum"=w2005) -> (error out=w2002:errorcluster)  [unwired: 1 in, 1 out]
                            n887 = Merge Errors(w2003, w2002, w2001) -> (w1999:errorcluster)
                          }
                          frame 1 {
                            # "Instr2"
                            n888 = property on="C-Wave Shape" class="Ring (strict)"(error in=w2008, "DisabledEnum"=w2012) -> (error out=w2009:errorcluster)  [unwired: 1 in, 1 out]
                            n889 = property on="A-Wave Shape" class="Ring (strict)"(error in=w2008, "DisabledEnum"=w2014) -> (error out=w2011:errorcluster)  [unwired: 1 in, 1 out]
                            n890 = property on="B-Wave Shape" class="Ring (strict)"(error in=w2008, "DisabledEnum"=w2013) -> (error out=w2010:errorcluster)  [unwired: 1 in, 1 out]
                            n891 = Merge Errors(w2011, w2010, w2009) -> (w2007:errorcluster)
                          }
                          frame 2 {
                            # "Instr3"
                            n892 = property on="C-Wave Shape" class="Ring (strict)"(error in=w2016, "DisabledEnum"=w2020) -> (error out=w2017:errorcluster)  [unwired: 1 in, 1 out]
                            n893 = property on="A-Wave Shape" class="Ring (strict)"(error in=w2016, "DisabledEnum"=w2022) -> (error out=w2019:errorcluster)  [unwired: 1 in, 1 out]
                            n894 = property on="B-Wave Shape" class="Ring (strict)"(error in=w2016, "DisabledEnum"=w2021) -> (error out=w2018:errorcluster)  [unwired: 1 in, 1 out]
                            n895 = Merge Errors(w2019, w2018, w2017) -> (w2015:errorcluster)
                          }
                        }
                      }
                      n896 = property on="EnableCtrls" class="Arr (strict)"(error in=w1962) -> (error out=w1973:errorcluster, "Value"=w1977:i8[][])  [unwired: 1 in, 1 out]
                      n897 = Replace Array Subset(array=w1977, new element=w1961, index (col)=11 ("disabled index (col)")) -> (w1978:i8[][])  [unwired: 1 in]
                      n898 = Replace Array Subset(array=w1978, new element=w1960, index (col)=12 ("disabled index (col)")) -> (w1979:i8[][])  [unwired: 1 in]
                      n899 = Replace Array Subset(array=w1979, new element=w1959, index (col)=13 ("disabled index (col)")) -> (w1980:i8[][])  [unwired: 1 in]
                      n900 = property on="EnableCtrls" class="Arr (strict)"(error in=w1973, "Value"=w1980) -> (error out=w1972:errorcluster)  [unwired: 1 in, 1 out]
                    }
                  }
                }
                frame Error {
                  # "In case of error, this will pass over the state machine. Helpful while debugging to avoid so many cases."
                }
              }
            }
            n901 = property on="Update" class="Bool (strict)"(error in=w824) -> (error out=w825:errorcluster, "Value"=w822:bool)  [unwired: 1 in, 1 out]
            n902 = property on="btnSaveAs" class="Bool"(error in=w824, "DisabledEnum"=w827) -> (error out=w829:errorcluster)  [unwired: 1 in, 1 out]
            n903 = property on="btnSave" class="Bool"(error in=w824, "DisabledEnum"=w827) -> (error out=w828:errorcluster)  [unwired: 1 in, 1 out]
            n904 = property on="Update" class="Bool (strict)"(error in=w825, "Val(Sgnl)"=w822) -> (error out=w823:errorcluster)  [unwired: 1 in, 1 out]
            n905 = Merge Errors(w828, w829, w823) -> (w826:errorcluster)
          }
          event "Chassis": Value Change {
            w2032 = T15."Enabled" ("Disabled")
            w2036 = FALSE ("StartMeas")
            # "Let the \"Mode Change\" event fix all the other settings, specially the Current and Power ones, to reflect the new value of Chassis."
            # "Update Device(s)Settings"
            n906 = event-data() -> ()  [unwired: 1 in, 6 out]
            n907 = property on="Mode" class="Ring (strict)"(error in=w2027) -> (error out=w2030:errorcluster, "Value"=w2029:T8)  [unwired: 1 in, 1 out]
            n908 = property on="Mode" class="Ring (strict)"(error in=w2030, "Val(Sgnl)"=w2029) -> (error out=w2028:errorcluster)  [unwired: 1 in, 1 out]
            n909 = property on="Update" class="Bool (strict)"(error in=w2028) -> (error out=w2035:errorcluster, "Value"=w2026:bool)  [unwired: 1 in, 1 out]
            n910 = property on="Update" class="Bool (strict)"(error in=w2035, "Val(Sgnl)"=w2026) -> (error out=w2031:errorcluster)  [unwired: 1 in, 1 out]
            n911 = property on="btnSaveAs" class="Bool"(error in=w2031, "DisabledEnum"=w2032) -> (error out=w2034:errorcluster)  [unwired: 1 in, 1 out]
            n912 = property on="btnSave" class="Bool"(error in=w2034, "DisabledEnum"=w2032) -> (error out=w2033:errorcluster)  [unwired: 1 in, 1 out]
          }
          event Value Change {
            w2038 = T15."Enabled" ("Disabled")
            w2065 = FALSE ("StartMeas")
            # "Update Device(s)Settings"
            # "If the user changes the Synchronization setting, the AC instruments need to made available their adequate \"Change at\" angles depending on Mode."
            n913 = event-data() -> ("NewVal"=w2054:T3)  [unwired: 1 in]
            n914 = Equal To 0?(x=w2054) -> (x = 0?=w2056:bool)
            n915 = case shown="False" w2056 {
              selector: w2056 -> [w2067 w2070]
              tunnel: [T15."Enabled" ("Disabled") 2] -> w2055
              tunnel: w2052 -> [w2068 w2071]
              tunnel: [w2068 w2071] -> w2051
              tunnel: [w2067 w2070] -> w2049
              tunnel: [w2067 w2070] -> w2048
              tunnel: [w2067 w2070] -> w2047
              frame False {
              }
              frame True {
                # "2 = Disbaled and Greyed Out for short"
              }
            }
            n916 = local read "Mode"() -> (w2064:T8)
            n917 = case shown="0, Default" w2064 {
              tunnel: [w2116 w2158 w2199 w2232 w2250 w2271 w2301 w2331] -> w2061
              tunnel: [w2116 w2159 w2199 w2233 w2250 w2271 w2302 w2331] -> w2060
              tunnel: [w2116 w2159 w2199 w2233 w2250 T15."Disabled and Grayed Out" ("Disabled") w2302 w2331] -> w2059
              tunnel: [TRUE TRUE TRUE FALSE FALSE TRUE TRUE TRUE] -> w2063
              tunnel: [TRUE TRUE TRUE FALSE FALSE FALSE FALSE FALSE] -> w2062
              tunnel: [w2107 w2143 w2191 w2227 w2245 w2265 w2293 w2323] -> w2058
              tunnel: w2051 -> [w2102 w2146 w2187 w2226 w2244 w2261 w2291 w2321]
              tunnel: w2055 -> [w2116 w2158 _ w2232 _ w2271 w2301 _]
              tunnel: w2054 -> [w2109 w2150 w2192 w2229 w2247 w2266 w2296 w2326]
              tunnel: [w2103 w2144 w2185 w2226 w2244 w2264 w2292 w2322] -> w2050
              tunnel: w2049 -> [w2108 w2149 w2188 w2228 w2246 w2263 w2294 w2325]
              tunnel: w2048 -> [w2106 w2148 w2190 _ _ w2262 w2295 w2324]
              tunnel: w2047 -> [w2105 w2147 w2189 _ _ _ _ _]
              tunnel: [w2104 w2145 w2186 w2226 w2244 w2261 w2291 w2321] -> w2046
              frame 0, Default {
                # "The three instruments have to show the same Sync setting"
                # "Instr1 works as Instr1/2/3"
                # "Three-Phase enables all angles in all instruments"
                n918 = case shown="True" w2108 {
                  tunnel: [w2135 w2137] -> w2107
                  tunnel: w2102 -> [w2135 w2136]
                  frame False {
                  }
                  frame True {
                    n919 = property on="A-Change at..." class="DigNum (strict)"(error in=w2136, "Value"=0) -> (error out=w2142:errorcluster)  [unwired: 1 in, 1 out]
                    n920 = property on="B-Change at..." class="DigNum (strict)"(error in=w2142, "Value"=0) -> (error out=w2141:errorcluster)  [unwired: 1 in, 1 out]
                    n921 = property on="C-Change at..." class="DigNum (strict)"(error in=w2141, "Value"=0) -> (error out=w2137:errorcluster)  [unwired: 1 in, 1 out]
                  }
                }
                n922 = case shown="True" w2106 {
                  tunnel: w2102 -> [w2127 w2129]
                  tunnel: [w2127 w2128] -> w2103
                  frame False {
                  }
                  frame True {
                    n923 = property on="A-Change at..." class="DigNum (strict)"(error in=w2129, "Value"=0) -> (error out=w2134:errorcluster)  [unwired: 1 in, 1 out]
                    n924 = property on="B-Change at..." class="DigNum (strict)"(error in=w2134, "Value"=0) -> (error out=w2133:errorcluster)  [unwired: 1 in, 1 out]
                    n925 = property on="C-Change at..." class="DigNum (strict)"(error in=w2133, "Value"=0) -> (error out=w2128:errorcluster)  [unwired: 1 in, 1 out]
                  }
                }
                n926 = case shown="True" w2105 {
                  tunnel: w2102 -> [w2119 w2121]
                  tunnel: [w2119 w2120] -> w2104
                  frame False {
                  }
                  frame True {
                    n927 = property on="A-Change at..." class="DigNum (strict)"(error in=w2121, "Value"=0) -> (error out=w2126:errorcluster)  [unwired: 1 in, 1 out]
                    n928 = property on="B-Change at..." class="DigNum (strict)"(error in=w2126, "Value"=0) -> (error out=w2125:errorcluster)  [unwired: 1 in, 1 out]
                    n929 = property on="C-Change at..." class="DigNum (strict)"(error in=w2125, "Value"=0) -> (error out=w2120:errorcluster)  [unwired: 1 in, 1 out]
                  }
                }
                n930 = local read "Device(s)Settings"() -> (w2114:T1)
                n931 = Bundle By Name(cluster=w2114, "Instr1.Synchronization"=w2109, "Instr2.Synchronization"=w2109, "Instr3.Synchronization"=w2109) -> (w2115:T1)
                n932 = local read "Instr2"() -> (w2113:T2)
                n933 = Bundle By Name(cluster=w2113, "Synchronization"=w2109) -> (w2112:T2)
                n934 = local read "Instr3"() -> (w2110:T2)
                n935 = Bundle By Name(cluster=w2110, "Synchronization"=w2109) -> (w2111:T2)
                n936 = local write "Instr2"(w2112) -> ()
                n937 = local write "Instr3"(w2111) -> ()
                n938 = local write "Device(s)Settings"(w2115) -> ()
              }
              frame 1 {
                w2159 = T15."Disabled and Grayed Out" ("Disabled")
                # "The three instruments have to show the same Sync setting"
                # "Instr1 works as Instr1/2/3"
                # "Instr1 as one AC single-phase instrument"
                n939 = case shown="False" w2149 {
                  tunnel: [w2177 w2179] -> w2143
                  tunnel: w2146 -> [w2177 w2178]
                  frame False {
                  }
                  frame True {
                    n940 = property on="A-Change at..." class="DigNum (strict)"(error in=w2178, "Value"=0) -> (error out=w2184:errorcluster)  [unwired: 1 in, 1 out]
                    n941 = property on="B-Change at..." class="DigNum (strict)"(error in=w2184, "Value"=0) -> (error out=w2183:errorcluster)  [unwired: 1 in, 1 out]
                    n942 = property on="C-Change at..." class="DigNum (strict)"(error in=w2183, "Value"=0) -> (error out=w2179:errorcluster)  [unwired: 1 in, 1 out]
                  }
                }
                n943 = case shown="False" w2148 {
                  tunnel: w2146 -> [w2169 w2171]
                  tunnel: [w2169 w2170] -> w2144
                  frame False {
                  }
                  frame True {
                    n944 = property on="A-Change at..." class="DigNum (strict)"(error in=w2171, "Value"=0) -> (error out=w2176:errorcluster)  [unwired: 1 in, 1 out]
                    n945 = property on="B-Change at..." class="DigNum (strict)"(error in=w2176, "Value"=0) -> (error out=w2175:errorcluster)  [unwired: 1 in, 1 out]
                    n946 = property on="C-Change at..." class="DigNum (strict)"(error in=w2175, "Value"=0) -> (error out=w2170:errorcluster)  [unwired: 1 in, 1 out]
                  }
                }
                n947 = case shown="False" w2147 {
                  tunnel: w2146 -> [w2161 w2163]
                  tunnel: [w2161 w2162] -> w2145
                  frame False {
                  }
                  frame True {
                    n948 = property on="A-Change at..." class="DigNum (strict)"(error in=w2163, "Value"=0) -> (error out=w2168:errorcluster)  [unwired: 1 in, 1 out]
                    n949 = property on="B-Change at..." class="DigNum (strict)"(error in=w2168, "Value"=0) -> (error out=w2167:errorcluster)  [unwired: 1 in, 1 out]
                    n950 = property on="C-Change at..." class="DigNum (strict)"(error in=w2167, "Value"=0) -> (error out=w2162:errorcluster)  [unwired: 1 in, 1 out]
                  }
                }
                n951 = local read "Device(s)Settings"() -> (w2155:T1)
                n952 = Bundle By Name(cluster=w2155, "Instr1.Synchronization"=w2150, "Instr2.Synchronization"=w2150, "Instr3.Synchronization"=w2150) -> (w2156:T1)
                n953 = local read "Instr3"() -> (w2151:T2)
                n954 = Bundle By Name(cluster=w2151, "Synchronization"=w2150) -> (w2152:T2)
                n955 = local read "Instr2"() -> (w2154:T2)
                n956 = Bundle By Name(cluster=w2154, "Synchronization"=w2150) -> (w2153:T2)
                n957 = local write "Instr3"(w2152) -> ()
                n958 = local write "Instr2"(w2153) -> ()
                n959 = local write "Device(s)Settings"(w2156) -> ()
              }
              frame 2 {
                w2199 = T15."Disabled and Grayed Out" ("Disabled")
                # "The three instruments have to show the same Sync setting"
                # "Instr1 works as Instr1/2/3"
                # "Instr1 as one DC single-channel instrument"
                n960 = case shown="False" w2188 {
                  tunnel: [w2218 w2220] -> w2191
                  tunnel: w2187 -> [w2218 w2219]
                  frame False {
                  }
                  frame True {
                    n961 = property on="A-Change at..." class="DigNum (strict)"(error in=w2219, "Value"=0) -> (error out=w2225:errorcluster)  [unwired: 1 in, 1 out]
                    n962 = property on="B-Change at..." class="DigNum (strict)"(error in=w2225, "Value"=0) -> (error out=w2224:errorcluster)  [unwired: 1 in, 1 out]
                    n963 = property on="C-Change at..." class="DigNum (strict)"(error in=w2224, "Value"=0) -> (error out=w2220:errorcluster)  [unwired: 1 in, 1 out]
                  }
                }
                n964 = case shown="False" w2190 {
                  tunnel: w2187 -> [w2210 w2212]
                  tunnel: [w2210 w2211] -> w2185
                  frame False {
                  }
                  frame True {
                    n965 = property on="A-Change at..." class="DigNum (strict)"(error in=w2212, "Value"=0) -> (error out=w2217:errorcluster)  [unwired: 1 in, 1 out]
                    n966 = property on="B-Change at..." class="DigNum (strict)"(error in=w2217, "Value"=0) -> (error out=w2216:errorcluster)  [unwired: 1 in, 1 out]
                    n967 = property on="C-Change at..." class="DigNum (strict)"(error in=w2216, "Value"=0) -> (error out=w2211:errorcluster)  [unwired: 1 in, 1 out]
                  }
                }
                n968 = case shown="False" w2189 {
                  tunnel: w2187 -> [w2202 w2204]
                  tunnel: [w2202 w2203] -> w2186
                  frame False {
                  }
                  frame True {
                    n969 = property on="A-Change at..." class="DigNum (strict)"(error in=w2204, "Value"=0) -> (error out=w2209:errorcluster)  [unwired: 1 in, 1 out]
                    n970 = property on="B-Change at..." class="DigNum (strict)"(error in=w2209, "Value"=0) -> (error out=w2208:errorcluster)  [unwired: 1 in, 1 out]
                    n971 = property on="C-Change at..." class="DigNum (strict)"(error in=w2208, "Value"=0) -> (error out=w2203:errorcluster)  [unwired: 1 in, 1 out]
                  }
                }
                n972 = local read "Device(s)Settings"() -> (w2197:T1)
                n973 = Bundle By Name(cluster=w2197, "Instr1.Synchronization"=w2192, "Instr2.Synchronization"=w2192, "Instr3.Synchronization"=w2192) -> (w2198:T1)
                n974 = local read "Instr2"() -> (w2196:T2)
                n975 = Bundle By Name(cluster=w2196, "Synchronization"=w2192) -> (w2195:T2)
                n976 = local read "Instr3"() -> (w2193:T2)
                n977 = Bundle By Name(cluster=w2193, "Synchronization"=w2192) -> (w2194:T2)
                n978 = local write "Instr2"(w2195) -> ()
                n979 = local write "Instr3"(w2194) -> ()
                n980 = local write "Device(s)Settings"(w2198) -> ()
              }
              frame 3, 9, 10, 13 {
                w2233 = T15."Disabled and Grayed Out" ("Disabled")
                # "Pass the setting only to Instr1 in Device(s)Settings."
                # "Instr1 works independently"
                # "Instr1 alone as one AC single-phase instrument"
                n981 = case shown="True" w2228 {
                  tunnel: [w2236 w2238] -> w2227
                  tunnel: w2226 -> [w2236 w2237]
                  frame False {
                  }
                  frame True {
                    n982 = property on="A-Change at..." class="DigNum (strict)"(error in=w2237, "Value"=0) -> (error out=w2243:errorcluster)  [unwired: 1 in, 1 out]
                    n983 = property on="B-Change at..." class="DigNum (strict)"(error in=w2243, "Value"=0) -> (error out=w2242:errorcluster)  [unwired: 1 in, 1 out]
                    n984 = property on="C-Change at..." class="DigNum (strict)"(error in=w2242, "Value"=0) -> (error out=w2238:errorcluster)  [unwired: 1 in, 1 out]
                  }
                }
                n985 = local read "Device(s)Settings"() -> (w2230:T1)
                n986 = Bundle By Name(cluster=w2230, "Instr1.Synchronization"=w2229) -> (w2231:T1)
                n987 = local write "Device(s)Settings"(w2231) -> ()
              }
              frame 4, 14, 15 {
                w2250 = T15."Disabled and Grayed Out" ("Disabled")
                # "Pass the setting only to Instr1 in Device(s)Settings."
                # "Instr1 works independently"
                # "Instr1 alone as one DC single-channel instrument"
                n988 = case shown="False" w2246 {
                  tunnel: [w2253 w2255] -> w2245
                  tunnel: w2244 -> [w2253 w2254]
                  frame False {
                  }
                  frame True {
                    n989 = property on="A-Change at..." class="DigNum (strict)"(error in=w2254, "Value"=0) -> (error out=w2260:errorcluster)  [unwired: 1 in, 1 out]
                    n990 = property on="B-Change at..." class="DigNum (strict)"(error in=w2260, "Value"=0) -> (error out=w2259:errorcluster)  [unwired: 1 in, 1 out]
                    n991 = property on="C-Change at..." class="DigNum (strict)"(error in=w2259, "Value"=0) -> (error out=w2255:errorcluster)  [unwired: 1 in, 1 out]
                  }
                }
                n992 = local read "Device(s)Settings"() -> (w2248:T1)
                n993 = Bundle By Name(cluster=w2248, "Instr1.Synchronization"=w2247) -> (w2249:T1)
                n994 = local write "Device(s)Settings"(w2249) -> ()
              }
              frame 5, 6 {
                # "Pass only Instr1 and Instr2 settings to Device(s)Settings."
                # "Instr1 works as Instr1/2 only"
                # "Instr1/Instr2 as one AC Two-Phase instrument"
                n995 = case shown="False" w2263 {
                  tunnel: [w2283 w2285] -> w2265
                  tunnel: w2261 -> [w2283 w2284]
                  frame False {
                  }
                  frame True {
                    n996 = property on="A-Change at..." class="DigNum (strict)"(error in=w2284, "Value"=0) -> (error out=w2290:errorcluster)  [unwired: 1 in, 1 out]
                    n997 = property on="B-Change at..." class="DigNum (strict)"(error in=w2290, "Value"=0) -> (error out=w2289:errorcluster)  [unwired: 1 in, 1 out]
                    n998 = property on="C-Change at..." class="DigNum (strict)"(error in=w2289, "Value"=0) -> (error out=w2285:errorcluster)  [unwired: 1 in, 1 out]
                  }
                }
                n999 = local read "Device(s)Settings"() -> (w2269:T1)
                n1000 = Bundle By Name(cluster=w2269, "Instr1.Synchronization"=w2266, "Instr2.Synchronization"=w2266) -> (w2270:T1)
                n1001 = case shown="False" w2262 {
                  tunnel: w2261 -> [w2275 w2277]
                  tunnel: [w2275 w2276] -> w2264
                  frame False {
                  }
                  frame True {
                    n1002 = property on="A-Change at..." class="DigNum (strict)"(error in=w2277, "Value"=0) -> (error out=w2282:errorcluster)  [unwired: 1 in, 1 out]
                    n1003 = property on="B-Change at..." class="DigNum (strict)"(error in=w2282, "Value"=0) -> (error out=w2281:errorcluster)  [unwired: 1 in, 1 out]
                    n1004 = property on="C-Change at..." class="DigNum (strict)"(error in=w2281, "Value"=0) -> (error out=w2276:errorcluster)  [unwired: 1 in, 1 out]
                  }
                }
                n1005 = local read "Instr2"() -> (w2268:T2)
                n1006 = Bundle By Name(cluster=w2268, "Synchronization"=w2266) -> (w2267:T2)
                n1007 = local write "Instr2"(w2267) -> ()
                n1008 = local write "Device(s)Settings"(w2270) -> ()
              }
              frame 7, 8 {
                w2302 = T15."Disabled and Grayed Out" ("Disabled")
                # "Pass only Instr1 and Instr2 settings to Device(s)Settings."
                # "Instr1 works as Instr1/2 only"
                # "Instr1/Instr2 as one AC single-phase instrument"
                n1009 = case shown="False" w2294 {
                  tunnel: [w2313 w2315] -> w2293
                  tunnel: w2291 -> [w2313 w2314]
                  frame False {
                  }
                  frame True {
                    n1010 = property on="A-Change at..." class="DigNum (strict)"(error in=w2314, "Value"=0) -> (error out=w2320:errorcluster)  [unwired: 1 in, 1 out]
                    n1011 = property on="B-Change at..." class="DigNum (strict)"(error in=w2320, "Value"=0) -> (error out=w2319:errorcluster)  [unwired: 1 in, 1 out]
                    n1012 = property on="C-Change at..." class="DigNum (strict)"(error in=w2319, "Value"=0) -> (error out=w2315:errorcluster)  [unwired: 1 in, 1 out]
                  }
                }
                n1013 = case shown="False" w2295 {
                  tunnel: w2291 -> [w2305 w2307]
                  tunnel: [w2305 w2306] -> w2292
                  frame False {
                  }
                  frame True {
                    n1014 = property on="A-Change at..." class="DigNum (strict)"(error in=w2307, "Value"=0) -> (error out=w2312:errorcluster)  [unwired: 1 in, 1 out]
                    n1015 = property on="B-Change at..." class="DigNum (strict)"(error in=w2312, "Value"=0) -> (error out=w2311:errorcluster)  [unwired: 1 in, 1 out]
                    n1016 = property on="C-Change at..." class="DigNum (strict)"(error in=w2311, "Value"=0) -> (error out=w2306:errorcluster)  [unwired: 1 in, 1 out]
                  }
                }
                n1017 = local read "Device(s)Settings"() -> (w2299:T1)
                n1018 = Bundle By Name(cluster=w2299, "Instr1.Synchronization"=w2296, "Instr2.Synchronization"=w2296) -> (w2300:T1)
                n1019 = local read "Instr2"() -> (w2298:T2)
                n1020 = Bundle By Name(cluster=w2298, "Synchronization"=w2296) -> (w2297:T2)
                n1021 = local write "Instr2"(w2297) -> ()
                n1022 = local write "Device(s)Settings"(w2300) -> ()
              }
              frame 11, 12 {
                w2331 = T15."Disabled and Grayed Out" ("Disabled")
                # "Pass only Instr1 and Instr2 settings to Device(s)Settings."
                # "Instr1 works as Instr1/2 only"
                # "Instr1/Instr2 as one DC single-channel instrument"
                n1023 = case shown="False" w2325 {
                  tunnel: [w2342 w2344] -> w2323
                  tunnel: w2321 -> [w2342 w2343]
                  frame False {
                  }
                  frame True {
                    n1024 = property on="A-Change at..." class="DigNum (strict)"(error in=w2343, "Value"=0) -> (error out=w2349:errorcluster)  [unwired: 1 in, 1 out]
                    n1025 = property on="B-Change at..." class="DigNum (strict)"(error in=w2349, "Value"=0) -> (error out=w2348:errorcluster)  [unwired: 1 in, 1 out]
                    n1026 = property on="C-Change at..." class="DigNum (strict)"(error in=w2348, "Value"=0) -> (error out=w2344:errorcluster)  [unwired: 1 in, 1 out]
                  }
                }
                n1027 = case shown="False" w2324 {
                  tunnel: w2321 -> [w2334 w2336]
                  tunnel: [w2334 w2335] -> w2322
                  frame False {
                  }
                  frame True {
                    n1028 = property on="A-Change at..." class="DigNum (strict)"(error in=w2336, "Value"=0) -> (error out=w2341:errorcluster)  [unwired: 1 in, 1 out]
                    n1029 = property on="B-Change at..." class="DigNum (strict)"(error in=w2341, "Value"=0) -> (error out=w2340:errorcluster)  [unwired: 1 in, 1 out]
                    n1030 = property on="C-Change at..." class="DigNum (strict)"(error in=w2340, "Value"=0) -> (error out=w2335:errorcluster)  [unwired: 1 in, 1 out]
                  }
                }
                n1031 = local read "Device(s)Settings"() -> (w2329:T1)
                n1032 = Bundle By Name(cluster=w2329, "Instr1.Synchronization"=w2326, "Instr2.Synchronization"=w2326) -> (w2330:T1)
                n1033 = local read "Instr2"() -> (w2328:T2)
                n1034 = Bundle By Name(cluster=w2328, "Synchronization"=w2326) -> (w2327:T2)
                n1035 = local write "Instr2"(w2327) -> ()
                n1036 = local write "Device(s)Settings"(w2330) -> ()
              }
            }
            n1037 = flat-sequence {
              tunnel: w2063 -> [w2083]
              tunnel: w2062 -> [w2082]
              tunnel: w2061 -> [w2081]
              tunnel: w2060 -> [w2080]
              tunnel: w2059 -> [w2079]
              tunnel: w2058 -> [w2078]
              tunnel: w2050 -> [w2076]
              tunnel: w2046 -> [w2077]
              tunnel: [w2075] -> w2045
              tunnel: [w2074] -> w2044
              tunnel: [w2073] -> w2043
              frame #0 {
                # "Enable/Disable the \"Change at\" controls as required."
                # "Instr1"
                n1038 = case shown="False" w2083 {
                  tunnel: w2081 -> [_ w2099]
                  tunnel: w2080 -> [_ w2098]
                  tunnel: w2079 -> [_ w2097]
                  tunnel: w2076 -> [w2094 w2096]
                  tunnel: [w2094 w2095] -> w2074
                  frame False {
                    # "Don't make any changes to Instr2"
                  }
                  frame True {
                    # "Instr2"
                    n1039 = property on="A-Change at..." class="DigNum (strict)"(error in=w2096, "DisabledEnum"=w2099) -> (error out=w2100:errorcluster)  [unwired: 1 in, 1 out]
                    n1040 = property on="B-Change at..." class="DigNum (strict)"(error in=w2100, "DisabledEnum"=w2098) -> (error out=w2101:errorcluster)  [unwired: 1 in, 1 out]
                    n1041 = property on="C-Change at..." class="DigNum (strict)"(error in=w2101, "DisabledEnum"=w2097) -> (error out=w2095:errorcluster)  [unwired: 1 in, 1 out]
                  }
                }
                n1042 = case shown="False" w2082 {
                  tunnel: w2081 -> [_ w2091]
                  tunnel: w2080 -> [_ w2090]
                  tunnel: w2079 -> [_ w2089]
                  tunnel: w2077 -> [w2086 w2088]
                  tunnel: [w2086 w2087] -> w2075
                  frame False {
                    # "Don't make any changes to Instr3"
                  }
                  frame True {
                    # "Instr3"
                    n1043 = property on="A-Change at..." class="DigNum (strict)"(error in=w2088, "DisabledEnum"=w2091) -> (error out=w2092:errorcluster)  [unwired: 1 in, 1 out]
                    n1044 = property on="B-Change at..." class="DigNum (strict)"(error in=w2092, "DisabledEnum"=w2090) -> (error out=w2093:errorcluster)  [unwired: 1 in, 1 out]
                    n1045 = property on="C-Change at..." class="DigNum (strict)"(error in=w2093, "DisabledEnum"=w2089) -> (error out=w2087:errorcluster)  [unwired: 1 in, 1 out]
                  }
                }
                n1046 = property on="A-Change at..." class="DigNum (strict)"(error in=w2078, "DisabledEnum"=w2081) -> (error out=w2084:errorcluster)  [unwired: 1 in, 1 out]
                n1047 = property on="B-Change at..." class="DigNum (strict)"(error in=w2084, "DisabledEnum"=w2080) -> (error out=w2085:errorcluster)  [unwired: 1 in, 1 out]
                n1048 = property on="C-Change at..." class="DigNum (strict)"(error in=w2085, "DisabledEnum"=w2079) -> (error out=w2073:errorcluster)  [unwired: 1 in, 1 out]
              }
            }
            n1049 = property on="Update" class="Bool (strict)"(error in=w2043) -> (error out=w2057:errorcluster, "Value"=w2053:bool)  [unwired: 1 in, 1 out]
            n1050 = property on="Update" class="Bool (strict)"(error in=w2057, "Val(Sgnl)"=w2053) -> (error out=w2041:errorcluster)  [unwired: 1 in, 1 out]
            n1051 = property on="btnSaveAs" class="Bool"(error in=w2044, "DisabledEnum"=w2038) -> (error out=w2040:errorcluster)  [unwired: 1 in, 1 out]
            n1052 = property on="btnSave" class="Bool"(error in=w2045, "DisabledEnum"=w2038) -> (error out=w2039:errorcluster)  [unwired: 1 in, 1 out]
            n1053 = Merge Errors(w2041, w2040, w2039) -> (w2042:errorcluster)
          }
          event Value Change {
            w2365 = T15."Enabled" ("Disabled")
            w2368 = FALSE ("StartMeas")
            # "If the index selection for the control is not equal to zero, it means that the option is not \"Immediate\" and then the adequate \"Change at\" controls need to be made available."
            # "Since these are properties of the \"Change at\" controls, and not their values, they'll be registered using the \"Update Device(s)Settings\" procedure so that this case doesn't get too complicated in structure."
            # "Update Device(s)Settings"
            # "The user can only access the Synchronization control in Instr2 when it is working as a separate instrument in its own panel. Otherwise, Instr1 is overriding it and already took care of Instr2 settings."
            n1054 = event-data() -> ("NewVal"=w2353:T3)  [unwired: 1 in]
            n1055 = Not Equal To 0?(x=w2353) -> (x != 0?=w2355:bool)
            n1056 = case shown="False" w2355 {
              tunnel: [T15."Disabled and Grayed Out" ("Disabled") T15."Enabled" ("Disabled")] -> w2354
              tunnel: [w2379 w2386] -> w2351
              tunnel: w2350 -> [w2378 w2386]
              frame False {
                # "Reset all to 0 if it becomes \"Immediate\""
                n1057 = property on="A-Change at..." class="DigNum (strict)"(error in=w2378, "Value"=0) -> (error out=w2384:errorcluster)  [unwired: 1 in, 1 out]
                n1058 = property on="B-Change at..." class="DigNum (strict)"(error in=w2384, "Value"=0) -> (error out=w2383:errorcluster)  [unwired: 1 in, 1 out]
                n1059 = property on="C-Change at..." class="DigNum (strict)"(error in=w2383, "Value"=0) -> (error out=w2379:errorcluster)  [unwired: 1 in, 1 out]
              }
              frame True {
              }
            }
            n1060 = local read "Mode"() -> (w2364:T8)
            n1061 = case shown="4, 10, 13" w2364 {
              tunnel: [w2389 w2392 w2395] -> w2362
              tunnel: [w2389 w2391 w2395] -> w2361
              tunnel: [w2389 w2391 w2395] -> w2360
              tunnel: [FALSE TRUE TRUE] -> w2363
              tunnel: [w2388 w2393 w2396] -> w2359
              tunnel: w2351 -> [w2388 w2393 w2396]
              tunnel: w2354 -> [_ w2392 _]
              frame Default {
                w2389 = T15."Enabled" ("Disabled")
                # "Instr2 is overriden by Instr1. No changes will be done to Instr2."
                # "Modes where Instr2 is not working by itself"
              }
              frame 3, 9, 14, 15 {
                w2391 = T15."Disabled and Grayed Out" ("Disabled")
                # "Modes where Instr2 is AC and available"
              }
              frame 4, 10, 13 {
                w2395 = T15."Disabled and Grayed Out" ("Disabled")
                # "Modes where Instr2 is DC and available"
              }
            }
            n1062 = case shown="True" w2363 {
              tunnel: w2362 -> [_ w2375]
              tunnel: w2361 -> [_ w2374]
              tunnel: w2360 -> [_ w2373]
              tunnel: w2359 -> [w2370 w2372]
              tunnel: [w2370 w2371] -> w2356
              frame False {
                # "Don't make any changes to Instr2"
              }
              frame True {
                # "Instr2"
                n1063 = property on="A-Change at..." class="DigNum (strict)"(error in=w2372, "DisabledEnum"=w2375) -> (error out=w2376:errorcluster)  [unwired: 1 in, 1 out]
                n1064 = property on="B-Change at..." class="DigNum (strict)"(error in=w2376, "DisabledEnum"=w2374) -> (error out=w2377:errorcluster)  [unwired: 1 in, 1 out]
                n1065 = property on="C-Change at..." class="DigNum (strict)"(error in=w2377, "DisabledEnum"=w2373) -> (error out=w2371:errorcluster)  [unwired: 1 in, 1 out]
              }
            }
            n1066 = property on="Update" class="Bool (strict)"(error in=w2356) -> (error out=w2358:errorcluster, "Value"=w2352:bool)  [unwired: 1 in, 1 out]
            n1067 = property on="Update" class="Bool (strict)"(error in=w2358, "Val(Sgnl)"=w2352) -> (error out=w2357:errorcluster)  [unwired: 1 in, 1 out]
            n1068 = property on="btnSaveAs" class="Bool"(error in=w2357, "DisabledEnum"=w2365) -> (error out=w2367:errorcluster)  [unwired: 1 in, 1 out]
            n1069 = property on="btnSave" class="Bool"(error in=w2367, "DisabledEnum"=w2365) -> (error out=w2366:errorcluster)  [unwired: 1 in, 1 out]
          }
          event Value Change {
            w2413 = T15."Enabled" ("Disabled")
            w2416 = FALSE ("StartMeas")
            # "If the index selection for the control is not equal to zero, it means that the option is not \"Immediate\" and then the adequate \"Change at\" controls need to be made available."
            # "Since these are properties of the \"Change at\" controls, and not their values, they'll be registered using the \"Update Device(s)Settings\" procedure so that this case doesn't get too complicated in structure."
            # "Update Device(s)Settings"
            # "Instr3 is available to the user most of the time to be able to change the Synchronization setting, except when Instr3 is overriden by Instr1."
            n1070 = event-data() -> ("NewVal"=w2401:T3)  [unwired: 1 in]
            n1071 = Not Equal To 0?(x=w2401) -> (x != 0?=w2403:bool)
            n1072 = case shown="False" w2403 {
              tunnel: [T15."Disabled and Grayed Out" ("Disabled") T15."Enabled" ("Disabled")] -> w2402
              tunnel: [w2426 w2434] -> w2399
              tunnel: w2398 -> [w2427 w2434]
              frame False {
                # "Reset all to 0 if it becomes \"Immediate\""
                n1073 = property on="A-Change at..." class="DigNum (strict)"(error in=w2427, "Value"=0) -> (error out=w2432:errorcluster)  [unwired: 1 in, 1 out]
                n1074 = property on="B-Change at..." class="DigNum (strict)"(error in=w2432, "Value"=0) -> (error out=w2431:errorcluster)  [unwired: 1 in, 1 out]
                n1075 = property on="C-Change at..." class="DigNum (strict)"(error in=w2431, "Value"=0) -> (error out=w2426:errorcluster)  [unwired: 1 in, 1 out]
              }
              frame True {
              }
            }
            n1076 = local read "Mode"() -> (w2412:T8)
            n1077 = case shown="0..2, Default" w2412 {
              tunnel: [w2437 w2440 w2443] -> w2410
              tunnel: [w2437 w2439 w2443] -> w2409
              tunnel: [w2437 w2439 w2443] -> w2408
              tunnel: [FALSE TRUE TRUE] -> w2411
              tunnel: [w2436 w2441 w2444] -> w2407
              tunnel: w2399 -> [w2436 w2441 w2444]
              tunnel: w2402 -> [_ w2440 _]
              frame 0..2, Default {
                w2437 = T15."Enabled" ("Disabled")
                # "Instr3 is overriden by Instr1. No changes will be done to Instr3."
                # "Modes where Instr3 is not working by itself"
              }
              frame 3, 5, 7, 11, 13, 14 {
                w2439 = T15."Disabled and Grayed Out" ("Disabled")
                # "Modes where Instr3 is AC and available"
              }
              frame 4, 6, 8..10, 12, 15 {
                w2443 = T15."Disabled and Grayed Out" ("Disabled")
                # "Modes where Instr3 is DC and available"
              }
            }
            n1078 = case shown="True" w2411 {
              tunnel: w2410 -> [_ w2423]
              tunnel: w2409 -> [_ w2422]
              tunnel: w2408 -> [_ w2421]
              tunnel: w2407 -> [w2418 w2420]
              tunnel: [w2418 w2419] -> w2404
              frame False {
                # "Don't make any changes to Instr3"
              }
              frame True {
                # "Instr3"
                n1079 = property on="A-Change at..." class="DigNum (strict)"(error in=w2420, "DisabledEnum"=w2423) -> (error out=w2424:errorcluster)  [unwired: 1 in, 1 out]
                n1080 = property on="B-Change at..." class="DigNum (strict)"(error in=w2424, "DisabledEnum"=w2422) -> (error out=w2425:errorcluster)  [unwired: 1 in, 1 out]
                n1081 = property on="C-Change at..." class="DigNum (strict)"(error in=w2425, "DisabledEnum"=w2421) -> (error out=w2419:errorcluster)  [unwired: 1 in, 1 out]
              }
            }
            n1082 = property on="Update" class="Bool (strict)"(error in=w2404) -> (error out=w2406:errorcluster, "Value"=w2400:bool)  [unwired: 1 in, 1 out]
            n1083 = property on="Update" class="Bool (strict)"(error in=w2406, "Val(Sgnl)"=w2400) -> (error out=w2405:errorcluster)  [unwired: 1 in, 1 out]
            n1084 = property on="btnSaveAs" class="Bool"(error in=w2405, "DisabledEnum"=w2413) -> (error out=w2415:errorcluster)  [unwired: 1 in, 1 out]
            n1085 = property on="btnSave" class="Bool"(error in=w2415, "DisabledEnum"=w2413) -> (error out=w2414:errorcluster)  [unwired: 1 in, 1 out]
          }
          event Value Change {
            w2453 = T15."Enabled" ("Disabled")
            w2456 = FALSE ("StartMeas")
            # "Aperture change is a value that does not affect others for the instrument. It only needs to be saved."
            n1086 = event-data() -> ()  [unwired: 1 in, 6 out]
            n1087 = local read "Mode"() -> (w2452:T8)
            n1088 = case shown="Default" w2452 {
              tunnel: [w2458 w2461 w2466] -> w2449
              tunnel: [w2458 w2460 w2465] -> w2448
              tunnel: [w2458 w2460 w2464] -> w2447
              frame 0..2 {
                # "Cases with Instr1 only"
                n1089 = local read "Instr1"() -> (w2459:T2)
                n1090 = Unbundle By Name(w2459) -> ("Aperture (cycles)"=w2458:i32)
              }
              frame 5..8, 11, 12 {
                # "Cases with Instr1 and Instr3"
                n1091 = local read "Instr1"() -> (w2463:T2)
                n1092 = local read "Instr3"() -> (w2462:T2)
                n1093 = Unbundle By Name(w2463) -> ("Aperture (cycles)"=w2460:i32)
                n1094 = Unbundle By Name(w2462) -> ("Aperture (cycles)"=w2461:i32)
              }
              frame Default {
                # "Cases with all instruments"
                n1095 = local read "Instr1"() -> (w2469:T2)
                n1096 = local read "Instr2"() -> (w2468:T2)
                n1097 = local read "Instr3"() -> (w2467:T2)
                n1098 = Unbundle By Name(w2468) -> ("Aperture (cycles)"=w2465:i32)
                n1099 = Unbundle By Name(w2469) -> ("Aperture (cycles)"=w2464:i32)
                n1100 = Unbundle By Name(w2467) -> ("Aperture (cycles)"=w2466:i32)
              }
            }
            n1101 = local read "Device(s)Settings"() -> (w2450:T1)
            n1102 = Bundle By Name(cluster=w2450, "Instr1.Aperture (cycles)"=w2447, "Instr2.Aperture (cycles)"=w2448, "Instr3.Aperture (cycles)"=w2449) -> (w2451:T1)
            n1103 = local write "Device(s)Settings"(w2451) -> ()
            n1104 = property on="btnSaveAs" class="Bool"(error in=w2446, "DisabledEnum"=w2453) -> (error out=w2455:errorcluster)  [unwired: 1 in, 1 out]
            n1105 = property on="btnSave" class="Bool"(error in=w2455, "DisabledEnum"=w2453) -> (error out=w2454:errorcluster)  [unwired: 1 in, 1 out]
          }
          event Value Change {
            w2477 = T15."Enabled" ("Disabled")
            w2480 = FALSE ("StartMeas")
            # "Frequency only affects AC instruments, so this event can only be activated depending on instrument and Mode.\n\"Mode change\" event already took care of enabling/disabling the Frequency controls in the different modes and instrumenst as needed."
            # "Frequency change is a value that does not affect others in the instrument. It only needs to be saved."
            n1106 = event-data() -> ()  [unwired: 1 in, 6 out]
            n1107 = local read "Mode"() -> (w2476:T8)
            n1108 = case shown="5..8, 11, 12" w2476 {
              tunnel: [w2482 w2485 w2490] -> w2473
              tunnel: [w2482 w2484 w2489] -> w2472
              tunnel: [w2482 w2484 w2488] -> w2471
              frame 0..2 {
                # "Cases with Instr1 only"
                n1109 = local read "Instr1"() -> (w2483:T2)
                n1110 = Unbundle By Name(w2483) -> ("FreqOut (Hz)"=w2482:dbl)
              }
              frame 5..8, 11, 12 {
                # "Cases with Instr1 and Instr3"
                n1111 = local read "Instr1"() -> (w2487:T2)
                n1112 = local read "Instr3"() -> (w2486:T2)
                n1113 = Unbundle By Name(w2487) -> ("FreqOut (Hz)"=w2484:dbl)
                n1114 = Unbundle By Name(w2486) -> ("FreqOut (Hz)"=w2485:dbl)
              }
              frame Default {
                # "Cases with all instruments"
                n1115 = local read "Instr1"() -> (w2493:T2)
                n1116 = local read "Instr2"() -> (w2492:T2)
                n1117 = local read "Instr3"() -> (w2491:T2)
                n1118 = Unbundle By Name(w2492) -> ("FreqOut (Hz)"=w2489:dbl)
                n1119 = Unbundle By Name(w2493) -> ("FreqOut (Hz)"=w2488:dbl)
                n1120 = Unbundle By Name(w2491) -> ("FreqOut (Hz)"=w2490:dbl)
              }
            }
            n1121 = local read "Device(s)Settings"() -> (w2474:T1)
            n1122 = Bundle By Name(cluster=w2474, "Instr1.FreqOut (Hz)"=w2471, "Instr2.FreqOut (Hz)"=w2472, "Instr3.FreqOut (Hz)"=w2473) -> (w2475:T1)
            n1123 = local write "Device(s)Settings"(w2475) -> ()
            n1124 = property on="btnSaveAs" class="Bool"(error in=w2470, "DisabledEnum"=w2477) -> (error out=w2479:errorcluster)  [unwired: 1 in, 1 out]
            n1125 = property on="btnSave" class="Bool"(error in=w2479, "DisabledEnum"=w2477) -> (error out=w2478:errorcluster)  [unwired: 1 in, 1 out]
          }
          event Value Change {
            w2501 = T15."Enabled" ("Disabled")
            w2504 = FALSE ("StartMeas")
            # "Pass all the values in the Safety Trips cluster of each Instrument to their Device(s)Settings counterparts"
            n1126 = event-data() -> ()  [unwired: 1 in, 6 out]
            n1127 = local read "Mode"() -> (w2499:T8)
            n1128 = case shown="0..2" w2499 {
              tunnel: [w2506 w2509 w2514] -> w2496
              tunnel: [w2506 w2508 w2513] -> w2495
              tunnel: [w2506 w2508 w2512] -> w2494
              frame 0..2 {
                # "Cases with Instr1 only"
                n1129 = local read "Instr1"() -> (w2507:T2)
                n1130 = Unbundle By Name(w2507) -> ("Safety Trips"=w2506:T5)
              }
              frame 5..8, 11, 12 {
                # "Cases with Instr1 and Instr3"
                n1131 = local read "Instr1"() -> (w2511:T2)
                n1132 = local read "Instr3"() -> (w2510:T2)
                n1133 = Unbundle By Name(w2511) -> ("Safety Trips"=w2508:T5)
                n1134 = Unbundle By Name(w2510) -> ("Safety Trips"=w2509:T5)
              }
              frame Default {
                # "Cases with all instruments"
                n1135 = local read "Instr1"() -> (w2517:T2)
                n1136 = local read "Instr2"() -> (w2516:T2)
                n1137 = local read "Instr3"() -> (w2515:T2)
                n1138 = Unbundle By Name(w2516) -> ("Safety Trips"=w2513:T5)
                n1139 = Unbundle By Name(w2517) -> ("Safety Trips"=w2512:T5)
                n1140 = Unbundle By Name(w2515) -> ("Safety Trips"=w2514:T5)
              }
            }
            n1141 = local read "Device(s)Settings"() -> (w2497:T1)
            n1142 = Bundle By Name(cluster=w2497, "Instr1.Safety Trips"=w2494, "Instr2.Safety Trips"=w2495, "Instr3.Safety Trips"=w2496) -> (w2498:T1)
            n1143 = local write "Device(s)Settings"(w2498) -> ()
            n1144 = property on="btnSaveAs" class="Bool"(error in=w2500, "DisabledEnum"=w2501) -> (error out=w2503:errorcluster)  [unwired: 1 in, 1 out]
            n1145 = property on="btnSave" class="Bool"(error in=w2503, "DisabledEnum"=w2501) -> (error out=w2502:errorcluster)  [unwired: 1 in, 1 out]
          }
          event "Handle", "MeasName", "ID Query", "Reset": Value Change {
            w2523 = T15."Enabled" ("Disabled")
            w2525 = FALSE ("StartMeas")
            # "The \"Update\" event call takes care of saving any changed controls"
            # "Update Device(s)Settings"
            # "These controls may be passed just as they are without processing or verification"
            n1146 = event-data() -> ()  [unwired: 1 in, 6 out]
            n1147 = property on="btnSave" class="Bool"(error in=w2520, "DisabledEnum"=w2523) -> (error out=w2522:errorcluster)  [unwired: 1 in, 1 out]
            n1148 = property on="btnSaveAs" class="Bool"(error in=w2522, "DisabledEnum"=w2523) -> (error out=w2521:errorcluster)  [unwired: 1 in, 1 out]
            n1149 = property on="Update" class="Bool (strict)"(error in=w2521) -> (error out=w2524:errorcluster, "Value"=w2518:bool)  [unwired: 1 in, 1 out]
            n1150 = property on="Update" class="Bool (strict)"(error in=w2524, "Val(Sgnl)"=w2518) -> (error out=w2519:errorcluster)  [unwired: 1 in, 1 out]
          }
          event "Measurement RefreshTime (ms)": Value Change {
            w2529 = T15."Enabled" ("Disabled")
            w2539 = FALSE
            # "Enable the [Save]  and [Save as] buttons if the configuration is saved."
            n1151 = event-data() -> ()  [unwired: 1 in, 1 out]
            n1152 = local read "Device(s)Settings"() -> (w2533:T1)
            n1153 = To Variant(anything=w2533) -> (Variant=w2537:variant)
            n1154 = To Variant(anything="Measurements") -> (Variant=w2534:variant)
            n1155 = call-dynamic "WriteToBaseConfigVariant.vi"("Measurement RefreshTime (ms)"="Measurement RefreshTime (ms)", "error in (no error)"=w2532, "Meas"=w2534, "Config"=w2537, "NHRGridSim in"=w2538) -> ("error out"=w2530:errorcluster, "NHRGridSim out"=w2531:refnum<class "NHRGridSim.lvclass">)  [unwired: 5 in]
            n1156 = property on="btnSave" class="Bool"(error in=w2530, "DisabledEnum"=w2529) -> (error out=w2528:errorcluster)  [unwired: 1 in, 1 out]
            n1157 = property on="btnSaveAs" class="Bool"(error in=w2528, "DisabledEnum"=w2529) -> (error out=w2527:errorcluster)  [unwired: 1 in, 1 out]
          }
          event Value Change {
            w2558 = T15."Enabled" ("Disabled")
            w2561 = FALSE ("StartMeas")
            # "For Instr1 the values of the phases must follow the value of Vout depending on being Three-Phase or Two-Phase mode. The rest of the modes are all for Single-Phase (AC) or Single-Channel (DC) instruments. The frame is to make sure that Instr1, Instr2 and Instr3 get updated before their changes are registered into their Device(s)Settings counterparts."
            # "Instr1"
            # "Turn indexed string into numeric."
            # "Get the present limits that the V Range control has, and the index of the present range selection."
            # "Update Device(s)Settings"
            # "When Vout is changed for Instr1, it requires more management than the other instruments because phases may be involved, and Instr1 may be overriding Instr2 and Instr3 too depending on Mode."
            n1158 = event-data() -> ("NewVal"=w2541:dbl)  [unwired: 1 in]
            n1159 = property on="Voltage (V)" class="Ring (strict)"(error in=w2550) -> (error out=w2554:errorcluster, "Strings []"=w2555:string[], "Value"=w2552:u16)  [unwired: 1 in, 1 out]
            n1160 = Index Array(array=w2555, index=w2552) -> (element=w2553:string)
            n1161 = Scan From String(format string="%f", input string=w2553, error in=w2554) -> (error out=w2545:errorcluster, output 1=w2542:dbl)  [unwired: 2 in, 2 out]
            n1162 = local read "Mode"() -> (w2540:T8)
            n1163 = Less?(x=w2542, y=w2541) -> (x < y?=w2543:bool)
            n1164 = Merge Errors(w2550, w2545) -> (w2549:errorcluster)
            n1165 = case shown="True" w2543 {
              tunnel: w2540 -> [_ w2609]
              frame False {
                # "No voltage range adjustment needed. Vout falls within present range."
              }
              frame True {
                w2608 = u16 1 ("Ranges.Voltage (V)")
                # "Increase range so that Vout can fit within it."
                n1166 = case shown="0..2" w2609 {
                  tunnel: w2608 -> [w2612 w2617 _]
                  frame 0..2 {
                    # "Instr1 overrides Instr2 and Instr3."
                    n1167 = local read "Instr2"() -> (w2615:T2)
                    n1168 = Bundle By Name(cluster=w2615, "Ranges.Voltage (V)"=w2612) -> (w2616:T2)
                    n1169 = local read "Instr3"() -> (w2614:T2)
                    n1170 = Bundle By Name(cluster=w2614, "Ranges.Voltage (V)"=w2612) -> (w2613:T2)
                    n1171 = local write "Instr2"(w2616) -> ()
                    n1172 = local write "Instr3"(w2613) -> ()
                  }
                  frame 5..8, 11, 12 {
                    # "Instr1 overrides Instr2 only."
                    n1173 = local read "Instr2"() -> (w2618:T2)
                    n1174 = Bundle By Name(cluster=w2618, "Ranges.Voltage (V)"=w2617) -> (w2619:T2)
                    n1175 = local write "Instr2"(w2619) -> ()
                  }
                  frame Default {
                    # "Neither Instr2 nor Instr3 are affected by Instr1 settings."
                    # "Instr1 is a single instrument itself."
                  }
                }
                n1176 = local read "Instr1"() -> (w2611:T2)
                n1177 = Bundle By Name(cluster=w2611, "Ranges.Voltage (V)"=w2608) -> (w2610:T2)
                n1178 = local write "Instr1"(w2610) -> ()
              }
            }
            n1179 = local read "Mode"() -> (w2546:T8)
            n1180 = flat-sequence {
              tunnel: w2541 -> [w2564]
              tunnel: w2549 -> [w2565]
              tunnel: [w2565] -> w2548
              tunnel: w2546 -> [w2563]
              frame #0 {
                n1181 = case shown="0" w2563 {
                  tunnel: w2564 -> [w2588 w2593 w2599 w2602 w2607]
                  tunnel: [w2587 w2593 w2597 w2602 w2607] -> w2568
                  tunnel: [w2587 w2593 w2597 w2602 w2606] -> w2567
                  tunnel: [w2587 w2593 0.0 ("NewVal") 0.0 ("NewVal") w2606] -> w2566
                  tunnel: [TRUE TRUE TRUE TRUE FALSE] -> w2570
                  tunnel: [TRUE TRUE FALSE FALSE FALSE] -> w2569
                  frame 0 {
                    # "Works as Instr1/2/3"
                    # "The three phase values are equal for (L-N)"
                    n1182 = Square Root(x=3.0) -> (sqrt(x)=w2589:dbl)
                    n1183 = Divide(x=w2588, y=w2589) -> (x/y=w2587:dbl)
                  }
                  frame 1, 2 {
                    # "Works as Instr1/2/3"
                    # "All three channels joined as a single output"
                  }
                  frame 5, 6 {
                    # "Works as Instr1/2 only"
                    # "Two channels joined as a Two-Phase output"
                    n1184 = Divide(x=w2599, y=2.0) -> (x/y=w2597:dbl)
                  }
                  frame 7, 8, 11, 12 {
                    # "Works as Instr1/2 only"
                    # "Two channels joined as a single output"
                  }
                  frame Default {
                    w2606 = 0.0 ("NewVal")
                    # "Works as Instr1 only"
                    # "Instr1 is alone and\nuses only one channel"
                  }
                }
                n1185 = case shown="True" w2569 {
                  tunnel: w2568 -> [_ w2576]
                  tunnel: w2567 -> [_ w2575]
                  tunnel: w2566 -> [_ w2574]
                  tunnel: w2564 -> [_ w2573]
                  frame False {
                  }
                  frame True {
                    n1186 = local read "Instr3"() -> (w2577:T2)
                    n1187 = Bundle By Name(cluster=w2577, "Phases.A-Volts (V)"=w2576, "Phases.B-Volts (V)"=w2575, "Phases.C-Volts (V)"=w2574, "Vout (V)"=w2573) -> (w2578:T2)
                    n1188 = local write "Instr3"(w2578) -> ()
                  }
                }
                n1189 = case shown="True" w2570 {
                  tunnel: w2568 -> [_ w2582]
                  tunnel: w2567 -> [_ w2581]
                  tunnel: w2566 -> [_ w2580]
                  tunnel: w2564 -> [_ w2579]
                  frame False {
                  }
                  frame True {
                    n1190 = local read "Instr2"() -> (w2584:T2)
                    n1191 = Bundle By Name(cluster=w2584, "Phases.A-Volts (V)"=w2582, "Phases.B-Volts (V)"=w2581, "Phases.C-Volts (V)"=w2580, "Vout (V)"=w2579) -> (w2583:T2)
                    n1192 = local write "Instr2"(w2583) -> ()
                  }
                }
                n1193 = local read "Instr1"() -> (w2571:T2)
                n1194 = Bundle By Name(cluster=w2571, "Vout (V)"=w2564, "Phases.A-Volts (V)"=w2568, "Phases.B-Volts (V)"=w2567, "Phases.C-Volts (V)"=w2566) -> (w2572:T2)
                n1195 = local write "Instr1"(w2572) -> ()
              }
            }
            n1196 = property on="Update" class="Bool (strict)"(error in=w2548) -> (error out=w2556:errorcluster, "Value"=w2544:bool)  [unwired: 1 in, 1 out]
            n1197 = property on="Update" class="Bool (strict)"(error in=w2556, "Val(Sgnl)"=w2544) -> (error out=w2547:errorcluster)  [unwired: 1 in, 1 out]
            n1198 = property on="btnSaveAs" class="Bool"(error in=w2547, "DisabledEnum"=w2558) -> (error out=w2560:errorcluster)  [unwired: 1 in, 1 out]
            n1199 = property on="btnSave" class="Bool"(error in=w2547, "DisabledEnum"=w2558) -> (error out=w2559:errorcluster)  [unwired: 1 in, 1 out]
            n1200 = Merge Errors(w2559, w2560) -> (w2557:errorcluster)
          }
          event Value Change {
            w2636 = T15."Enabled" ("Disabled")
            w2639 = FALSE ("StartMeas")
            # "There's no need to check for Mode because Instr2 can only appear in the interface to be operated by the user when it is working alone as a separate instrument."
            # "Instr2"
            # "Turn that indexed string into its actual numeric value."
            # "Get the present limits that the V Range control has, and the index of the present range selection."
            # "Update Device(s)Settings"
            # "Instr2 can only detect a Vout change when it's not being overriden by Instr1 and has its own instrument panel visible so that the user can operate its controls."
            n1201 = event-data() -> ("NewVal"=w2620:dbl)  [unwired: 1 in]
            n1202 = property on="Voltage (V)" class="Ring (strict)"(error in=w2627) -> (error out=w2632:errorcluster, "Strings []"=w2633:string[], "Value"=w2630:u16)  [unwired: 1 in, 1 out]
            n1203 = Index Array(array=w2633, index=w2630) -> (element=w2631:string)
            n1204 = Scan From String(format string="%f", input string=w2631, error in=w2632) -> (error out=w2623:errorcluster, output 1=w2621:dbl)  [unwired: 2 in, 2 out]
            n1205 = Merge Errors(w2627, w2623) -> (w2626:errorcluster)
            n1206 = Less?(x=w2621, y=w2620) -> (x < y?=w2628:bool)
            n1207 = case shown="True" w2628 {
              frame False {
                # "No voltage range adjustment needed. Vout falls within present range."
              }
              frame True {
                # "Increase range so that Vout can fit within it."
                n1208 = local read "Instr2"() -> (w2648:T2)
                n1209 = Bundle By Name(cluster=w2648, "Ranges.Voltage (V)"=u16 1) -> (w2647:T2)
                n1210 = local write "Instr2"(w2647) -> ()
              }
            }
            n1211 = flat-sequence {
              tunnel: w2626 -> [w2644]
              tunnel: [w2644] -> w2625
              tunnel: w2620 -> [w2641]
              frame #0 {
                w2645 = 0.0 ("NewVal")
                # "The frame is only to ensure that the cluster is updated before \"Update\" is called."
                n1212 = local read "Instr2"() -> (w2643:T2)
                n1213 = Bundle By Name(cluster=w2643, "Phases.C-Volts (V)"=w2645, "Phases.B-Volts (V)"=w2645, "Phases.A-Volts (V)"=w2641, "Vout (V)"=w2641) -> (w2642:T2)
                n1214 = local write "Instr2"(w2642) -> ()
              }
            }
            n1215 = property on="Update" class="Bool (strict)"(error in=w2625) -> (error out=w2634:errorcluster, "Value"=w2622:bool)  [unwired: 1 in, 1 out]
            n1216 = property on="Update" class="Bool (strict)"(error in=w2634, "Val(Sgnl)"=w2622) -> (error out=w2624:errorcluster)  [unwired: 1 in, 1 out]
            n1217 = property on="btnSaveAs" class="Bool"(error in=w2624, "DisabledEnum"=w2636) -> (error out=w2638:errorcluster)  [unwired: 1 in, 1 out]
            n1218 = property on="btnSave" class="Bool"(error in=w2624, "DisabledEnum"=w2636) -> (error out=w2637:errorcluster)  [unwired: 1 in, 1 out]
            n1219 = Merge Errors(w2637, w2638) -> (w2635:errorcluster)
          }
          event Value Change {
            w2665 = T15."Enabled" ("Disabled")
            w2668 = FALSE ("StartMeas")
            # "There's no need to check for Mode because Instr3 can only appear in the interface to be operated by the user when it is working alone as a separate instrument."
            # "Instr3"
            # "Turn that indexed string into its actual numeric value."
            # "Get the present limits that the V Range control has, and the index of the present range selection."
            # "Update Device(s)Settings"
            # "Instr3 can only detect a Vout change when it's not being overriden by Instr1 and has its own instrument panel visible so that the user can operate its controls."
            n1220 = event-data() -> ("NewVal"=w2649:dbl)  [unwired: 1 in]
            n1221 = property on="Voltage (V)" class="Ring (strict)"(error in=w2656) -> (error out=w2661:errorcluster, "Strings []"=w2662:string[], "Value"=w2659:u16)  [unwired: 1 in, 1 out]
            n1222 = Index Array(array=w2662, index=w2659) -> (element=w2660:string)
            n1223 = Scan From String(format string="%f", input string=w2660, error in=w2661) -> (error out=w2652:errorcluster, output 1=w2650:dbl)  [unwired: 2 in, 2 out]
            n1224 = Merge Errors(w2656, w2652) -> (w2655:errorcluster)
            n1225 = Less?(x=w2650, y=w2649) -> (x < y?=w2657:bool)
            n1226 = case shown="True" w2657 {
              frame False {
                # "No voltage range adjustment needed. Vout falls within present range."
              }
              frame True {
                # "Increase range so that Vout can fit within it."
                n1227 = local read "Instr3"() -> (w2677:T2)
                n1228 = Bundle By Name(cluster=w2677, "Ranges.Voltage (V)"=u16 1) -> (w2676:T2)
                n1229 = local write "Instr3"(w2676) -> ()
              }
            }
            n1230 = flat-sequence {
              tunnel: w2655 -> [w2673]
              tunnel: [w2673] -> w2654
              tunnel: w2649 -> [w2670]
              frame #0 {
                w2674 = 0.0 ("NewVal")
                # "The frame is only to ensure that the cluster is updated before \"Update\" is called."
                n1231 = local read "Instr3"() -> (w2672:T2)
                n1232 = Bundle By Name(cluster=w2672, "Phases.C-Volts (V)"=w2674, "Phases.B-Volts (V)"=w2674, "Phases.A-Volts (V)"=w2670, "Vout (V)"=w2670) -> (w2671:T2)
                n1233 = local write "Instr3"(w2671) -> ()
              }
            }
            n1234 = property on="Update" class="Bool (strict)"(error in=w2654) -> (error out=w2663:errorcluster, "Value"=w2651:bool)  [unwired: 1 in, 1 out]
            n1235 = property on="Update" class="Bool (strict)"(error in=w2663, "Val(Sgnl)"=w2651) -> (error out=w2653:errorcluster)  [unwired: 1 in, 1 out]
            n1236 = property on="btnSaveAs" class="Bool"(error in=w2653, "DisabledEnum"=w2665) -> (error out=w2667:errorcluster)  [unwired: 1 in, 1 out]
            n1237 = property on="btnSave" class="Bool"(error in=w2653, "DisabledEnum"=w2665) -> (error out=w2666:errorcluster)  [unwired: 1 in, 1 out]
            n1238 = Merge Errors(w2666, w2667) -> (w2664:errorcluster)
          }
          event Value Change {
            w2689 = T15."Enabled" ("Disabled")
            w2691 = FALSE ("StartMeas")
            # "Get all the present phase voltages in Instr1"
            # "Update Device(s)Settings"
            # "Only Instr1 can be configured to be multiphase. Therefore, it's the only instrument which provides user access to modify any phase voltages individually.\nThere's no need to check for \"Instr2.PhasesABC\" changes nor \"Instr3. PhasesABC\" changes, because those cases cannot be generated by the user."
            # "Instr1 is the only one that can change phase voltage values. Verify that any new phase voltage value is within range, and if it's not, force it to be."
            n1239 = event-data() -> ("CtlRef"=w2692:refnum<vi>)  [unwired: 1 in, 2 out]
            n1240 = local read "Instr1"() -> (w2688:T2)
            n1241 = Unbundle By Name(w2688) -> ("Phases.A-Volts (V)"=w2686:dbl, "Phases.B-Volts (V)"=w2687:dbl, "Phases.C-Volts (V)"=w2685:dbl)
            n1242 = local read "Mode"() -> (w2693:T8)
            n1243 = case shown="0" w2693 {
              tunnel: w2692 -> [_ w2710 w2746]
              tunnel: [w2695 w2704 w2741] -> w2678
              tunnel: w2687 -> [_ w2705 w2744]
              tunnel: w2686 -> [_ w2706 w2742]
              tunnel: w2685 -> [_ _ w2743]
              tunnel: w2684 -> [w2695 w2709 w2745]
              frame Default {
                # "The rest of the modes have no phases, so there's no need to adjust anything."
              }
              frame 5, 6 {
                # "Set the voltage level range to an adequate value depending if the total is within range or if it could have exceeded it."
                # "Two-Phase Modes"
                n1244 = property class="DigNum (strict)"(reference=w2710, error in=w2709) -> (reference out=w2707:refnum<vi>, error out=w2708:errorcluster, "Label.Text"=w2713:string)
                n1245 = Add(x=w2706, y=w2705) -> (x+y=w2715:dbl)
                n1246 = Greater?(x=w2715, y=500.0) -> (0:w2712:bool)
                n1247 = Close Reference(reference=w2707, error in (no error)=w2708) -> (error out=w2704:errorcluster)
                n1248 = case shown="True" w2712 {
                  tunnel: w2713 -> [_ w2732]
                  tunnel: "A-Volts (V)" -> [_ w2731]
                  tunnel: w2706 -> [w2718 w2729]
                  tunnel: w2705 -> [w2717 w2728]
                  tunnel: [w2718 w2727] -> w2696
                  tunnel: [w2717 w2726] -> w2697
                  tunnel: [w2719 u16 1 ("f")] -> w2698
                  tunnel: [w2716 500.0] -> w2699
                  frame False {
                    # "The combined value of both phases generates a value of Vout within valid limits."
                    # "Depending on the combined result of the phase values, adjust to the adequate voltage range level"
                    n1249 = Add(x=w2718, y=w2717) -> (x+y=w2716:dbl)
                    n1250 = Greater?(x=w2716, y=350.0) -> (0:w2722:bool)
                    n1251 = Select(t=u16 1, s=w2722, f=u16 0) -> (s? t:f=w2719:u16)
                  }
                  frame True, Default {
                    n1252 = Equal?(x=w2732, y=w2731) -> (x = y?=w2730:bool)
                    n1253 = case shown="True" w2730 {
                      tunnel: w2729 -> [w2735 w2738]
                      tunnel: w2728 -> [w2733 w2739]
                      tunnel: [w2734 w2738] -> w2727
                      tunnel: [w2733 w2737] -> w2726
                      frame True {
                        # "Adjust it so that the sum of both phases doesn't exceed 500V"
                        # "If Phase-A value exceeded max Two-Phase V range"
                        n1254 = Subtract(x=500.0 ("y"), y=w2735) -> (x-y=w2734:dbl)
                      }
                      frame False {
                        # "Adjust it so that the sum of both phases doesn't exceed 500V"
                        # "If Phase-B value exceeded max Two-Phase V range"
                        n1255 = Subtract(x=500.0 ("y"), y=w2739) -> (x-y=w2737:dbl)
                      }
                    }
                  }
                }
                n1256 = local read "Instr1"() -> (w2703:T2)
                n1257 = Bundle By Name(cluster=w2703, "Vout (V)"=w2699, "Ranges.Voltage (V)"=w2698, "Phases.A-Volts (V)"=w2696, "Phases.B-Volts (V)"=w2697) -> (w2702:T2)
                n1258 = local write "Instr1"(w2702) -> ()
                n1259 = local read "Instr2"() -> (w2700:T2)
                n1260 = Bundle By Name(cluster=w2700, "Vout (V)"=w2699, "Ranges.Voltage (V)"=w2698, "Phases.A-Volts (V)"=w2696, "Phases.B-Volts (V)"=w2697) -> (w2701:T2)
                n1261 = local write "Instr2"(w2701) -> ()
              }
              frame 0 {
                # "Do the phases math to get the present value of Vout"
                # "Check if the contribution all  phase voltages exceeds the 606V three phase maximum."
                # "Three-Phase Mode will check against the possibility of exceeding 606V, and which adequate voltage range level to use."
                n1262 = property class="DigNum (strict)"(reference=w2746, error in=w2745) -> (error out=w2741:errorcluster, "Label.Text"=w2754:string)  [unwired: 1 out]
                n1263 = Compound Arithmetic op=ADD(w2742, w2744, w2743) -> (w2749:dbl)
                n1264 = Square Root(x=3.0) -> (sqrt(x)=w2751:dbl)
                n1265 = Divide(x=w2749, y=3.0) -> (x/y=w2748:dbl)
                n1266 = Multiply(x=w2751, y=w2748) -> (x*y=w2750:dbl)
                n1267 = Greater?(x=w2750, y=606.0) -> (0:w2753:bool)
                n1268 = case shown="True" w2753 {
                  tunnel: w2754 -> [_ w2789]
                  tunnel: w2750 -> [w2760 _]
                  tunnel: w2744 -> [w2757 w2788]
                  tunnel: w2743 -> [w2756 w2787]
                  tunnel: w2742 -> [w2758 w2782]
                  frame False {
                    # "If the total value of all phases combined did not exceed the maximum 606V of the three phase Mode, there's no need to adjust their values. Check instead which is the correct voltage range that can contain the result. Adjust the range to be either 303V or 606V depending on the magnitude of the new total."
                    n1269 = Greater?(x=w2760, y=303.0) -> (0:w2769:bool)
                    n1270 = Select(t=u16 1, s=w2769, f=u16 0) -> (s? t:f=w2759:u16)
                    n1271 = local read "Instr1"() -> (w2765:T2)
                    n1272 = Bundle By Name(cluster=w2765, "Vout (V)"=w2760, "Ranges.Voltage (V)"=w2759, "Phases.A-Volts (V)"=w2758, "Phases.B-Volts (V)"=w2757, "Phases.C-Volts (V)"=w2756) -> (w2766:T2)
                    n1273 = local write "Instr1"(w2766) -> ()
                    n1274 = local read "Instr2"() -> (w2764:T2)
                    n1275 = Bundle By Name(cluster=w2764, "Vout (V)"=w2760, "Ranges.Voltage (V)"=w2759, "Phases.A-Volts (V)"=w2758, "Phases.B-Volts (V)"=w2757, "Phases.C-Volts (V)"=w2756) -> (w2763:T2)
                    n1276 = local write "Instr2"(w2763) -> ()
                    n1277 = local read "Instr3"() -> (w2761:T2)
                    n1278 = Bundle By Name(cluster=w2761, "Vout (V)"=w2760, "Ranges.Voltage (V)"=w2759, "Phases.A-Volts (V)"=w2758, "Phases.B-Volts (V)"=w2757, "Phases.C-Volts (V)"=w2756) -> (w2762:T2)
                    n1279 = local write "Instr3"(w2762) -> ()
                  }
                  frame True, Default {
                    # "Set the Instr1 V range to the 606V choice because the new value would have exceeded it. Due to that, Vout has to be set to the 606V maximum too."
                    n1280 = case shown="\"A-Volts (V)\", Default" w2789 {
                      tunnel: w2788 -> [w2791 _ w2809]
                      tunnel: w2787 -> [w2790 w2799 _]
                      tunnel: [w2792 w2800 w2808] -> w2771
                      tunnel: w2782 -> [_ w2800 w2808]
                      tunnel: [w2791 w2801 w2809] -> w2772
                      tunnel: [w2790 w2799 w2810] -> w2773
                      frame "A-Volts (V)", Default {
                        w2794 = 3.0 ("y")
                        # "Adjust Phase A volts so that the contribution of all phases adds up to 606V"
                        n1281 = Compound Arithmetic op=ADD(w2791, w2790) -> (w2798:dbl)
                        n1282 = Multiply(x=606.0 ("y"), y=w2794) -> (x*y=w2795:dbl)
                        n1283 = Square Root(x=w2794) -> (sqrt(x)=w2796:dbl)
                        n1284 = Divide(x=w2795, y=w2796) -> (x/y=w2797:dbl)
                        n1285 = Subtract(x=w2797, y=w2798) -> (x-y=w2792:dbl)
                      }
                      frame "B-Volts (V)" {
                        w2804 = 3.0 ("y")
                        # "Adjust Phase B volts so that the contribution of all phases adds up to 606V"
                        n1286 = Compound Arithmetic op=ADD(w2800, w2799) -> (w2802:dbl)
                        n1287 = Multiply(x=606.0 ("y"), y=w2804) -> (x*y=w2806:dbl)
                        n1288 = Square Root(x=w2804) -> (sqrt(x)=w2805:dbl)
                        n1289 = Divide(x=w2806, y=w2805) -> (x/y=w2803:dbl)
                        n1290 = Subtract(x=w2803, y=w2802) -> (x-y=w2801:dbl)
                      }
                      frame "C-Volts (V)" {
                        w2812 = 3.0 ("y")
                        # "Adjust Phase C volts so that the contribution of all phases adds up to 606V"
                        n1291 = Compound Arithmetic op=ADD(w2808, w2809) -> (w2816:dbl)
                        n1292 = Multiply(x=606.0 ("y"), y=w2812) -> (x*y=w2813:dbl)
                        n1293 = Square Root(x=w2812) -> (sqrt(x)=w2814:dbl)
                        n1294 = Divide(x=w2813, y=w2814) -> (x/y=w2815:dbl)
                        n1295 = Subtract(x=w2815, y=w2816) -> (x-y=w2810:dbl)
                      }
                    }
                    n1296 = local read "Instr1"() -> (w2786:T2)
                    n1297 = Bundle By Name(cluster=w2786, "Vout (V)"=606.0 ("y"), "Ranges.Voltage (V)"=u16 1 ("Value"), "Phases.A-Volts (V)"=w2771, "Phases.B-Volts (V)"=w2772, "Phases.C-Volts (V)"=w2773) -> (w2785:T2)
                    n1298 = local write "Instr1"(w2785) -> ()
                    n1299 = local read "Instr2"() -> (w2778:T2)
                    n1300 = Bundle By Name(cluster=w2778, "Vout (V)"=606.0 ("y"), "Ranges.Voltage (V)"=u16 1 ("Value"), "Phases.A-Volts (V)"=w2771, "Phases.B-Volts (V)"=w2772, "Phases.C-Volts (V)"=w2773) -> (w2779:T2)
                    n1301 = local write "Instr2"(w2779) -> ()
                    n1302 = local read "Instr3"() -> (w2777:T2)
                    n1303 = Bundle By Name(cluster=w2777, "Vout (V)"=606.0 ("y"), "Ranges.Voltage (V)"=u16 1 ("Value"), "Phases.A-Volts (V)"=w2771, "Phases.B-Volts (V)"=w2772, "Phases.C-Volts (V)"=w2773) -> (w2776:T2)
                    n1304 = local write "Instr3"(w2776) -> ()
                  }
                }
              }
            }
            n1305 = property on="Update" class="Bool (strict)"(error in=w2678) -> (error out=w2690:errorcluster, "Value"=w2683:bool)  [unwired: 1 in, 1 out]
            n1306 = property on="btnSaveAs" class="Bool"(error in=w2678, "DisabledEnum"=w2689) -> (error out=w2680:errorcluster)  [unwired: 1 in, 1 out]
            n1307 = property on="btnSave" class="Bool"(error in=w2678, "DisabledEnum"=w2689) -> (error out=w2681:errorcluster)  [unwired: 1 in, 1 out]
            n1308 = property on="Update" class="Bool (strict)"(error in=w2690, "Val(Sgnl)"=w2683) -> (error out=w2679:errorcluster)  [unwired: 1 in, 1 out]
            n1309 = Merge Errors(w2681, w2680, w2679) -> (w2682:errorcluster)
          }
          event Value Change {
            w2824 = T15."Enabled" ("Disabled")
            w2825 = FALSE ("StartMeas")
            # "No need to \"Update\" here because values are passed directly to Device(s)Settings  in the case select structure."
            # "Get all the present phase angles in Instr1"
            # "Only Instr1 can be configured to be multiphase. Therefore, it's the only instrument which provides user access to modify any phase angles individually. There's no need to check for Instr2 or Instr3 for these controls."
            # "Instr1 is the only one that can change phase angle values. Angles should be coerced already only as integers between 0 and 359, and only available for three-phase and two-phase cases."
            n1310 = event-data() -> ()  [unwired: 1 in, 3 out]
            n1311 = local read "Instr1"() -> (w2818:T2)
            n1312 = Unbundle By Name(w2818) -> ("Phases.B-Angle (Deg)"=w2821:i32, "Phases.C-Angle (Deg)"=w2822:i32)
            n1313 = local read "Mode"() -> (w2826:T8)
            n1314 = case shown="0" w2826 {
              tunnel: [w2828 w2833 w2838] -> w2817
              tunnel: w2822 -> [w2829 _ _]
              tunnel: w2821 -> [w2831 w2836 _]
              tunnel: w2820 -> [w2828 w2833 w2838]
              frame 0 {
                # "Three-phase mode is the only one that uses both angles B and C."
                n1315 = local read "Device(s)Settings"() -> (w2832:T1)
                n1316 = Bundle By Name(cluster=w2832, "Instr1.Phases.B-Angle (Deg)"=w2831, "Instr2.Phases.B-Angle (Deg)"=w2831, "Instr3.Phases.B-Angle (Deg)"=w2831, "Instr1.Phases.C-Angle (Deg)"=w2829, "Instr2.Phases.C-Angle (Deg)"=w2829, "Instr3.Phases.C-Angle (Deg)"=w2829) -> (w2830:T1)
                n1317 = local write "Device(s)Settings"(w2830) -> ()
              }
              frame 5, 6 {
                w2834 = 0 ("Instr2.Phases.C-Angle (Deg)")
                # "Two-phse only uses Instr1 and Instr2 together for the B angle. Everything else has to be 0."
                # "Two-phase mode is the only one that uses only angles B."
                n1318 = local read "Device(s)Settings"() -> (w2837:T1)
                n1319 = Bundle By Name(cluster=w2837, "Instr1.Phases.B-Angle (Deg)"=w2836, "Instr2.Phases.B-Angle (Deg)"=w2836, "Instr3.Phases.B-Angle (Deg)"=w2834, "Instr1.Phases.C-Angle (Deg)"=w2834, "Instr2.Phases.C-Angle (Deg)"=w2834, "Instr3.Phases.C-Angle (Deg)"=w2834) -> (w2835:T1)
                n1320 = local write "Device(s)Settings"(w2835) -> ()
              }
              frame Default {
                w2839 = 0 ("Instr2.Phases.C-Angle (Deg)")
                # "Any other Modes doesn't use phase angles, set them to 0 in all instruments."
                n1321 = local read "Device(s)Settings"() -> (w2841:T1)
                n1322 = Bundle By Name(cluster=w2841, "Instr1.Phases.B-Angle (Deg)"=w2839, "Instr2.Phases.B-Angle (Deg)"=w2839, "Instr3.Phases.B-Angle (Deg)"=w2839, "Instr1.Phases.C-Angle (Deg)"=w2839, "Instr2.Phases.C-Angle (Deg)"=w2839, "Instr3.Phases.C-Angle (Deg)"=w2839) -> (w2840:T1)
                n1323 = local write "Device(s)Settings"(w2840) -> ()
              }
            }
            n1324 = property on="btnSave" class="Bool"(error in=w2817, "DisabledEnum"=w2824) -> (error out=w2823:errorcluster)  [unwired: 1 in, 1 out]
            n1325 = property on="btnSaveAs" class="Bool"(error in=w2823, "DisabledEnum"=w2824) -> (error out=w2819:errorcluster)  [unwired: 1 in, 1 out]
          }
          event Value Change {
            w2850 = T15."Enabled" ("Disabled")
            w2851 = FALSE ("StartMeas")
            # "No need to \"Update\" here because values are passed directly to Device(s)Settings in the case select structure."
            # "Get all the present \"Change at\" values in Instr1"
            # "Since Instr1 may override Instr2 and Instr3 in some modes, and it can be three-phase, two-phase or one phase, evaluate what to do depending on Mode."
            n1326 = event-data() -> ()  [unwired: 1 in, 3 out]
            n1327 = local read "Instr1"() -> (w2844:T2)
            n1328 = Unbundle By Name(w2844) -> ("Phases.A-Change at..."=w2847:i32, "Phases.B-Change at..."=w2848:i32, "Phases.C-Change at..."=w2842:i32)
            n1329 = local read "Mode"() -> (w2852:T8)
            n1330 = case shown="0" w2852 {
              tunnel: [w2855 w2862 w2868 w2873 w2878 w2881] -> w2843
              tunnel: w2848 -> [w2856 w2861 _ _ _ _]
              tunnel: w2847 -> [w2858 w2864 w2867 w2872 w2877 _]
              tunnel: w2846 -> [w2855 w2862 w2868 w2873 w2878 w2881]
              tunnel: w2842 -> [w2854 _ _ _ _ _]
              frame 0 {
                # "In three-phase mode all values are used, and affect Instr2 and Instr3 too."
                n1331 = local read "Device(s)Settings"() -> (w2859:T1)
                n1332 = Bundle By Name(cluster=w2859, "Instr1.Phases.A-Change at..."=w2858, "Instr2.Phases.A-Change at..."=w2858, "Instr3.Phases.A-Change at..."=w2858, "Instr1.Phases.B-Change at..."=w2856, "Instr2.Phases.B-Change at..."=w2856, "Instr3.Phases.B-Change at..."=w2856, "Instr1.Phases.C-Change at..."=w2854, "Instr2.Phases.C-Change at..."=w2854, "Instr3.Phases.C-Change at..."=w2854) -> (w2857:T1)
                n1333 = local write "Device(s)Settings"(w2857) -> ()
              }
              frame 5, 6 {
                w2860 = 0 ("Instr1.Phases.C-Change at...")
                # "In two-phase mode \"Chage at\" C is not used. Instr1 and Instr2 are linked."
                n1334 = local read "Device(s)Settings"() -> (w2865:T1)
                n1335 = Bundle By Name(cluster=w2865, "Instr1.Phases.A-Change at..."=w2864, "Instr2.Phases.A-Change at..."=w2864, "Instr1.Phases.B-Change at..."=w2861, "Instr2.Phases.B-Change at..."=w2861, "Instr1.Phases.C-Change at..."=w2860, "Instr2.Phases.C-Change at..."=w2860) -> (w2863:T1)
                n1336 = local write "Device(s)Settings"(w2863) -> ()
              }
              frame 1 {
                w2866 = 0 ("Instr1.Phases.C-Change at...")
                # "Instr1, Instr2 and Instr3 are a single combined one-phase AC instrument."
                n1337 = local read "Device(s)Settings"() -> (w2870:T1)
                n1338 = Bundle By Name(cluster=w2870, "Instr1.Phases.A-Change at..."=w2867, "Instr2.Phases.A-Change at..."=w2867, "Instr3.Phases.A-Change at..."=w2867, "Instr1.Phases.B-Change at..."=w2866, "Instr2.Phases.B-Change at..."=w2866, "Instr3.Phases.B-Change at..."=w2866, "Instr1.Phases.C-Change at..."=w2866, "Instr2.Phases.C-Change at..."=w2866, "Instr3.Phases.C-Change at..."=w2866) -> (w2869:T1)
                n1339 = local write "Device(s)Settings"(w2869) -> ()
              }
              frame 7, 8 {
                w2871 = 0 ("Instr1.Phases.C-Change at...")
                # "Instr1 and Instr2 are a single combined one-phase AC instrument."
                n1340 = local read "Device(s)Settings"() -> (w2875:T1)
                n1341 = Bundle By Name(cluster=w2875, "Instr1.Phases.A-Change at..."=w2872, "Instr2.Phases.A-Change at..."=w2872, "Instr1.Phases.B-Change at..."=w2871, "Instr2.Phases.B-Change at..."=w2871, "Instr1.Phases.C-Change at..."=w2871, "Instr2.Phases.C-Change at..."=w2871) -> (w2874:T1)
                n1342 = local write "Device(s)Settings"(w2874) -> ()
              }
              frame 3, 9, 10, 13 {
                w2876 = 0 ("Instr1.Phases.C-Change at...")
                # "Instr1 is a single one-phase AC instrument."
                n1343 = local read "Device(s)Settings"() -> (w2880:T1)
                n1344 = Bundle By Name(cluster=w2880, "Instr1.Phases.A-Change at..."=w2877, "Instr1.Phases.B-Change at..."=w2876, "Instr1.Phases.C-Change at..."=w2876) -> (w2879:T1)
                n1345 = local write "Device(s)Settings"(w2879) -> ()
              }
              frame Default {
                # "Don't update any settings, they should all be set to 0 by default in all instrumenst and modes when the event \"Mode change\" occurs."
                # "In all other modes Instr1 is DC and \"Change at\" cannot generate a change event."
              }
            }
            n1346 = property on="btnSave" class="Bool"(error in=w2843, "DisabledEnum"=w2850) -> (error out=w2849:errorcluster)  [unwired: 1 in, 1 out]
            n1347 = property on="btnSaveAs" class="Bool"(error in=w2849, "DisabledEnum"=w2850) -> (error out=w2845:errorcluster)  [unwired: 1 in, 1 out]
          }
          event Value Change {
            w2892 = T15."Enabled" ("Disabled")
            w2893 = FALSE ("StartMeas")
            # "Voltage slew always matters.\nCurrent and Power only matter for DC slews.\nFrequency and Phase only matter for AC slews."
            # "No need to \"Update\" here because values are passed directly to Device(s)Settings in the case select structure."
            # "Since Instr1 may override Instr2 and Instr3 in some modes, and AC and DC don't have the same slews available to the user, evaluate what to do with Slew changes depending on Mode."
            n1348 = event-data() -> ()  [unwired: 1 in, 1 out]
            n1349 = local read "Instr1"() -> (w2889:T2)
            n1350 = Unbundle By Name(w2889) -> ("Slew Rates.Voltage (V/s)"=w2888:dbl, "Slew Rates.Current (A/s)"=w2885:dbl, "Slew Rates.Power (W/s)"=w2884:dbl, "Slew Rates.Frequency (Hz/s)"=w2887:dbl, "Slew Rates.Phase Angle (Deg/s)"=w2886:dbl)
            n1351 = local read "Mode"() -> (w2894:T8)
            n1352 = case shown="0, 1, Default" w2894 {
              tunnel: w2888 -> [w2899 w2905 w2911 w2917 w2923 w2929]
              tunnel: w2887 -> [w2898 w2903 w2909 _ w2921 w2928]
              tunnel: w2886 -> [w2897 _ w2910 _ w2922 _]
              tunnel: w2885 -> [_ w2904 _ w2916 _ w2927]
              tunnel: w2884 -> [_ _ _ w2915 _ _]
              tunnel: [w2896 w2902 w2908 w2914 w2920 w2926] -> w2882
              tunnel: w2883 -> [w2896 w2902 w2908 w2914 w2920 w2926]
              frame 0, 1, Default {
                # "Instr1 is AC and overrides Instr2 and Instr3"
                n1353 = local read "Device(s)Settings"() -> (w2901:T1)
                n1354 = Bundle By Name(cluster=w2901, "Instr1.Slew Rates.Voltage (V/s)"=w2899, "Instr2.Slew Rates.Voltage (V/s)"=w2899, "Instr3.Slew Rates.Voltage (V/s)"=w2899, "Instr1.Slew Rates.Frequency (Hz/s)"=w2898, "Instr2.Slew Rates.Frequency (Hz/s)"=w2898, "Instr3.Slew Rates.Frequency (Hz/s)"=w2898, "Instr1.Slew Rates.Phase Angle (Deg/s)"=w2897, "Instr2.Slew Rates.Phase Angle (Deg/s)"=w2897, "Instr3.Slew Rates.Phase Angle (Deg/s)"=w2897) -> (w2900:T1)
                n1355 = local write "Device(s)Settings"(w2900) -> ()
              }
              frame 2 {
                # "Instr1 is DC and overrides Instr2 and Instr3"
                n1356 = local read "Device(s)Settings"() -> (w2907:T1)
                n1357 = Bundle By Name(cluster=w2907, "Instr1.Slew Rates.Voltage (V/s)"=w2905, "Instr2.Slew Rates.Voltage (V/s)"=w2905, "Instr3.Slew Rates.Voltage (V/s)"=w2905, "Instr1.Slew Rates.Current (A/s)"=w2904, "Instr2.Slew Rates.Current (A/s)"=w2904, "Instr3.Slew Rates.Current (A/s)"=w2904, "Instr1.Slew Rates.Power (W/s)"=w2903, "Instr2.Slew Rates.Power (W/s)"=w2903, "Instr3.Slew Rates.Power (W/s)"=w2903) -> (w2906:T1)
                n1358 = local write "Device(s)Settings"(w2906) -> ()
              }
              frame 3, 9, 10, 13 {
                # "Instr1 is AC working as a single instrument"
                n1359 = local read "Device(s)Settings"() -> (w2913:T1)
                n1360 = Bundle By Name(cluster=w2913, "Instr1.Slew Rates.Voltage (V/s)"=w2911, "Instr1.Slew Rates.Frequency (Hz/s)"=w2909, "Instr1.Slew Rates.Phase Angle (Deg/s)"=w2910) -> (w2912:T1)
                n1361 = local write "Device(s)Settings"(w2912) -> ()
              }
              frame 4, 14, 15 {
                # "Instr1 is DC working as a single instrument"
                n1362 = local read "Device(s)Settings"() -> (w2919:T1)
                n1363 = Bundle By Name(cluster=w2919, "Instr1.Slew Rates.Voltage (V/s)"=w2917, "Instr1.Slew Rates.Current (A/s)"=w2916, "Instr1.Slew Rates.Power (W/s)"=w2915) -> (w2918:T1)
                n1364 = local write "Device(s)Settings"(w2918) -> ()
              }
              frame 5..8 {
                # "Instr1 is AC and overrides Instr2 only"
                n1365 = local read "Device(s)Settings"() -> (w2925:T1)
                n1366 = Bundle By Name(cluster=w2925, "Instr1.Slew Rates.Voltage (V/s)"=w2923, "Instr2.Slew Rates.Voltage (V/s)"=w2923, "Instr1.Slew Rates.Frequency (Hz/s)"=w2921, "Instr2.Slew Rates.Frequency (Hz/s)"=w2921, "Instr1.Slew Rates.Phase Angle (Deg/s)"=w2922, "Instr2.Slew Rates.Phase Angle (Deg/s)"=w2922) -> (w2924:T1)
                n1367 = local write "Device(s)Settings"(w2924) -> ()
              }
              frame 11, 12 {
                # "Instr1 is DC and overrides Instr2 only"
                n1368 = local read "Device(s)Settings"() -> (w2931:T1)
                n1369 = Bundle By Name(cluster=w2931, "Instr1.Slew Rates.Voltage (V/s)"=w2929, "Instr2.Slew Rates.Voltage (V/s)"=w2929, "Instr1.Slew Rates.Current (A/s)"=w2927, "Instr2.Slew Rates.Current (A/s)"=w2927, "Instr1.Slew Rates.Power (W/s)"=w2928, "Instr2.Slew Rates.Power (W/s)"=w2928) -> (w2930:T1)
                n1370 = local write "Device(s)Settings"(w2930) -> ()
              }
            }
            n1371 = property on="btnSave" class="Bool"(error in=w2882, "DisabledEnum"=w2892) -> (error out=w2891:errorcluster)  [unwired: 1 in, 1 out]
            n1372 = property on="btnSaveAs" class="Bool"(error in=w2891, "DisabledEnum"=w2892) -> (error out=w2890:errorcluster)  [unwired: 1 in, 1 out]
          }
          event Value Change {
            w2942 = T15."Enabled" ("Disabled")
            w2943 = FALSE ("StartMeas")
            # "Voltage slew always matters.\nCurrent and Power only matter for DC slews.\nFrequency and Phase only matter for AC slews."
            # "No need to \"Update\" here because values are passed directly to Device(s)Settings in the case select structure."
            # "Instr2 can be configured by the user as  a single instrument only in some modes, and AC and DC don't have the same slews available to the user, evaluate what to do with Slew changes depending on Mode."
            n1373 = event-data() -> ()  [unwired: 1 in, 1 out]
            n1374 = local read "Instr2"() -> (w2939:T2)
            n1375 = Unbundle By Name(w2939) -> ("Slew Rates.Voltage (V/s)"=w2938:dbl, "Slew Rates.Current (A/s)"=w2935:dbl, "Slew Rates.Power (W/s)"=w2934:dbl, "Slew Rates.Frequency (Hz/s)"=w2937:dbl, "Slew Rates.Phase Angle (Deg/s)"=w2936:dbl)
            n1376 = local read "Mode"() -> (w2944:T8)
            n1377 = case shown="3, 9, 15, Default" w2944 {
              tunnel: w2938 -> [w2949 w2955]
              tunnel: w2937 -> [w2947 _]
              tunnel: w2936 -> [w2948 _]
              tunnel: w2935 -> [_ w2954]
              tunnel: w2934 -> [_ w2953]
              tunnel: [w2946 w2952] -> w2932
              tunnel: w2933 -> [w2946 w2952]
              frame 3, 9, 15, Default {
                # "Instr2 is AC working as a single instrument"
                n1378 = local read "Device(s)Settings"() -> (w2951:T1)
                n1379 = Bundle By Name(cluster=w2951, "Instr2.Slew Rates.Voltage (V/s)"=w2949, "Instr2.Slew Rates.Frequency (Hz/s)"=w2947, "Instr2.Slew Rates.Phase Angle (Deg/s)"=w2948) -> (w2950:T1)
                n1380 = local write "Device(s)Settings"(w2950) -> ()
              }
              frame 4, 10, 13 {
                # "Instr2 is DC working as a single instrument"
                n1381 = local read "Device(s)Settings"() -> (w2957:T1)
                n1382 = Bundle By Name(cluster=w2957, "Instr2.Slew Rates.Voltage (V/s)"=w2955, "Instr2.Slew Rates.Current (A/s)"=w2954, "Instr2.Slew Rates.Power (W/s)"=w2953) -> (w2956:T1)
                n1383 = local write "Device(s)Settings"(w2956) -> ()
              }
            }
            n1384 = property on="btnSave" class="Bool"(error in=w2932, "DisabledEnum"=w2942) -> (error out=w2941:errorcluster)  [unwired: 1 in, 1 out]
            n1385 = property on="btnSaveAs" class="Bool"(error in=w2941, "DisabledEnum"=w2942) -> (error out=w2940:errorcluster)  [unwired: 1 in, 1 out]
          }
          event Value Change {
            w2968 = T15."Enabled" ("Disabled")
            w2969 = FALSE ("StartMeas")
            # "Voltage slew always matters.\nCurrent and Power only matter for DC slews.\nFrequency and Phase only matter for AC slews."
            # "No need to \"Update\" here because values are passed directly to Device(s)Settings in the case select structure."
            # "Instr3 can be configured by the user as  a single instrument only in some modes, and AC and DC don't have the same slews available to the user, evaluate what to do with Slew changes depending on Mode."
            n1386 = event-data() -> ()  [unwired: 1 in, 1 out]
            n1387 = local read "Instr3"() -> (w2965:T2)
            n1388 = Unbundle By Name(w2965) -> ("Slew Rates.Voltage (V/s)"=w2964:dbl, "Slew Rates.Current (A/s)"=w2961:dbl, "Slew Rates.Power (W/s)"=w2960:dbl, "Slew Rates.Frequency (Hz/s)"=w2963:dbl, "Slew Rates.Phase Angle (Deg/s)"=w2962:dbl)
            n1389 = local read "Mode"() -> (w2970:T8)
            n1390 = case shown="4, 6, 8..10, 12, 15" w2970 {
              tunnel: w2964 -> [w2975 w2981]
              tunnel: w2963 -> [w2973 _]
              tunnel: w2962 -> [w2974 _]
              tunnel: w2961 -> [_ w2980]
              tunnel: w2960 -> [_ w2979]
              tunnel: [w2972 w2978] -> w2958
              tunnel: w2959 -> [w2972 w2978]
              frame 3, 5, 7, 11, 13, 14, Default {
                # "Instr3 is AC working as a single instrument"
                n1391 = local read "Device(s)Settings"() -> (w2977:T1)
                n1392 = Bundle By Name(cluster=w2977, "Instr3.Slew Rates.Voltage (V/s)"=w2975, "Instr3.Slew Rates.Frequency (Hz/s)"=w2973, "Instr3.Slew Rates.Phase Angle (Deg/s)"=w2974) -> (w2976:T1)
                n1393 = local write "Device(s)Settings"(w2976) -> ()
              }
              frame 4, 6, 8..10, 12, 15 {
                # "Instr3 is DC working as a single instrument"
                n1394 = local read "Device(s)Settings"() -> (w2983:T1)
                n1395 = Bundle By Name(cluster=w2983, "Instr3.Slew Rates.Voltage (V/s)"=w2981, "Instr3.Slew Rates.Current (A/s)"=w2980, "Instr3.Slew Rates.Power (W/s)"=w2979) -> (w2982:T1)
                n1396 = local write "Device(s)Settings"(w2982) -> ()
              }
            }
            n1397 = property on="btnSave" class="Bool"(error in=w2958, "DisabledEnum"=w2968) -> (error out=w2967:errorcluster)  [unwired: 1 in, 1 out]
            n1398 = property on="btnSaveAs" class="Bool"(error in=w2967, "DisabledEnum"=w2968) -> (error out=w2966:errorcluster)  [unwired: 1 in, 1 out]
          }
          event Value Change {
            w2990 = T15."Enabled" ("Disabled")
            w2991 = FALSE ("StartMeas")
            # "No need to \"Update\" here because values are passed directly to Device(s)Settings in the case select structure."
            # "Get all the present \"Change at\" values in Instr2"
            # "Instr2 it's only available as a stand-alone instrument in very few modes, and can only be a single channel instrument, so the call will only affect \"Change at\" A."
            n1399 = event-data() -> ()  [unwired: 1 in, 3 out]
            n1400 = local read "Instr2"() -> (w2985:T2)
            n1401 = Unbundle By Name(w2985) -> ("Phases.A-Change at..."=w2988:i32)
            n1402 = local read "Mode"() -> (w2992:T8)
            n1403 = case shown="3, 9, 14, 15" w2992 {
              tunnel: [w2995 w2998] -> w2984
              tunnel: w2988 -> [_ _]
              tunnel: w2987 -> [w2995 w2998]
              frame 3, 9, 14, 15 {
                w2994 = 0 ("Instr1.Phases.C-Change at...")
                # "The only modes when Instr2 is an avilable single one-phase AC instrument."
                n1404 = local read "Device(s)Settings"() -> (w2997:T1)
                n1405 = Bundle By Name(cluster=w2997, "Instr2.Phases.A-Change at..."=w2994, "Instr2.Phases.B-Change at..."=w2994, "Instr2.Phases.C-Change at..."=w2994) -> (w2996:T1)
                n1406 = local write "Device(s)Settings"(w2996) -> ()
              }
              frame Default {
                # "Don't update any settings, they should all be set to 0 by default in all instrumenst and modes when the event \"Mode change\" occurs."
                # "Instr2 is either DC or doesn't exist as a separate instrument."
              }
            }
            n1407 = property on="btnSave" class="Bool"(error in=w2984, "DisabledEnum"=w2990) -> (error out=w2989:errorcluster)  [unwired: 1 in, 1 out]
            n1408 = property on="btnSaveAs" class="Bool"(error in=w2989, "DisabledEnum"=w2990) -> (error out=w2986:errorcluster)  [unwired: 1 in, 1 out]
          }
          event Value Change {
            w3005 = T15."Enabled" ("Disabled")
            w3006 = FALSE ("StartMeas")
            # "No need to \"Update\" here because values are passed directly to Device(s)Settings in the case select structure."
            # "Get all the present \"Change at\" values in Instr3"
            # "Instr3 it's only available as a stand-alone instrument in some modes, and can only be a single channel instrument, so the call will only affect \"Change at\" A."
            n1409 = event-data() -> ()  [unwired: 1 in, 3 out]
            n1410 = local read "Instr3"() -> (w3000:T2)
            n1411 = Unbundle By Name(w3000) -> ("Phases.A-Change at..."=w3003:i32)
            n1412 = local read "Mode"() -> (w3007:T8)
            n1413 = case shown="3, 5, 7, 11, 13, 14" w3007 {
              tunnel: [w3011 w3014] -> w2999
              tunnel: w3003 -> [w3009 _]
              tunnel: w3002 -> [w3011 w3014]
              frame 3, 5, 7, 11, 13, 14 {
                w3010 = 0 ("Instr1.Phases.C-Change at...")
                # "Instr1 is a single one-phase AC instrument."
                n1414 = local read "Device(s)Settings"() -> (w3013:T1)
                n1415 = Bundle By Name(cluster=w3013, "Instr3.Phases.A-Change at..."=w3009, "Instr3.Phases.B-Change at..."=w3010, "Instr3.Phases.C-Change at..."=w3010) -> (w3012:T1)
                n1416 = local write "Device(s)Settings"(w3012) -> ()
              }
              frame Default {
                # "Don't update any settings, they should all be set to 0 by default in all instrumenst and modes when the event \"Mode change\" occurs."
                # "In all other modes Instr3 is DC and \"Change at\" cannot generate a change event."
              }
            }
            n1417 = property on="btnSave" class="Bool"(error in=w2999, "DisabledEnum"=w3005) -> (error out=w3004:errorcluster)  [unwired: 1 in, 1 out]
            n1418 = property on="btnSaveAs" class="Bool"(error in=w3004, "DisabledEnum"=w3005) -> (error out=w3001:errorcluster)  [unwired: 1 in, 1 out]
          }
          event Value Change {
            w3030 = T15."Enabled" ("Disabled")
            w3031 = FALSE ("StartMeas")
            # "Turn string to numeric."
            # "Check if the V range selection requires adjustments in the instrument(s) voltages."
            # "Instr1"
            # "Instr1 can override Instr2 and Instr3, and it can also have phases settings. Make voltages adjustments if needed depending on Mode."
            n1419 = event-data() -> ()  [unwired: 1 in, 1 out]
            n1420 = property on="Voltage (V)" class="Ring (strict)"(error in=w3019) -> (error out=w3025:errorcluster, "Strings []"=w3027:string[], "Value"=w3018:u16)  [unwired: 1 in, 1 out]
            n1421 = local read "Instr1"() -> (w3026:T2)
            n1422 = Index Array(array=w3027, index=w3018) -> (element=w3024:string)
            n1423 = Unbundle By Name(w3026) -> ("Vout (V)"=w3015:dbl)
            n1424 = Scan From String(format string="%f", input string=w3024, error in=w3025) -> (error out=w3017:errorcluster, output 1=w3028:dbl)  [unwired: 2 in, 2 out]
            n1425 = Less?(x=w3028, y=w3015) -> (x < y?=w3021:bool)
            n1426 = local read "Mode"() -> (w3020:T8)
            n1427 = case shown="True" w3021 {
              tunnel: w3028 -> [_ w3051]
              tunnel: w3020 -> [w3034 w3054]
              tunnel: w3018 -> [w3036 w3055]
              tunnel: [w3035 w3049] -> w3016
              tunnel: w3017 -> [w3035 w3049]
              tunnel: w3015 -> [w3033 _]
              frame False {
                # "Do nothing to adjust voltages, the value of Vout is inside the new range. Just update Device(s)Settings."
                n1428 = case shown="0..2, Default" w3034 {
                  tunnel: w3036 -> [w3038 w3042 w3046]
                  tunnel: w3033 -> [w3037 w3041 w3045]
                  frame 0..2, Default {
                    # "Instr1 overrides Instr2 and Instr3"
                    n1429 = local read "Device(s)Settings"() -> (w3039:T1)
                    n1430 = Bundle By Name(cluster=w3039, "Instr1.Vout (V)"=w3037, "Instr2.Vout (V)"=w3037, "Instr3.Vout (V)"=w3037, "Instr1.Ranges.Voltage (V)"=w3038, "Instr2.Ranges.Voltage (V)"=w3038, "Instr3.Ranges.Voltage (V)"=w3038) -> (w3040:T1)
                    n1431 = local write "Device(s)Settings"(w3040) -> ()
                  }
                  frame 3, 4, 9, 10, 13..15 {
                    # "Instr1 is a single instrument"
                    n1432 = local read "Device(s)Settings"() -> (w3044:T1)
                    n1433 = Bundle By Name(cluster=w3044, "Instr1.Vout (V)"=w3041, "Instr1.Ranges.Voltage (V)"=w3042) -> (w3043:T1)
                    n1434 = local write "Device(s)Settings"(w3043) -> ()
                  }
                  frame 5..8, 11, 12 {
                    # "Instr1 overrides Instr2 only"
                    n1435 = local read "Device(s)Settings"() -> (w3047:T1)
                    n1436 = Bundle By Name(cluster=w3047, "Instr1.Vout (V)"=w3045, "Instr2.Vout (V)"=w3045, "Instr1.Ranges.Voltage (V)"=w3046, "Instr2.Ranges.Voltage (V)"=w3046) -> (w3048:T1)
                    n1437 = local write "Device(s)Settings"(w3048) -> ()
                  }
                }
              }
              frame True {
                # "Since Vout was larger than the new range choice, by default Vout will be set to be the full new range limit to keep it as close as possible to the previous Vout level."
                # "If the new range is lower than Vout, then Vout needs to be lowered to fit inside the new range. Depending on the Mode, the phase voltages may need some adjustments to follow the Vout change too."
                n1438 = case shown="0" w3054 {
                  tunnel: w3051 -> [w3080 w3083 w3087 w3088 w3091]
                  tunnel: [w3079 w3083 w3085 w3088 w3091] -> w3053
                  tunnel: [w3079 w3083 w3085 w3088 w3090] -> w3052
                  tunnel: [w3079 w3083 0.0 ("NewVal") 0.0 ("NewVal") w3090] -> w3050
                  frame 0 {
                    # "The three phase values are equal for (L-N)"
                    n1439 = Square Root(x=3.0) -> (sqrt(x)=w3081:dbl)
                    n1440 = Divide(x=w3080, y=w3081) -> (x/y=w3079:dbl)
                  }
                  frame 1, 2 {
                    # "All three channels joined as a single output"
                  }
                  frame 5, 6 {
                    # "Two channels joined as a split phase output"
                    n1441 = Divide(x=w3087, y=2.0) -> (x/y=w3085:dbl)
                  }
                  frame 7, 8, 11, 12 {
                    # "Two channels joined as a single output"
                  }
                  frame Default {
                    w3090 = 0.0 ("NewVal")
                    # "The instrument uses only one phase/channel"
                  }
                }
                n1442 = local read "Instr1"() -> (w3056:T2)
                n1443 = Bundle By Name(cluster=w3056, "Phases.A-Volts (V)"=w3053, "Phases.B-Volts (V)"=w3052, "Phases.C-Volts (V)"=w3050, "Vout (V)"=w3051) -> (w3057:T2)
                n1444 = local write "Instr1"(w3057) -> ()
                n1445 = case shown="0..2, Default" w3054 {
                  tunnel: w3055 -> [w3062 w3065 w3072]
                  tunnel: w3053 -> [w3061 w3069 w3076]
                  tunnel: w3052 -> [w3060 w3068 w3075]
                  tunnel: w3050 -> [w3058 w3067 w3074]
                  tunnel: w3051 -> [w3059 w3066 w3073]
                  frame 0..2, Default {
                    # "Instr1 overrides Instr2 and Instr3"
                    n1446 = local read "Device(s)Settings"() -> (w3063:T1)
                    n1447 = Bundle By Name(cluster=w3063, "Instr1.Phases.A-Volts (V)"=w3061, "Instr2.Phases.A-Volts (V)"=w3061, "Instr3.Phases.A-Volts (V)"=w3061, "Instr1.Phases.B-Volts (V)"=w3060, "Instr2.Phases.B-Volts (V)"=w3060, "Instr3.Phases.B-Volts (V)"=w3060, "Instr1.Phases.C-Volts (V)"=w3058, "Instr2.Phases.C-Volts (V)"=w3058, "Instr3.Phases.C-Volts (V)"=w3058, "Instr1.Vout (V)"=w3059, "Instr2.Vout (V)"=w3059, "Instr3.Vout (V)"=w3059, "Instr1.Ranges.Voltage (V)"=w3062, "Instr2.Ranges.Voltage (V)"=w3062, "Instr3.Ranges.Voltage (V)"=w3062) -> (w3064:T1)
                    n1448 = local write "Device(s)Settings"(w3064) -> ()
                  }
                  frame 3, 4, 9, 10, 13..15 {
                    # "Instr1 is a single instrument"
                    n1449 = local read "Device(s)Settings"() -> (w3071:T1)
                    n1450 = Bundle By Name(cluster=w3071, "Instr1.Phases.A-Volts (V)"=w3069, "Instr1.Phases.B-Volts (V)"=w3068, "Instr1.Phases.C-Volts (V)"=w3067, "Instr1.Vout (V)"=w3066, "Instr1.Ranges.Voltage (V)"=w3065) -> (w3070:T1)
                    n1451 = local write "Device(s)Settings"(w3070) -> ()
                  }
                  frame 5..8, 11, 12 {
                    # "Instr1 overrides Instr2 only"
                    n1452 = local read "Device(s)Settings"() -> (w3077:T1)
                    n1453 = Bundle By Name(cluster=w3077, "Instr1.Phases.A-Volts (V)"=w3076, "Instr2.Phases.A-Volts (V)"=w3076, "Instr1.Phases.B-Volts (V)"=w3075, "Instr2.Phases.B-Volts (V)"=w3075, "Instr1.Phases.C-Volts (V)"=w3074, "Instr2.Phases.C-Volts (V)"=w3074, "Instr1.Vout (V)"=w3073, "Instr2.Vout (V)"=w3073, "Instr1.Ranges.Voltage (V)"=w3072, "Instr2.Ranges.Voltage (V)"=w3072) -> (w3078:T1)
                    n1454 = local write "Device(s)Settings"(w3078) -> ()
                  }
                }
              }
            }
            n1455 = property on="btnSaveAs" class="Bool"(error in=w3016, "DisabledEnum"=w3030) -> (error out=w3023:errorcluster)  [unwired: 1 in, 1 out]
            n1456 = property on="btnSave" class="Bool"(error in=w3023, "DisabledEnum"=w3030) -> (error out=w3022:errorcluster)  [unwired: 1 in, 1 out]
          }
          event Value Change {
            w3106 = T15."Enabled" ("Disabled")
            w3107 = FALSE ("StartMeas")
            # "No need to \"Update\" because Device(s)Settings were already set inside the case structure."
            # "Turn string to numeric."
            # "Check if the V range selection requires adjustments in the instrument voltage."
            # "Instr2"
            # "Instr2 can only exist as a single phase/channel affecting only itself. So, in which Mode, is irrelevant. Only its own settings need to be adjusted."
            n1457 = event-data() -> ()  [unwired: 1 in, 1 out]
            n1458 = property on="Voltage (V)" class="Ring (strict)"(error in=w3096) -> (error out=w3101:errorcluster, "Strings []"=w3103:string[], "Value"=w3095:u16)  [unwired: 1 in, 1 out]
            n1459 = Index Array(array=w3103, index=w3095) -> (element=w3100:string)
            n1460 = local read "Instr2"() -> (w3102:T2)
            n1461 = Unbundle By Name(w3102) -> ("Vout (V)"=w3092:dbl)
            n1462 = Scan From String(format string="%f", input string=w3100, error in=w3101) -> (error out=w3094:errorcluster, output 1=w3104:dbl)  [unwired: 2 in, 2 out]
            n1463 = Less?(x=w3104, y=w3092) -> (x < y?=w3097:bool)
            n1464 = case shown="True" w3097 {
              tunnel: w3104 -> [_ w3115]
              tunnel: w3095 -> [w3113 w3114]
              tunnel: [w3112 w3118] -> w3093
              tunnel: w3094 -> [w3112 w3118]
              tunnel: w3092 -> [w3109 _]
              frame False {
                # "Do nothing to adjust Vout because it's still inside the new range. Just update Device(s)Settings."
                n1465 = local read "Device(s)Settings"() -> (w3111:T1)
                n1466 = Bundle By Name(cluster=w3111, "Instr2.Vout (V)"=w3109, "Instr2.Ranges.Voltage (V)"=w3113) -> (w3110:T1)
                n1467 = local write "Device(s)Settings"(w3110) -> ()
              }
              frame True {
                # "Since Vout was larger than the new range choice, by default Vout will be set to be the full new range limit to keep it as close as possible to the previous Vout level."
                # "If the new range is lower than Vout, then Vout needs to be lowered to fit inside the new range."
                n1468 = local read "Device(s)Settings"() -> (w3117:T1)
                n1469 = Bundle By Name(cluster=w3117, "Instr2.Vout (V)"=w3115, "Instr2.Ranges.Voltage (V)"=w3114) -> (w3116:T1)
                n1470 = local read "Instr2"() -> (w3119:T2)
                n1471 = Bundle By Name(cluster=w3119, "Vout (V)"=w3115) -> (w3120:T2)
                n1472 = local write "Instr2"(w3120) -> ()
                n1473 = local write "Device(s)Settings"(w3116) -> ()
              }
            }
            n1474 = property on="btnSaveAs" class="Bool"(error in=w3093, "DisabledEnum"=w3106) -> (error out=w3099:errorcluster)  [unwired: 1 in, 1 out]
            n1475 = property on="btnSave" class="Bool"(error in=w3099, "DisabledEnum"=w3106) -> (error out=w3098:errorcluster)  [unwired: 1 in, 1 out]
          }
          event Value Change {
            w3135 = T15."Enabled" ("Disabled")
            w3136 = FALSE ("StartMeas")
            # "No need to \"Update\" because Device(s)Settings were already set inside the case structure."
            # "Turn string to numeric."
            # "Check if the V range selection requires adjustments in the instrument voltage."
            # "Instr3"
            # "Instr3 can only exist as a single phase/channel affecting only itself. So, in which Mode, is irrelevant. Only its own settings need to be adjusted."
            n1476 = event-data() -> ()  [unwired: 1 in, 1 out]
            n1477 = property on="Voltage (V)" class="Ring (strict)"(error in=w3125) -> (error out=w3130:errorcluster, "Strings []"=w3132:string[], "Value"=w3124:u16)  [unwired: 1 in, 1 out]
            n1478 = Index Array(array=w3132, index=w3124) -> (element=w3129:string)
            n1479 = local read "Instr3"() -> (w3131:T2)
            n1480 = Unbundle By Name(w3131) -> ("Vout (V)"=w3121:dbl)
            n1481 = Scan From String(format string="%f", input string=w3129, error in=w3130) -> (error out=w3123:errorcluster, output 1=w3133:dbl)  [unwired: 2 in, 2 out]
            n1482 = Less?(x=w3133, y=w3121) -> (x < y?=w3126:bool)
            n1483 = case shown="True" w3126 {
              tunnel: w3133 -> [_ w3144]
              tunnel: w3124 -> [w3142 w3143]
              tunnel: [w3141 w3147] -> w3122
              tunnel: w3123 -> [w3141 w3147]
              tunnel: w3121 -> [w3138 _]
              frame False {
                # "Do nothing to adjust Vout because it's still inside the new range. Just update Device(s)Settings."
                n1484 = local read "Device(s)Settings"() -> (w3140:T1)
                n1485 = Bundle By Name(cluster=w3140, "Instr3.Vout (V)"=w3138, "Instr3.Ranges.Voltage (V)"=w3142) -> (w3139:T1)
                n1486 = local write "Device(s)Settings"(w3139) -> ()
              }
              frame True {
                # "Since Vout was larger than the new range choice, by default Vout will be set to be the full new range limit to keep it as close as possible to the previous Vout level."
                # "If the new range is lower than Vout, then Vout needs to be lowered to fit inside the new range."
                n1487 = local read "Device(s)Settings"() -> (w3146:T1)
                n1488 = Bundle By Name(cluster=w3146, "Instr3.Vout (V)"=w3144, "Instr3.Ranges.Voltage (V)"=w3143) -> (w3145:T1)
                n1489 = local read "Instr3"() -> (w3148:T2)
                n1490 = Bundle By Name(cluster=w3148, "Vout (V)"=w3144) -> (w3149:T2)
                n1491 = local write "Instr3"(w3149) -> ()
                n1492 = local write "Device(s)Settings"(w3145) -> ()
              }
            }
            n1493 = property on="btnSaveAs" class="Bool"(error in=w3122, "DisabledEnum"=w3135) -> (error out=w3128:errorcluster)  [unwired: 1 in, 1 out]
            n1494 = property on="btnSave" class="Bool"(error in=w3128, "DisabledEnum"=w3135) -> (error out=w3127:errorcluster)  [unwired: 1 in, 1 out]
          }
          event Value Change {
            w3157 = T15."Enabled" ("Disabled")
            w3158 = FALSE ("StartMeas")
            # "Since the current range in the device is dependent on the number of chassis presently turned on in the grid emulator, there's a possibility that the range limits that could have been saved in a recently-loaded configuration file do not match the present state of the grid emulator. To ensure that the present current range limits are correct in case that the user wants to save the present configuration, the list of options that the current range controls show need to be updated to the actual number of chassis turned on in the emulator. Then those values can be passed to Device(s)Settings to be saved."
            # "Update Device(s)Settings"
            # "If any current range control is changed in any instrument, update the list of options that the controls show."
            n1495 = event-data() -> ()  [unwired: 1 in, 6 out]
            n1496 = flat-sequence {
              tunnel: w3152 -> [w3167]
              tunnel: [w3160] -> w3151
              frame #0 {
                # "2"
                # "1"
                # "3"
                # "Refresh the 'Strings[]' array property for the current range control of each instrument."
                # "Instr3"
                # "Instr2"
                # "Instr1"
                # "The frame is to make sure that all data has been updated in the instruments controls before passing the values to the Device(s)Settings cluster."
                n1497 = local read "Chassis"() -> (w3172:i32)
                n1498 = local read "Mode"() -> (w3173:T8)
                n1499 = Multiply(x=w3172, y=6) -> (x*y=w3169:i32)
                n1500 = Multiply(x=30, y=w3172) -> (x*y=w3168:i32)
                n1501 = case shown="Default" w3173 {
                  tunnel: w3169 -> [w3182 w3187 w3201]
                  tunnel: w3168 -> [w3179 w3184 w3200]
                  tunnel: [w3176 w3190 w3197] -> w3166
                  tunnel: [w3175 w3189 w3199] -> w3165
                  tunnel: [w3175 w3189 w3199] -> w3163
                  tunnel: [w3175 w3189 w3198] -> w3161
                  tunnel: w3167 -> [w3174 w3183 w3195]
                  frame Default {
                    w3180 = "%d" ("format string")
                    # "All other modes have the same current range limits regardless of instrument configuration."
                    n1502 = Format Into String(format string=w3180, error in=w3174, w3182) -> (resulting string=w3178:string, error out=w3181:errorcluster)  [unwired: 1 in]
                    n1503 = Format Into String(format string=w3180, error in=w3181, w3179) -> (resulting string=w3177:string, error out=w3176:errorcluster)  [unwired: 1 in]
                    n1504 = Build Array(w3178, w3177) -> (w3175:string[])
                  }
                  frame 1, 2 {
                    w3185 = 3 ("y")
                    w3193 = "%d" ("format string")
                    # "Three single AC or three single DC instruments"
                    n1505 = Multiply(x=w3187, y=w3185) -> (x*y=w3188:i32)
                    n1506 = Multiply(x=w3185, y=w3184) -> (x*y=w3186:i32)
                    n1507 = Format Into String(format string=w3193, error in=w3183, w3188) -> (resulting string=w3192:string, error out=w3194:errorcluster)  [unwired: 1 in]
                    n1508 = Format Into String(format string=w3193, error in=w3194, w3186) -> (resulting string=w3191:string, error out=w3190:errorcluster)  [unwired: 1 in]
                    n1509 = Build Array(w3192, w3191) -> (w3189:string[])
                  }
                  frame 7, 8, 11, 12 {
                    w3202 = "%d" ("format string")
                    w3206 = 2 ("y")
                    # "One double AC or DC, and a third singe AC or DC"
                    n1510 = Format Into String(format string=w3202, error in=w3195, w3201) -> (resulting string=w3204:string, error out=w3205:errorcluster)  [unwired: 1 in]
                    n1511 = Format Into String(format string=w3202, error in=w3205, w3200) -> (resulting string=w3203:string, error out=w3196:errorcluster)  [unwired: 1 in]
                    n1512 = Multiply(x=w3201, y=w3206) -> (x*y=w3208:i32)
                    n1513 = Multiply(x=w3206, y=w3200) -> (x*y=w3207:i32)
                    n1514 = Build Array(w3204, w3203) -> (w3198:string[])
                    n1515 = Format Into String(format string=w3202, error in=w3196, w3208) -> (resulting string=w3210:string, error out=w3211:errorcluster)  [unwired: 1 in]
                    n1516 = Format Into String(format string=w3202, error in=w3211, w3207) -> (resulting string=w3209:string, error out=w3197:errorcluster)  [unwired: 1 in]
                    n1517 = Build Array(w3210, w3209) -> (w3199:string[])
                  }
                }
                n1518 = property on="Current (A)" class="Ring (strict)"(error in=w3166, "Strings []"=w3165) -> (error out=w3164:errorcluster)  [unwired: 1 in, 1 out]
                n1519 = property on="Current (A)" class="Ring (strict)"(error in=w3164, "Strings []"=w3163) -> (error out=w3162:errorcluster)  [unwired: 1 in, 1 out]
                n1520 = property on="Current (A)" class="Ring (strict)"(error in=w3162, "Strings []"=w3161) -> (error out=w3160:errorcluster)  [unwired: 1 in, 1 out]
              }
            }
            n1521 = property on="Update" class="Bool (strict)"(error in=w3151) -> (error out=w3156:errorcluster, "Value"=w3150:bool)  [unwired: 1 in, 1 out]
            n1522 = property on="Update" class="Bool (strict)"(error in=w3156, "Val(Sgnl)"=w3150) -> (error out=w3153:errorcluster)  [unwired: 1 in, 1 out]
            n1523 = property on="btnSaveAs" class="Bool"(error in=w3153, "DisabledEnum"=w3157) -> (error out=w3154:errorcluster)  [unwired: 1 in, 1 out]
            n1524 = property on="btnSave" class="Bool"(error in=w3154, "DisabledEnum"=w3157) -> (error out=w3155:errorcluster)  [unwired: 1 in, 1 out]
          }
          event Value Change {
            w3220 = T15."Enabled" ("Disabled")
            w3221 = FALSE ("StartMeas")
            # "Wave Shapes are only enabled when the instrument is AC. That has been taken care in the \"WaveEnable\" case of the \"Mode Change\" event."
            # "No need to \"Update\" here because values are passed directly to Device(s)Settings in the case select structure."
            # "Since Instr1 exists in all modes and it may override Instr2 and Instr3 in some of them, evaluate what to do with Wave Shape changes depending on Mode."
            n1525 = event-data() -> ()  [unwired: 1 in, 6 out]
            n1526 = local read "Instr1"() -> (w3217:T2)
            n1527 = Unbundle By Name(w3217) -> ("Phases.A-Wave Shape"=w3216:u16, "Phases.B-Wave Shape"=w3215:u16, "Phases.C-Wave Shape"=w3212:u16)
            n1528 = local read "Mode"() -> (w3222:T8)
            n1529 = case shown="3, 4, 9, 10, 13..15" w3222 {
              tunnel: w3216 -> [w3227 w3233 w3239]
              tunnel: w3215 -> [w3225 w3231 w3237]
              tunnel: [w3226 w3232 w3238] -> w3213
              tunnel: w3214 -> [w3226 w3232 w3238]
              tunnel: [w3224 w3230 w3236] -> _
              tunnel: w3212 -> [w3224 w3230 w3236]
              frame 0..2, Default {
                # "Instr1 overrides Instr2 and Instr3"
                n1530 = local read "Device(s)Settings"() -> (w3229:T1)
                n1531 = Bundle By Name(cluster=w3229, "Instr1.Phases.A-Wave Shape"=w3227, "Instr2.Phases.A-Wave Shape"=w3227, "Instr3.Phases.A-Wave Shape"=w3227, "Instr1.Phases.B-Wave Shape"=w3225, "Instr2.Phases.B-Wave Shape"=w3225, "Instr3.Phases.B-Wave Shape"=w3225, "Instr1.Phases.C-Wave Shape"=w3224, "Instr2.Phases.C-Wave Shape"=w3224, "Instr3.Phases.C-Wave Shape"=w3224) -> (w3228:T1)
                n1532 = local write "Device(s)Settings"(w3228) -> ()
              }
              frame 5..8, 11, 12 {
                # "Instr1 overrides Instr2 only"
                n1533 = local read "Device(s)Settings"() -> (w3235:T1)
                n1534 = Bundle By Name(cluster=w3235, "Instr1.Phases.A-Wave Shape"=w3233, "Instr2.Phases.A-Wave Shape"=w3233, "Instr1.Phases.B-Wave Shape"=w3231, "Instr2.Phases.B-Wave Shape"=w3231, "Instr1.Phases.C-Wave Shape"=w3230, "Instr2.Phases.C-Wave Shape"=w3230) -> (w3234:T1)
                n1535 = local write "Device(s)Settings"(w3234) -> ()
              }
              frame 3, 4, 9, 10, 13..15 {
                # "Instr1 is a single instrument by itself"
                n1536 = local read "Device(s)Settings"() -> (w3241:T1)
                n1537 = Bundle By Name(cluster=w3241, "Instr1.Phases.A-Wave Shape"=w3239, "Instr1.Phases.B-Wave Shape"=w3237, "Instr1.Phases.C-Wave Shape"=w3236) -> (w3240:T1)
                n1538 = local write "Device(s)Settings"(w3240) -> ()
              }
            }
            n1539 = property on="btnSave" class="Bool"(error in=w3213, "DisabledEnum"=w3220) -> (error out=w3219:errorcluster)  [unwired: 1 in, 1 out]
            n1540 = property on="btnSaveAs" class="Bool"(error in=w3219, "DisabledEnum"=w3220) -> (error out=w3218:errorcluster)  [unwired: 1 in, 1 out]
          }
          event Value Change {
            w3250 = T15."Enabled" ("Disabled")
            w3251 = FALSE ("StartMeas")
            # "Wave Shapes are only enabled when the instrument is AC. That has been taken care in the \"WaveEnable\" case of the \"Mode Change\" event."
            # "No need to \"Update\" here because values are passed directly to Device(s)Settings in the case select structure."
            # "Instr2 can only exist as itself in a few modes to be able to change its Wave Shapes."
            n1541 = event-data() -> ()  [unwired: 1 in, 6 out]
            n1542 = local read "Instr2"() -> (w3247:T2)
            n1543 = Unbundle By Name(w3247) -> ("Phases.A-Wave Shape"=w3246:u16, "Phases.B-Wave Shape"=w3245:u16, "Phases.C-Wave Shape"=w3242:u16)
            n1544 = local read "Mode"() -> (w3252:T8)
            n1545 = case shown="3, 4, 9, 10, 13..15" w3252 {
              tunnel: w3246 -> [_ w3259]
              tunnel: w3245 -> [_ w3257]
              tunnel: [w3255 w3258] -> w3243
              tunnel: w3244 -> [w3255 w3258]
              tunnel: [w3254 w3256] -> _
              tunnel: w3242 -> [w3254 w3256]
              frame Default {
                # "Instr2 is unavailable in the other modes."
              }
              frame 3, 4, 9, 10, 13..15 {
                # "Modes in which Instr2 can be accessed by the user as a single instrument."
                n1546 = local read "Device(s)Settings"() -> (w3261:T1)
                n1547 = Bundle By Name(cluster=w3261, "Instr2.Phases.A-Wave Shape"=w3259, "Instr2.Phases.B-Wave Shape"=w3257, "Instr2.Phases.C-Wave Shape"=w3256) -> (w3260:T1)
                n1548 = local write "Device(s)Settings"(w3260) -> ()
              }
            }
            n1549 = property on="btnSave" class="Bool"(error in=w3243, "DisabledEnum"=w3250) -> (error out=w3249:errorcluster)  [unwired: 1 in, 1 out]
            n1550 = property on="btnSaveAs" class="Bool"(error in=w3249, "DisabledEnum"=w3250) -> (error out=w3248:errorcluster)  [unwired: 1 in, 1 out]
          }
          event Value Change {
            w3270 = T15."Enabled" ("Disabled")
            w3271 = FALSE ("StartMeas")
            # "Wave Shapes are only enabled when the instrument is AC. That has been taken care in the \"WaveEnable\" case of the \"Mode Change\" event."
            # "No need to \"Update\" here because values are passed directly to Device(s)Settings in the case select structure."
            # "Instr3 can only exist as itself in a few modes to be able to change its Wave Shapes."
            n1551 = event-data() -> ()  [unwired: 1 in, 6 out]
            n1552 = local read "Instr3"() -> (w3267:T2)
            n1553 = Unbundle By Name(w3267) -> ("Phases.A-Wave Shape"=w3266:u16, "Phases.B-Wave Shape"=w3265:u16, "Phases.C-Wave Shape"=w3262:u16)
            n1554 = local read "Mode"() -> (w3272:T8)
            n1555 = case shown="3..15" w3272 {
              tunnel: w3266 -> [_ w3279]
              tunnel: w3265 -> [_ w3277]
              tunnel: [w3275 w3278] -> w3263
              tunnel: w3264 -> [w3275 w3278]
              tunnel: [w3274 w3276] -> _
              tunnel: w3262 -> [w3274 w3276]
              frame Default {
                # "Instr3 is unavailable in the other modes."
              }
              frame 3..15 {
                # "Modes in which Instr3 can be accessed by the user as a single instrument."
                n1556 = local read "Device(s)Settings"() -> (w3281:T1)
                n1557 = Bundle By Name(cluster=w3281, "Instr3.Phases.A-Wave Shape"=w3279, "Instr3.Phases.B-Wave Shape"=w3277, "Instr3.Phases.C-Wave Shape"=w3276) -> (w3280:T1)
                n1558 = local write "Device(s)Settings"(w3280) -> ()
              }
            }
            n1559 = property on="btnSave" class="Bool"(error in=w3263, "DisabledEnum"=w3270) -> (error out=w3269:errorcluster)  [unwired: 1 in, 1 out]
            n1560 = property on="btnSaveAs" class="Bool"(error in=w3269, "DisabledEnum"=w3270) -> (error out=w3268:errorcluster)  [unwired: 1 in, 1 out]
          }
        }
        n1561 = Or(x=w412, y=w413) -> (x .or. y?=w414:bool)
      }
      "Changed" <- w19
      "Save As" <- w13
      n1562 = call <vilib>:"Clear Errors.vi"("error in (no error)"=w9) -> ("error out"=w8:errorcluster)  [unwired: 5 in, 1 out]
      n1563 = property class="VI"(error in=w8, "FP.Behavior"=T11."Default" ("Front Panel Window:Behavior")) -> (error out=w17:errorcluster)  [unwired: 1 in, 1 out]
      n1564 = property class="VI"(error in=w17, "FP.State"=T12."Closed" ("Front Panel Window:State")) -> ()  [unwired: 1 in, 2 out]
    }
    frame Error {
    }
  }
  "MyPluginsBase out" <- w3
  "error out" <- w2
